vi "Main UI.vi"() -> (3 "CH Name":string[](array[string]))   [LabVIEW 2017]
uses:
  Controls/Load Bank.ctl
  Controls/Available Tests.ctl
  Controls/Graphic Display.ctl
  Controls/Auto Test Display.ctl
  Console Sim/Controls/Console Select.ctl
  Controls/Test TypeDef.ctl
  Code Library/Queue References Array.ctl
  Code Library/Queue Element.ctl
  Controls/Snapshot Typedef.ctl
  Controls/FanMode.ctl
  Controls/LPCA Commands.ctl
  <vilib>/DAQmx/write.llb/DAQmx Write (Analog DBL 1Chan 1Samp).vi
  <vilib>/DAQmx/write.llb/DAQmx Write (Analog Wfm 1Chan NSamp).vi
  <vilib>/DAQmx/write.llb/DAQmx Write (Digital Bool 1Line 1Point).vi
  <vilib>/Utility/config.llb/Read Key (String).vi
  <vilib>/DAQmx/miscellaneous.llb/DAQmx Fill In Error Info.vi
  <vilib>/Utility/config.llb/Write Key (String).vi
  <vilib>/Utility/config.llb/NI_LVConfig.lvlib
  <vilib>/measure/NI_MABase.lvlib
  <resource>/objmgr/daqmx.rc
panel:
  in  "Console Select":T1=enum."SCL Torque"
  in  "Load Config":bool
  in  "Save Config":bool
  in  "SS#":u16
  in  "Snapshot":bool
  in  "Path":path=path "<Data File Path>"
  in  "Test Details":string="<Test Details>"
  out "Test Description":string="<Select Test for a Description>"
  in  "Available Tests":T2
  out "Version":string
  out "Over Temp":bool
  in  "LPCA COM":refnum<visa-resource-name>="COM3"
  in  "Targets":enum32{"Page 1"}(tab)
  in  "Auto Pulse":bool
  in  "Range":i32=2 min=0 max=2 step=1
  in  "Spin":bool
  in  "Load Bank":T3 caption="L/B"
  in  "RPM Target":i32 caption="RPM" min=0 max=250 step=1
  in  "Ibrake":i32=1 caption="MAMP" min=0 max=2500 step=1
  in  "Step Height":i32=2 caption="Ramp" min=1 max=5 step=1
  in  "Thermal Limits":enum32{"Page 1"}(tab)
  in  "S Period":dbl=1.0 min=0.0 max=1440.0 step=0.1 format="%#_g min"
  in  "Thermal Limit":i32=200 min=25 max=250 step=1 format="%.0f degC"
  in  "Thermal Resume":i32=5 min=0 max=250 step=1 format="%.0f degC"
  in  "Stop Time":dbl=60.0 min=1.0 max=1440.0 step=1.0 format="%#_g min"
  in  "Thermal Equilibrium":bool caption="Thermal\nEquilibrium"
  out "Graphic Display":T4
  in  "Data Display":u16(ring) items=["CH.Name", "CH.Name", "CH.Name", "Ibrake", "CH.Name", "CH.Name", "CH.Name", "CH.Name", "CH.Name", "CH.Name", "CH.Name", "CH.Name", "CH.Name", "CH.Name", "Torque", "Ambent", "Brake", "CH.Name", "CH.Name", "CH.Name", "CH.Name", "CH.Name", "CH.Name", "CH.Name", "CH.Name", "CH.Name", "CH.Name"]
  out "Reading Graph":waveform(dbl)(graph)
  out "RPM Graph":cluster{"X":dbl, "Y":dbl}[](graph)
  out "CH Value":dbl[](array[numeric]) format="%.2f"
  in  "Data Setup":i32[](listbox)
  out "RPM":cluster{dbl, dbl}(knob) scale=0.0..300.0
  out "Torque (in-lb)":dbl(knob) scale=-2000.0..2000.0 scale format="%.2f"
  out "Auto Test Controls":T5
  in  "FanMode":bool
  out "Capture":bool
  in  "Stop Test":bool
  in  "Start Test":bool
  in  "Pause Test":bool
  in  "Load Sweep":string
  in  "RPM Sweep":string
  in  "Ibrake Sweep":string
  in  "Sample Frequency":dbl=60.0 min=1.0 max=60.0 step=1.0 format="%.0f S/min"
  in  "Filters":T6(ring)
  out "Sample":bool
  in  "Step Height Sweep":string
  in  "Range Sweep":string
  out "Fan Mode LED Array":bool[](array[boolean])=[FALSE, TRUE, FALSE]
  in  "Save Pulse Data":bool
  in  "Start Pulse":bool
  in  "Pulse Frequency":dbl
  in  "Amplitude":dbl
  in  "Average RPM":dbl
  out "Waveform Graph":waveform(dbl)(graph)
  out "Test Status":string
  out "Test:":string
  out "Time Stamp Control":timestamp format="%<%H:%M:%S  %d/%m/%Y>T"
  # "Targets"
  # "Stop Conditions"
  # "Auto Test Controls"
  # "Swept Targets"
  # "On       Off      Auto"
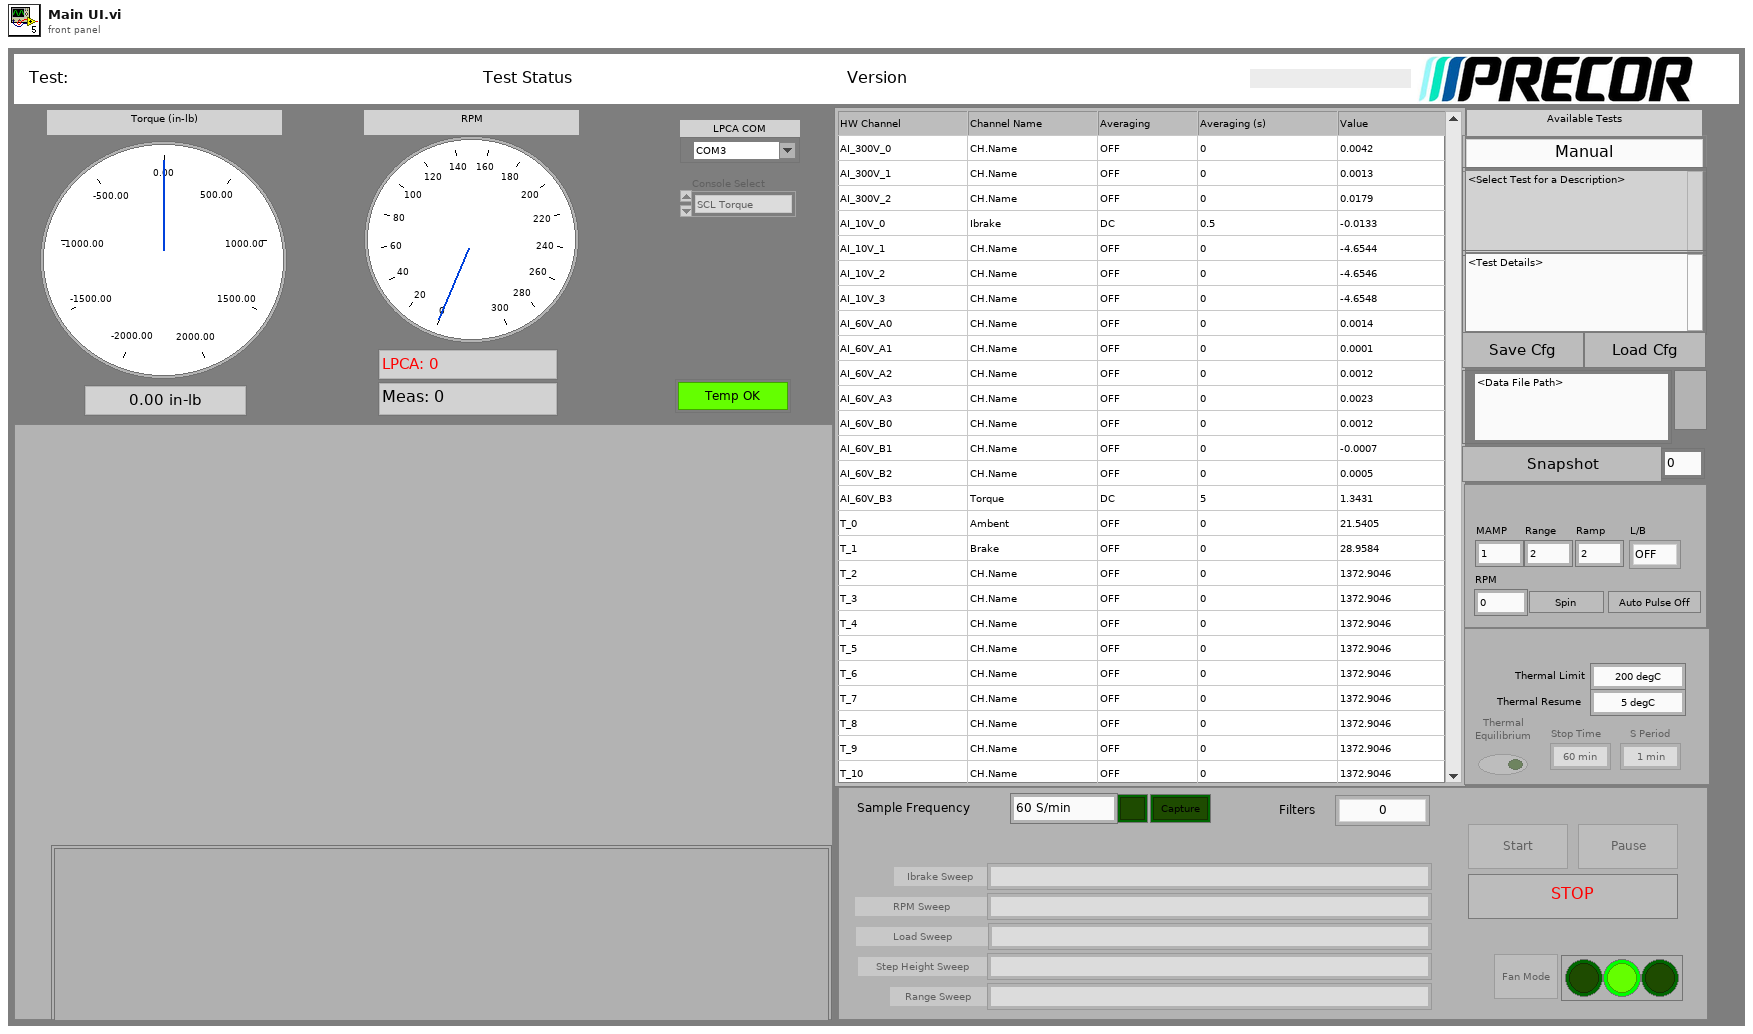
[diagram p1: front panel]
types:
  T1 = typedef "Console Select.ctl" = enum16{"P31 EFX800", "AMT", "SCL Torque"}
  T2 = typedef "Available Tests.ctl" = enum16{"Manual", "EFX Brake Torque", "Generator Torque", "EFX Brake Thermal", "Generator Thermal", "Pulsed RPM", "AMT Brake Torque", "Bike Brake Torque", "AMT Brake Thermal", "Bike Brake Thermal"}
  T3 = typedef "Load Bank.ctl" = enum16{"OFF", "50", "25", "16.7", "12.5", "10.0", "8.3", "7.1", "6.3", "5.6", "5.0", "4.5", "4.2", "3.8", "3.6", "3.3", "3.1"}
  T4 = typedef "Graphic Display.ctl" = enum32{"Analize", "Pulse", "Hidden"}
  T5 = typedef "Auto Test Display.ctl" = enum32{"Sweep Targes", "Pulse", "Hidden"}
  T6 = enum16{"0", "0.1", "0.2", "0.5", "1", "2", "5", "10", "20", "50", "100", "200", "500", "1000", "2000", "5000", "10000"}
  T7 = typedef "Test TypeDef.ctl" = cluster{"Queue Array":T8, "Queue Element":T9, "System Event":refnum<user-event>, "System Event RefNum":refnum<event-registration>, "Queue List":string[], "LPCA COM":refnum<visa-resource-name>, "Rotating":bool, "PrecorAI":refnum<k21>, "T_0 Index":i32, "Bar Graph X":i32[], "Channels":string[], "Active Indicies":i32[], "Active Channels":string[][], "Sample Frequency":dbl, "Ibrake Sweep":string[], "RPM Sweep":string[], "Load Sweep":string[], "Step Height Sweep":string[], "Range Sweep":string[], "A Counter":i32, "B Counter":i32, "C Counter":i32, "#A":i32, "#B":i32, "#C":i32, "Current RPM":dbl, "Current Ibrake":u32, "Current Range":u32, "Current Step Height":u32, "Load Bank":T3, "Cfg Cntrls":refnum<vi>[], "T_Monitor Indices":i32[], "Thermal Limit":i32, "Thermal Resume":i32, "Timer Reset":bool, "Stop Time":dbl, "Autotest":bool, "Pulsed RPM Capture":bool, "Get Sample":bool, "Last State":string, "Reset Timeout":bool, "Ctrl Refs":cluster{"Test Details":refnum<vi>, "Save Config":refnum<vi>, "Load Config":refnum<vi>, "Path":refnum<vi>, "Snapshot":refnum<vi>, "SS#":refnum<vi>, "Ibrake":refnum<vi>, "RPM Target":refnum<vi>, "Spin":refnum<vi>, "Load Bank":refnum<vi>, "Start Test":refnum<vi>, "Pause Test":refnum<vi>, "Load Sweep":refnum<vi>, "RPM Sweep":refnum<vi>, "Ibrake Sweep":refnum<vi>, "Filters":refnum<vi>, "Sample Frequency":refnum<vi>, "Data Setup":refnum<vi>, "Pause":refnum<vi>, "Stop Time":refnum<vi>, "S Period":refnum<vi>, "Range":refnum<vi>, "Step Height":refnum<vi>, "Step Height Sweep":refnum<vi>, "Range Sweep":refnum<vi>, "Available Tests":refnum<vi>, "RPM Graph":refnum<vi>, "RPM Knob":refnum<vi>, "FanMode":refnum<vi>, "Fan Mode LED Array":refnum<vi>, "Thermal Equilibrium":refnum<vi>, "Data Display":refnum<vi>, "LPCA Error":refnum<vi>, "LPCA Ramp":refnum<vi>, "LPCA Range":refnum<vi>, "LPCA Resistance":refnum<vi>, "Analyze Read":refnum<vi>, "Console Select":refnum<vi>, "Sub Panel":refnum<vi>}, "Pulse Waveform":waveform(dbl), "Snapshot":T10, "Sample Period":dbl, "OverTemp":bool, "Available Tests":T2, "FanMode":T11, "Fan Mode LED Array":bool[], "Thermal\nEquilibrium ":bool, "Equilibrium Stop":bool, "AvgDegChg":dbl[]}
  T8 = typedef "Queue References Array.ctl" = refnum<queue>[]
  T9 = typedef "Queue Element.ctl" = cluster{"state":string, "data":variant}
  T10 = typedef "Snapshot Typedef.ctl" = cluster{"Test Details":string, "Version":string, "Date":timestamp, "Selected Test":string, "Snapshot Number":u16, "Time":timestamp, "Ibrake Setpoint":string, "RPM Setpoint":string, "Range Setpoint":string, "Step Height Setpoint":string, "Load Bank Setpoint":string, "Measurement Headers":string, "Measurements":string, "A":i32, "B":i32, "C":i32, "Raw Data":string[][], "Available Tests":T2, "Ibrake List":string, "RPM List":string, "Load Bank List":string, "Range List":string, "Step Height List":string, "FanMode Setpoint":T11}
  T11 = typedef "FanMode.ctl" = enum16{"On", "Off", "Auto"}
  T12 = cluster{"Test Details":refnum<vi>, "Save Config":refnum<vi>, "Load Config":refnum<vi>, "Path":refnum<vi>, "Snapshot":refnum<vi>, "SS#":refnum<vi>, "Ibrake":refnum<vi>, "RPM Target":refnum<vi>, "Spin":refnum<vi>, "Load Bank":refnum<vi>, "Start Test":refnum<vi>, "Pause Test":refnum<vi>, "Load Sweep":refnum<vi>, "RPM Sweep":refnum<vi>, "Ibrake Sweep":refnum<vi>, "Filters":refnum<vi>, "Sample Frequency":refnum<vi>, "Data Setup":refnum<vi>, "Pause":refnum<vi>, "Stop Time":refnum<vi>, "S Period":refnum<vi>, "Range":refnum<vi>, "Step Height":refnum<vi>, "Step Height Sweep":refnum<vi>, "Range Sweep":refnum<vi>, "Available Tests":refnum<vi>, "RPM Graph":refnum<vi>, "RPM Knob":refnum<vi>, "FanMode":refnum<vi>, "Fan Mode LED Array":refnum<vi>, "Thermal Equilibrium":refnum<vi>, "Data Display":refnum<vi>, "LPCA Error":refnum<vi>, "LPCA Ramp":refnum<vi>, "LPCA Range":refnum<vi>, "LPCA Resistance":refnum<vi>, "Analyze Read":refnum<vi>, "Console Select":refnum<vi>, "Sub Panel":refnum<vi>}
  T13 = typedef "lveventtype.ctl" = enum32{"Null", "Timeout", "Annotation Menu Selection", "Annotation Menu Selection?", "App Instance Close", "App Instance Close?", "Autoscale Range Change", "Bookmark Info Change", "Cell Edit", "Cell Edit?", "Cursor Grab", "Cursor Grab?", "Cursor Menu Selection", "Cursor Menu Selection?", "Cursor Move", "Cursor Release", "Data Change", "Direction Change", "Display State Change", "Drag Ended", "Drag Enter", "Drag Leave", "Drag Over", "Drag Source Update", "Drag Starting", "Drag Starting?", "Drop", "Exec State Change", "Key Down", "Key Down?", "Key Repeat", "Key Repeat?", "Key Up", "Listbox Double Click", "Menu Activation?", "Menu Selection (App)", "Menu Selection? (App)", "Menu Selection (User)", "Mouse Down", "Mouse Down?", "Mouse Enter", "Mouse Leave", "Mouse Move", "Mouse Up", "Mouse Wheel", "NI Security User Change (App)", "Pane Size", "Panel Close", "Panel Close?", "Panel Resize", "Plot Attribute Change", "Scale Range Change", "Shortcut Menu Activation?", "Shortcut Menu Selection (App)", "Shortcut Menu Selection? (App)", "Shortcut Menu Selection (User)", "Tree Double Click", "Tree Drag", "Tree Drag?", "Tree Drop", "Tree Drop?", "Tree Item Close", "Tree Item Close?", "Tree Item Open", "Tree Item Open?", "User Event", "Value Change"}
  T14 = typedef "LVPoint32TypeDef.ctl" = cluster{"Horizontal":i32, "Vertical":i32}
  T15 = typedef "LVRowAndColumnTypeDef.ctl" = cluster{"Row":i32, "Column":i32}
  T16 = cluster{"Label.Text":string, "selected path":path}
  T17 = cluster{"ItemTag":string, "Row":i32, "Column":i32}
  T18 = cluster{"String":string, "Row":i32, "Column":i32}
  T19 = typedef "NI_LVConfig.lvlib/Config Data RefNum.ctl" = refnum<k1>
  T20 = typedef "LPCA Commands.ctl" = enum16{"RSET", "stop", "rpmh", "rpml", "prpm", "rpm", "mamp", "rng", "tmp1", "tmp2", "err", "ramp"}
  T21 = enum16{"Init", "Get", "Set Step Counter", "Insert Command", "Insert Now Command"}
  T22 = cluster{"A Counter":i32, "B Counter":i32, "C Counter":i32}
  T23 = cluster{"ItemNames":string[][], "ItemSyms":i32[]}
  T24 = enum8{"Enabled", "Disabled", "Disabled and Grayed Out"}
  T25 = cluster{"A Counter":i32, "B Counter":i32, "B Counter 2":i32}
  T26 = cluster{"seconds since 1Jan1904":timestamp, "SS#":u16, "Snapshot":bool}
  T27 = cluster{"Sample Acquired":bool, "Torque":dbl, "Temperatre Plot Data":cluster{dbl[], i32[]}[], "Temperature Avg":dbl[], "Samples":i32}
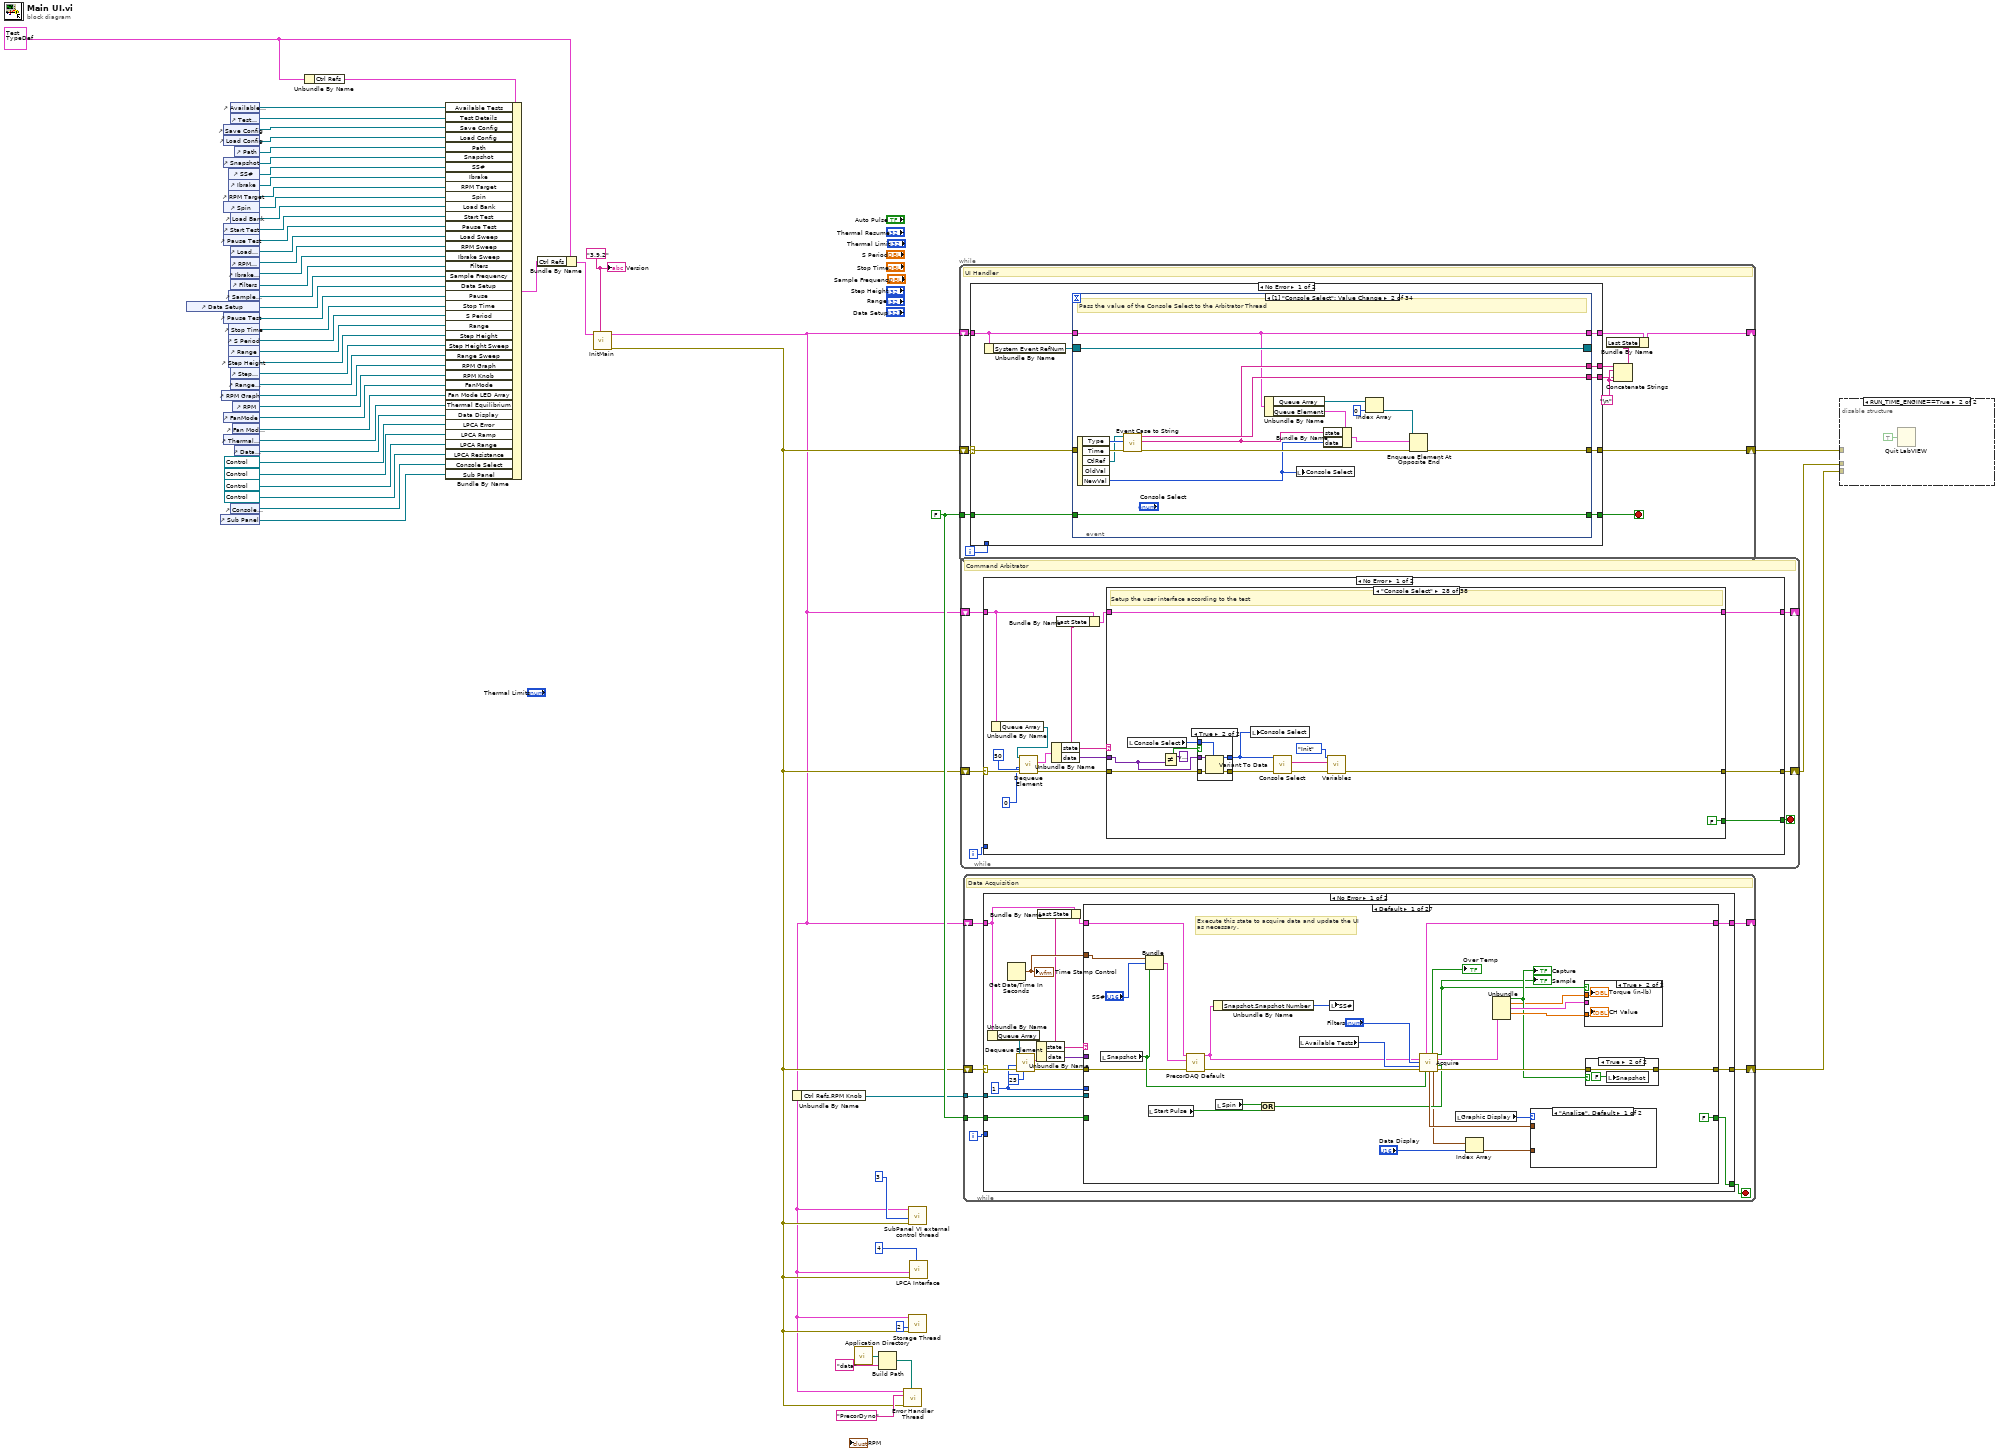
[diagram p0: block diagram]
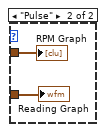
[diagram p3: hidden frame]
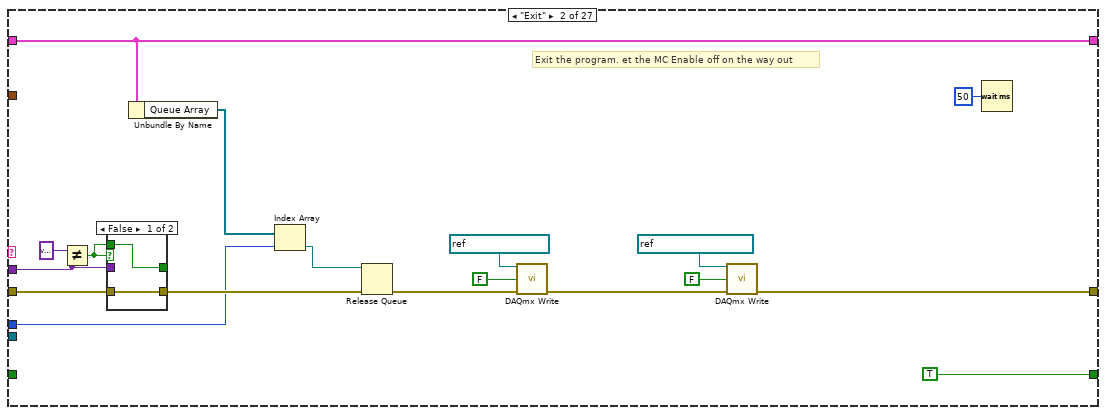
[diagram p5: hidden frame]
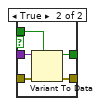
[diagram p6: hidden frame]
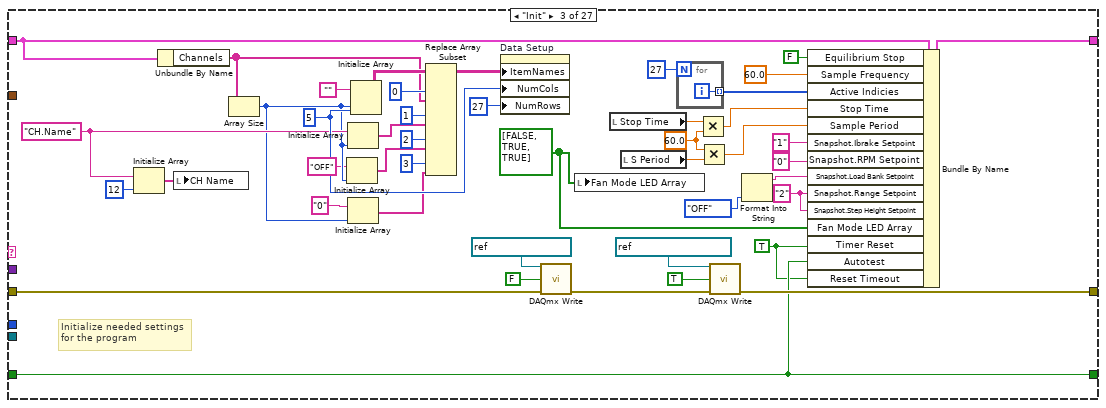
[diagram p7: hidden frame]
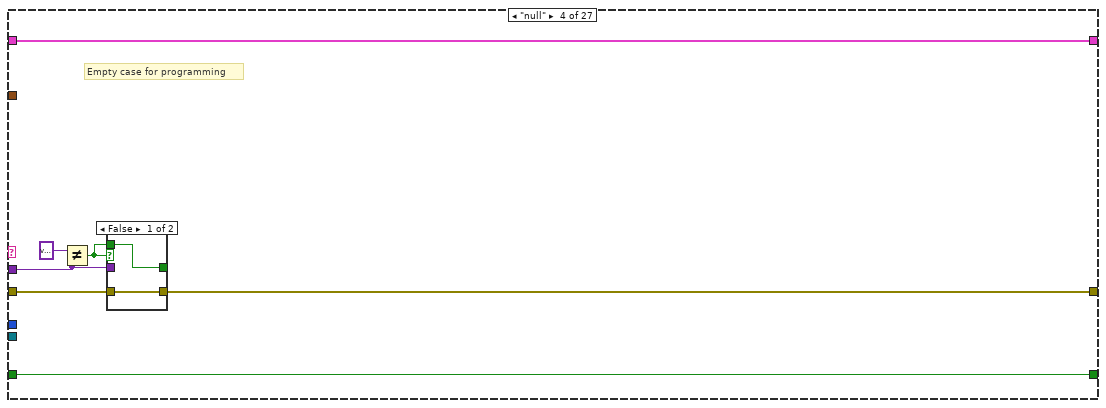
[diagram p8: hidden frame]
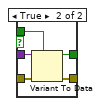
[diagram p9: hidden frame]
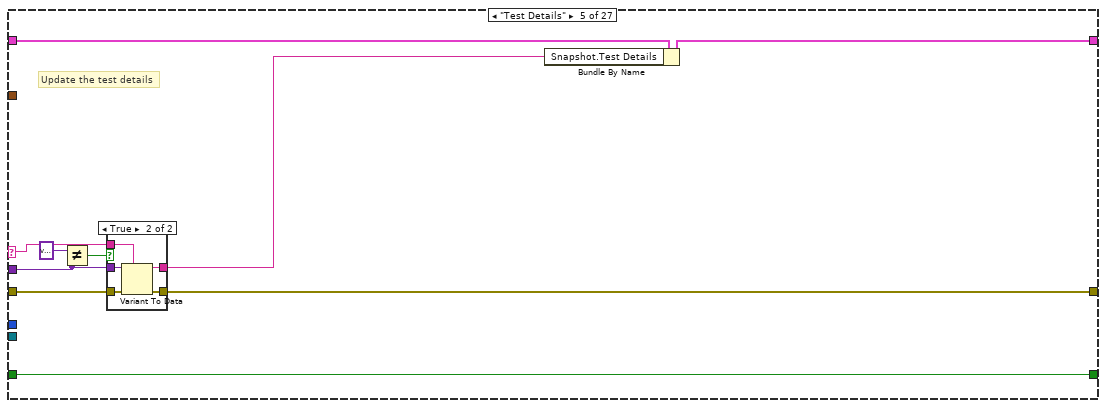
[diagram p10: hidden frame]
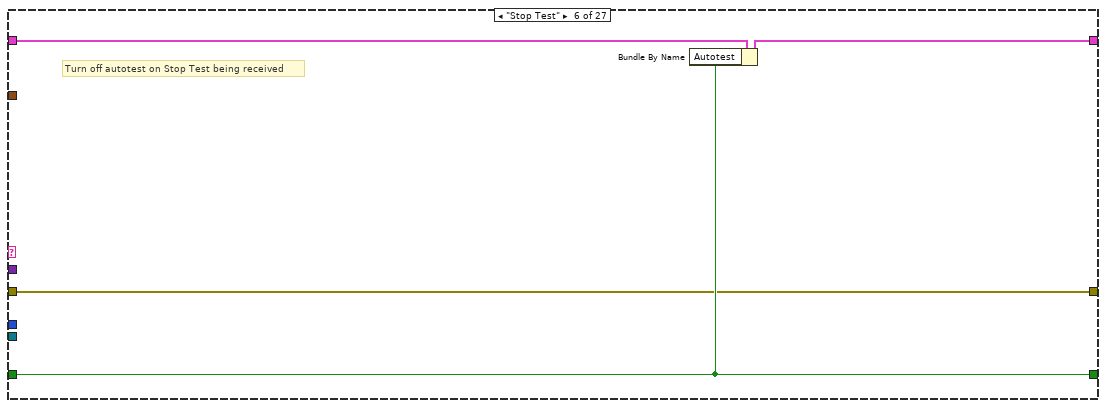
[diagram p12: hidden frame]
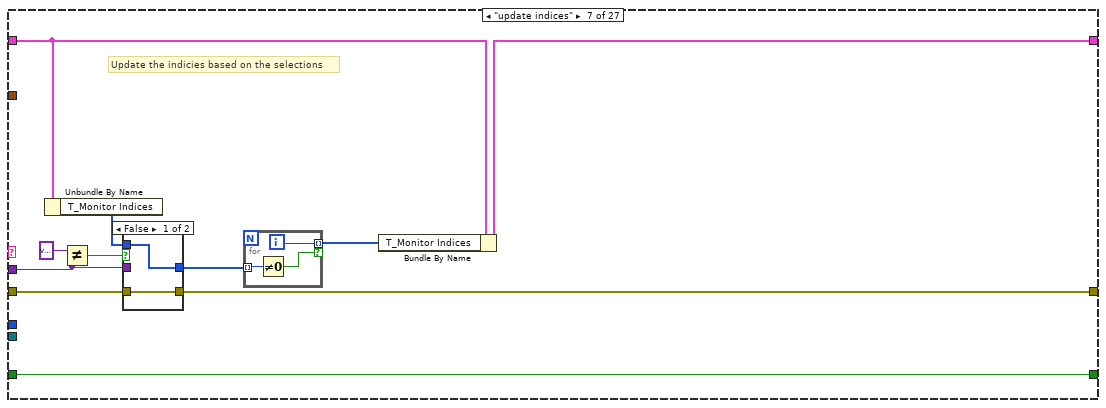
[diagram p13: hidden frame]
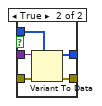
[diagram p14: hidden frame]
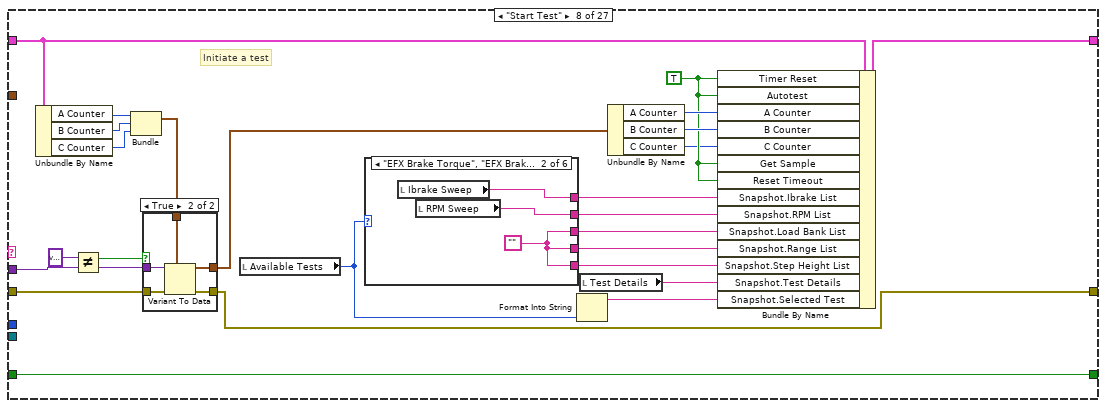
[diagram p15: hidden frame]
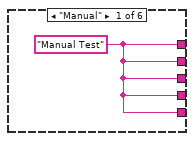
[diagram p16: hidden frame]
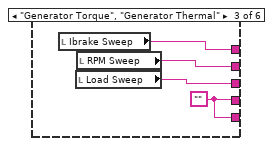
[diagram p17: hidden frame]
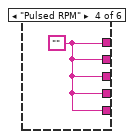
[diagram p18: hidden frame]
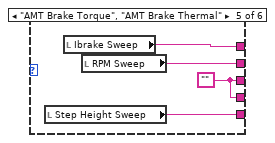
[diagram p19: hidden frame]
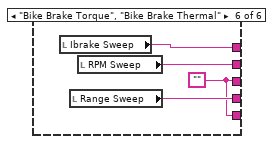
[diagram p20: hidden frame]
diagram:
  w21 = "3.9.2" ("Version")
  w3 = T7 {"Queue Array"=[], "Queue Element"={"state"="", "data"=variant}, "System Event"=refnum, "System Event RefNum"=refnum, "Queue List"=[], "LPCA COM"="", "Rotating"=FALSE, "PrecorAI"="", "T_0 Index"=0, "Bar Graph X"=[], "Channels"=[], "Active Indicies"=[], "Active Channels"=[], "Sample Frequency"=0.0, "Ibrake Sweep"=[], "RPM Sweep"=[], "Load Sweep"=[], "Step Height Sweep"=[], "Range Sweep"=[], "A Counter"=0, "B Counter"=0, "C Counter"=0, "#A"=0, "#B"=0, "#C"=0, "Current RPM"=0.0, "Current Ibrake"=0, "Current Range"=0, "Current Step Height"=0, "Load Bank"=enum."OFF", "Cfg Cntrls"=[], "T_Monitor Indices"=[], "Thermal Limit"=0, "Thermal Resume"=0, "Timer Reset"=FALSE, "Stop Time"=0.0, "Autotest"=FALSE, "Pulsed RPM Capture"=FALSE, "Get Sample"=FALSE, "Last State"="", "Reset Timeout"=FALSE, "Ctrl Refs"={"Test Details"=refnum, "Save Config"=refnum, "Load Config"=refnum, "Path"=refnum, "Snapshot"=refnum, "SS#"=refnum, "Ibrake"=refnum, "RPM Target"=refnum, "Spin"=refnum, "Load Bank"=refnum, "Start Test"=refnum, "Pause Test"=refnum, "Load Sweep"=refnum, "RPM Sweep"=refnum, "Ibrake Sweep"=refnum, "Filters"=refnum, "Sample Frequency"=refnum, "Data Setup"=refnum, "Pause"=refnum, "Stop Time"=refnum, "S Period"=refnum, "Range"=refnum, "Step Height"=refnum, "Step Height Sweep"=refnum, "Range Sweep"=refnum, "Available Tests"=refnum, "RPM Graph"=refnum, "RPM Knob"=refnum, "FanMode"=refnum, "Fan Mode LED Array"=refnum, "Thermal Equilibrium"=refnum, "Data Display"=refnum, "LPCA Error"=refnum, "LPCA Ramp"=refnum, "LPCA Range"=refnum, "LPCA Resistance"=refnum, "Analyze Read"=refnum, "Console Select"=refnum, "Sub Panel"=refnum}, "Pulse Waveform"={"t0"=timestamp(0 s since 1904-01-01), "dt"=1.0, "Y"=[]}, "Snapshot"={"Test Details"="", "Version"="", "Date"=timestamp(0 s since 1904-01-01), "Selected Test"="", "Snapshot Number"=0, "Time"=timestamp(0 s since 1904-01-01), "Ibrake Setpoint"="", "RPM Setpoint"="", "Range Setpoint"="", "Step Height Setpoint"="", "Load Bank Setpoint"="", "Measurement Headers"="", "Measurements"="", "A"=0, "B"=0, "C"=0, "Raw Data"=[], "Available Tests"=enum."Manual", "Ibrake List"="", "RPM List"="", "Load Bank List"="", "Range List"="", "Step Height List"="", "FanMode Setpoint"=enum."On"}, "Sample Period"=0.0, "OverTemp"=FALSE, "Available Tests"=enum."Manual", "FanMode"=enum."On", "Fan Mode LED Array"=[], "Thermal\nEquilibrium "=FALSE, "Equilibrium Stop"=FALSE, "AvgDegChg"=[]}
  w55 = FALSE
  n1 = control-ref of="Data Setup"() -> (w31:refnum<vi>)
  n2 = control-ref of="Sub Panel"() -> (w6:refnum<vi>)
  n3 = control-ref of="RPM Graph"() -> (w20:refnum<vi>)
  n4 = control-ref of="Save Config"() -> (w48:refnum<vi>)
  n5 = control-ref of="Load Config"() -> (w47:refnum<vi>)
  n6 = control-ref of="Snapshot"() -> (w45:refnum<vi>)
  n7 = control-ref of="Spin"() -> (w41:refnum<vi>)
  n8 = control-ref of="Start Test"() -> (w39:refnum<vi>)
  n9 = control-ref of="Pause Test"() -> (w38:refnum<vi>)
  n10 = control-ref of="Pause Test"() -> (w30:refnum<vi>)
  n11 = control-ref of="FanMode"() -> (w17:refnum<vi>)
  n12 = control-ref of="Thermal Equilibrium"() -> (w15:refnum<vi>)
  n13 = control-ref of="SS#"() -> (w44:refnum<vi>)
  n14 = control-ref of="Ibrake"() -> (w43:refnum<vi>)
  n15 = control-ref of="RPM Target"() -> (w42:refnum<vi>)
  n16 = control-ref of="Sample Frequency"() -> (w32:refnum<vi>)
  n17 = control-ref of="Stop Time"() -> (w29:refnum<vi>)
  n18 = control-ref of="S Period"() -> (w28:refnum<vi>)
  n19 = control-ref of="Range"() -> (w27:refnum<vi>)
  n20 = control-ref of="Step Height"() -> (w26:refnum<vi>)
  n21 = control-ref of="Available Tests"() -> (w23:refnum<vi>)
  n22 = control-ref of="Test Details"() -> (w49:refnum<vi>)
  n23 = control-ref of="Load Bank"() -> (w40:refnum<vi>)
  n24 = control-ref of="Load Sweep"() -> (w36:refnum<vi>)
  n25 = control-ref of="RPM Sweep"() -> (w35:refnum<vi>)
  n26 = control-ref of="Ibrake Sweep"() -> (w34:refnum<vi>)
  n27 = control-ref of="Filters"() -> (w33:refnum<vi>)
  n28 = control-ref of="Step Height Sweep"() -> (w25:refnum<vi>)
  n29 = control-ref of="Range Sweep"() -> (w24:refnum<vi>)
  n30 = control-ref of="Console Select"() -> (w1:refnum<vi>)
  n31 = control-ref of="RPM"() -> (w19:refnum<vi>)
  n32 = control-ref of="Fan Mode LED Array"() -> (w16:refnum<vi>)
  n33 = control-ref of="Path"() -> (w46:refnum<vi>)
  n34 = control-ref of="Data Display"() -> (w14:refnum<vi>)
  n35 = Unbundle By Name(w3) -> ("Ctrl Refs"=w37:T12)
  n36 = Bundle By Name(cluster=w37, "Available Tests"=w23, "Test Details"=w49, "Save Config"=w48, "Load Config"=w47, "Path"=w46, "Snapshot"=w45, "SS#"=w44, "Ibrake"=w43, "RPM Target"=w42, "Spin"=w41, "Load Bank"=w40, "Start Test"=w39, "Pause Test"=w38, "Load Sweep"=w36, "RPM Sweep"=w35, "Ibrake Sweep"=w34, "Filters"=w33, "Sample Frequency"=w32, "Data Setup"=w31, "Pause"=w30, "Stop Time"=w29, "S Period"=w28, "Range"=w27, "Step Height"=w26, "Step Height Sweep"=w25, "Range Sweep"=w24, "RPM Graph"=w20, "RPM Knob"=w19, "FanMode"=w17, "Fan Mode LED Array"=w16, "Thermal Equilibrium"=w15, "Data Display"=w14, "LPCA Error"=refnum<vi> refnum, "LPCA Ramp"=refnum<vi> refnum, "LPCA Range"=refnum<vi> refnum, "LPCA Resistance"=refnum<vi> refnum, "Console Select"=w1, "Sub Panel"=w6) -> (w22:T12)
  n37 = Bundle By Name(cluster=w3, "Ctrl Refs"=w22) -> (w4:T7)
  n38 = call "InitMain.vi"("Version"=w21, "Cluster In"=w4) -> ("error out"=w5:errorcluster, "Cluster Out"=w2:T7)  [unwired: 8 in]
  n39 = Unbundle By Name(w2) -> ("Ctrl Refs.RPM Knob"=w18:refnum<vi>)
  n40 = call <vilib>:"Application Directory.vi"() -> ("Application Directory"=w13:path)
  n41 = Build Path(base path=w13, name or relative path="data") -> (appended path=w11:path)
  n42 = call "Error Handler Thread.vi"("Data Path"=w11, "error in (no error)"=w5, "File Name"="PrecorDyno", "Cluster"=w2) -> ()  [unwired: 8 in]
  n43 = call "SubPanel VI external control thread.vi"("error in (no error)"=w5, "index"=3, "Control Data"=w2) -> ()  [unwired: 9 in]
  n44 = call "Storage Thread.vi"("error in (no error)"=w5, "index"=2, "Control Data"=w2) -> ()  [unwired: 9 in]
  n45 = call "LPCA Interface.vi"("index"=4, "error in (no error)"=w5, "Cluster"=w2) -> ()  [unwired: 9 in]
  n46 = while {
    shift-right: [w68] -> w57
    shift-left: w5 -> [w69]
    tunnel: w55 -> [w66]
    shift-right: [w63] -> _
    shift-left: w2 -> [w64]
    i -> [w58]
    stop <- w67 stop-if-true
    w62 = "\n"
    # "UI Handler"
    n47 = case shown="No Error" w69 {
      selector: w69 -> [w74 w937]
      tunnel: [w78 w936] -> w68
      tunnel: [w77 w939] -> w67
      tunnel: w66 -> [w76 w939]
      tunnel: [w75 w935] -> w65
      tunnel: w64 -> [w73 w935]
      tunnel: [w71 _] -> w61
      tunnel: [w70 _] -> w60
      tunnel: w58 -> [_ _]
      frame No Error {
        n48 = Unbundle By Name(w73) -> ("System Event RefNum"=w72:refnum<event-registration>)
        n49 = event shown="[1] \"Console Select\": Value Change" {
          selector: w72 -> [w81 w99 w114 w128 w143 w160 w216 w256 w283 w310 w331 w351 w370 w425 w448 w471 w494 w519 w541 w567 w594 w623 w652 w664 w694 w725 w755 w785 w815 w845 w865 w880 w889 w923]
          dyn-events: [w81 w99 w114 w128 w143 w160 w216 w256 w283 w310 w331 w351 w370 w425 w448 w471 w494 w519 w541 w567 w594 w623 w652 w664 w694 w725 w755 w785 w815 w845 w865 w880 w890 w923] -> _
          timeout: _ -> [_ _ _ _ _ _ _ _ _ _ _ _ _ _ _ _ _ _ _ _ _ _ _ _ _ _ _ _ _ _ _ _ _ _]
          tunnel: w74 -> [w85 w101 w117 w131 w146 w162 w218 w258 w286 w313 w334 w353 w372 w427 w450 w473 w496 w521 w543 w569 w596 w625 w654 w666 w696 w726 w756 w786 w816 w846 w856 w872 w894 w926]
          tunnel: [w82 w90 w112 w125 w141 w153 w207 w250 w273 w305 w327 w349 w369 w410 w444 w467 w490 w515 w537 w563 w590 w604 w634 w660 w689 w719 w749 w779 w809 w839 w862 w877 w888 w921] -> w78
          tunnel: [w86 w102 w118 w132 w147 w163 w219 w259 w274 w314 w335 w354 w358 w428 w451 w474 w497 w522 w544 w570 w597 w626 w655 w667 w697 w727 w757 w787 w817 w847 w866 w881 w886 w919] -> w77
          tunnel: w76 -> [w86 w102 w118 w132 w147 w163 w219 w259 w274 w314 w335 w354 w358 w428 w451 w474 w497 w522 w544 w570 w597 w626 w655 w667 w697 w727 w757 w787 w817 w847 w866 w881 w885 w919]
          tunnel: [w83 w88 w111 w124 w140 w148 w206 w249 w282 w308 w326 w348 w367 w406 w447 w470 w493 w518 w540 w566 w593 w611 w635 w662 w692 w723 w753 w783 w813 w843 w855 w871 w892 w922] -> w75
          tunnel: w73 -> [w83 w88 w111 w124 w140 w148 w206 w249 w282 w308 w326 w348 w367 w406 w447 w470 w493 w518 w540 w566 w593 w609 w636 w662 w692 w723 w753 w783 w813 w843 w855 w871 w891 w922]
          tunnel: [w80 w89 w105 w119 w134 w149 w209 w244 w271 w287 w315 w336 w356 w392 w429 w452 w475 w500 w523 w545 w571 w598 w627 w658 w682 w698 w728 w758 w788 w818 w848 w867 w882 w913] -> w71
          tunnel: [w79 w98 w113 w127 w133 w150 w208 w243 w272 w288 w315 w336 w355 w392 w429 w452 w475 w500 w523 w545 w571 w598 w627 w657 w682 w698 w728 w758 w788 w818 w848 w867 w882 w913] -> w70
          event Timeout {
            # "Generally, a default case for use as a template"
            n50 = event-data() -> ("Type"=w84:T13)  [unwired: 1 in]
            n51 = call "Event Case to String.vi"("error in (no error)"=w85, "Type"=w84) -> ("error out"=w82:errorcluster, "Label.Text"=w80:string, "Diagnostic String"=w79:string)  [unwired: 7 in]
          }
          event Value Change {
            # "Pass the value of the Console Select to the Arbitrator Thread"
            n52 = event-data() -> ("Type"=w100:T13, "CtlRef"=w97:refnum<vi>, "NewVal"=w87:T1)  [unwired: 1 in, 2 out]
            n53 = call "Event Case to String.vi"("error in (no error)"=w101, "Type"=w100, "Control In"=w97) -> ("error out"=w91:errorcluster, "Label.Text"=w89:string, "Diagnostic String"=w98:string)  [unwired: 6 in]
            n54 = Unbundle By Name(w88) -> ("Queue Array"=w96:T8, "Queue Element"=w93:T9)
            n55 = local write "Console Select"(w87) -> ()
            n56 = Bundle By Name(cluster=w93, "state"=w89, "data"=w87) -> (w92:T9)
            n57 = Index Array(array=w96, index=0) -> (element=w95:refnum<queue>)
            n58 = Enqueue Element At Opposite End(queue=w95, element=w92, error in (no error)=w91) -> (error out=w90:errorcluster)  [unwired: 1 in, 2 out]
          }
          event "Test Details": Value Change {
            # "Passes the contents of Test Details to the acquisition thread."
            n59 = event-data() -> ("CtlRef"=w103:refnum<vi>, "Type"=w116:T13, "NewVal"=w104:string)  [unwired: 1 in]
            n60 = call "Event Case to String.vi"("error in (no error)"=w117, "Type"=w116, "Control In"=w103) -> ("error out"=w115:errorcluster, "Label.Text"=w105:string, "Diagnostic String"=w113:string)  [unwired: 6 in]
            n61 = Unbundle By Name(w111) -> ("Queue Array"=w110:T8, "Queue Element"=w107:T9)
            n62 = Bundle By Name(cluster=w107, "state"=w105, "data"=w104) -> (w106:T9)
            n63 = Index Array(array=w110, index=1) -> (element=w109:refnum<queue>)
            n64 = Enqueue Element At Opposite End(queue=w109, element=w106, error in (no error)=w115) -> (error out=w112:errorcluster)  [unwired: 1 in, 2 out]
          }
          event "Average RPM", "Amplitude", "Pulse Frequency": Value Change {
            # "Fires the appropriate case of the Command Arbitrator"
            n65 = event-data() -> ("CtlRef"=w126:refnum<vi>, "Type"=w130:T13)  [unwired: 1 in]
            n66 = call "Event Case to String.vi"("error in (no error)"=w131, "Type"=w130, "Control In"=w126) -> ("error out"=w129:errorcluster, "Label.Text"=w119:string, "Diagnostic String"=w127:string)  [unwired: 6 in]
            n67 = Unbundle By Name(w124) -> ("Queue Array"=w123:T8, "Queue Element"=w121:T9)
            n68 = Bundle By Name(cluster=w121, "state"=w119) -> (w120:T9)
            n69 = Index Array(array=w123) -> (element=w122:refnum<queue>)  [unwired: 1 in]
            n70 = Enqueue Element At Opposite End(queue=w122, element=w120, error in (no error)=w129) -> (error out=w125:errorcluster)  [unwired: 1 in, 2 out]
          }
          event "LPCA COM": Value Change {
            # "Passes the selcted COM port to the LPCA thread."
            n71 = event-data() -> ("NewVal"=w135:refnum<visa-resource-name>, "CtlRef"=w142:refnum<vi>, "Type"=w145:T13)  [unwired: 1 in]
            n72 = call "Event Case to String.vi"("error in (no error)"=w146, "Type"=w145, "Control In"=w142) -> ("error out"=w144:errorcluster, "Label.Text"=w134:string, "Diagnostic String"=w133:string)  [unwired: 6 in]
            n73 = Unbundle By Name(w140) -> ("Queue Array"=w139:T8)
            n74 = Index Array(array=w139) -> (element=w138:refnum<queue>)  [unwired: 1 in]
            n75 = Bundle By Name(cluster=T9 {"state"="init LPCA", "data"=variant} ("element"), "data"=w135) -> (w136:T9)
            n76 = Enqueue Element(queue=w138, element=w136, error in (no error)=w144) -> (error out=w141:errorcluster)  [unwired: 1 in, 2 out]
          }
          event "Snapshot": Mouse Down? {
            # "Fires the case to acquire a data snapshot."
            n77 = event-data() -> ("CtlRef"=w159:refnum<vi>, "Type"=w161:T13)  [unwired: 1 in]
            n78 = call "Event Case to String.vi"("error in (no error)"=w162, "Type"=w161, "Control In"=w159) -> ("error out"=w154:errorcluster, "Label.Text"=w149:string, "Diagnostic String"=w150:string)  [unwired: 6 in]
            n79 = local read "Path"() -> (w157:path)
            n80 = Equal?(x=w157, y=path "<Data File Path>" ("Path")) -> (x = y?=w155:bool)
            n81 = Not A Number/Path/Refnum?(number/path/refnum=w157) -> (NaN/Path/Refnum?=w156:bool)
            n82 = Or(x=w156, y=w155) -> (x .or. y?=w151:bool)
            n83 = case shown="True" w151 {
              selector: w151 -> [w164 _]
              tunnel: w154 -> [w165 w174]
              tunnel: [w165 w169] -> w153
              tunnel: [w164 w167] -> w152
              tunnel: w148 -> [_ w171]
              frame False {
              }
              frame True {
                n84 = call "File Dialog2"("prompt"="Please Select a Storage File", "error in"=w174, "pattern (all files)"="*.csv") -> ("selected path"=w172:path, "cancelled"=w168:bool, "error out"=w170:errorcluster)  [unwired: 9 in, 1 out]
                n85 = case shown="False" w168 {
                  selector: w168 -> [w175 w197]
                  tunnel: w172 -> [w179 _]
                  tunnel: w171 -> [w178 _]
                  tunnel: w170 -> [w177 w198]
                  tunnel: [w176 w198] -> w169
                  tunnel: [w175 w197] -> w167
                  frame False {
                    n86 = local write "Path"(w179) -> ()
                    n87 = Strip Path(path=w179) -> (stripped path=w182:path, name=w186:string)
                    n88 = Match Pattern(string=w186, regular expression="\\.") -> (before substring=w184:string, after substring=w189:string)  [unwired: 1 in, 2 out]
                    n89 = Concatenate Strings(w184, ".csv" ("y")) -> (w183:string)
                    n90 = Equal?(x=w189, y="csv") -> (x = y?=w187:bool)
                    n91 = Build Path(base path=w182, name or relative path=w183) -> (appended path=w181:path)
                    n92 = Select(t=w179, s=w187, f=w181) -> (s? t:f=w180:path)
                    n93 = Unbundle By Name(w178) -> ("Queue Array"=w196:T8)
                    n94 = To Variant(anything=w180) -> (Variant=w191:variant)
                    n95 = local write "Path"(w180) -> ()
                    n96 = Bundle By Name(cluster=T9 {"state"="New File", "data"=variant} ("element"), "data"=w191) -> (w192:T9)
                    n97 = Index Array(array=w196, index=2) -> (element=w194:refnum<queue>)
                    n98 = Enqueue Element(queue=w194, element=w192, error in (no error)=w177) -> (error out=w176:errorcluster)  [unwired: 1 in, 2 out]
                  }
                  frame True {
                  }
                }
              }
            }
            n99 = event-data("Discard?"=w152) -> ()  [unwired: 1 in, 1 out]
          }
          event "Data Setup": Mouse Down {
            # "Modify the symbol of the selected row"
            n100 = event-data() -> ("CtlRef"=w215:refnum<vi>, "Type"=w217:T13, "Coords"=w210:T14)  [unwired: 1 in]
            n101 = call "Event Case to String.vi"("error in (no error)"=w218, "Type"=w217, "Control In"=w215) -> ("error out"=w214:errorcluster, "Label.Text"=w209:string, "Diagnostic String"=w208:string)  [unwired: 6 in]
            n102 = invoke class="MCListbox (strict)" method="Point To Row Column"(reference=w215, error in=w214, "Point"=w210) -> (reference out=w211:refnum<vi>, error out=w212:errorcluster, "CellPosition"=w203:T15, "InGlyph"=w213:bool)  [unwired: 4 in, 3 out]
            n103 = Unbundle By Name(w206) -> ("Queue Array"=w205:T8, "Queue Element"=w204:T9, "T_0 Index"=w201:i32)
            n104 = Unbundle By Name(w203) -> ("Row"=w202:i32)
            n105 = Greater Or Equal?(x=w202, y=w201) -> (x >= y?=w199:bool)
            n106 = Compound Arithmetic op=AND(w199, w213) -> (w200:bool)
            n107 = case shown="True" w200 {
              tunnel: w212 -> [w220 w239]
              tunnel: w211 -> [_ w240]
              tunnel: [w220 w221] -> w207
              tunnel: w205 -> [_ w232]
              tunnel: w204 -> [_ w229]
              tunnel: w202 -> [_ w226]
              frame False {
              }
              frame True {
                n108 = property class="MCListbox (strict)"(reference=w240, error in=w239) -> (reference out=w237:refnum<vi>, error out=w238:errorcluster, "ItemSyms"=w234:i32[])
                n109 = Index Array(array=w234, index=w226) -> (element=w236:i32)
                n110 = case shown="1" w236 {
                  tunnel: [1 0] -> w235
                  frame 0, Default {
                  }
                  frame 1 {
                  }
                }
                n111 = Replace Array Subset(array=w234, new element=w235, index=w226) -> (w227:i32[])
                n112 = Bundle By Name(cluster=w229, "state"="update indices", "data"=w227) -> (w222:T9)
                n113 = Index Array(array=w232, index #1=0 ("index"), index #2=1 ("index")) -> (element #1=w223:refnum<queue>, element #2=w231:refnum<queue>)
                n114 = property class="MCListbox (strict)"(reference=w237, error in=w238, "ItemSyms"=w227) -> (error out=w233:errorcluster)  [unwired: 1 out]
                n115 = Enqueue Element At Opposite End(queue=w231, element=w222, error in (no error)=w233) -> (error out=w224:errorcluster)  [unwired: 1 in, 2 out]
                n116 = Enqueue Element At Opposite End(queue=w223, element=w222, error in (no error)=w224) -> (error out=w221:errorcluster)  [unwired: 1 in, 2 out]
              }
            }
          }
          event "Save Config", "Load Config": Mouse Up {
            # "Save or load a selected configuration"
            n117 = event-data() -> ("CtlRef"=w255:refnum<vi>, "Type"=w257:T13)  [unwired: 1 in]
            n118 = call "Event Case to String.vi"("error in (no error)"=w258, "Type"=w257, "Control In"=w255) -> ("error out"=w253:errorcluster, "Label.Text"=w244:string, "Diagnostic String"=w243:string)  [unwired: 6 in]
            n119 = case shown="\"Save Config\"" w244 {
              tunnel: w253 -> [w268 w270]
              tunnel: [w268 w270] -> w252
              tunnel: ["Select Config File to Load" "Enter a Filename to Save the\nCurrent Configuration"] -> w251
              frame "False", Default {
              }
              frame "Save Config" {
              }
            }
            n120 = Unbundle By Name(w249) -> ("Queue Array"=w248:T8)
            n121 = call "File Dialog"("prompt"=w251, "error in"=w252) -> ("selected path"=w245:path, "cancelled"=w246:bool, "error out"=w254:errorcluster)  [unwired: 10 in, 1 out]
            n122 = Index Array(array=w248) -> (element=w247:refnum<queue>)  [unwired: 1 in]
            n123 = case shown="False" w246 {
              tunnel: w254 -> [w265 w266]
              tunnel: [w264 w266] -> w250
              tunnel: w247 -> [w263 _]
              tunnel: w245 -> [w261 _]
              tunnel: w244 -> [w262 _]
              frame False {
                n124 = Bundle("Label.Text"=w262, "selected path"=w261) -> (w260:T16)  [unwired: 1 in]
                n125 = Enqueue Element(queue=w263, element=w260, error in (no error)=w265) -> (error out=w264:errorcluster)  [unwired: 1 in, 2 out]
              }
              frame True {
              }
            }
          }
          event "Stop Test", "Pause Test", "Start Test", "Start Pulse", "Save Pulse Data": Value Change {
            # "General Value change button handler"
            n126 = event-data() -> ("CtlRef"=w276:refnum<vi>, "Type"=w285:T13, "NewVal"=w275:bool)  [unwired: 1 in]
            n127 = Unbundle By Name(w282) -> ("Queue Array"=w281:T8)
            n128 = call "Event Case to String.vi"("error in (no error)"=w286, "Type"=w285, "Control In"=w276) -> ("error out"=w284:errorcluster, "Label.Text"=w272:string, "Diagnostic String"=w271:string)  [unwired: 6 in]
            n129 = Index Array(array=w281, index=0) -> (element=w279:refnum<queue>)
            n130 = Bundle By Name(cluster=T9 {"state"="", "data"=variant} ("element"), "state"=w272, "data"=w275) -> (w277:T9)
            n131 = Enqueue Element At Opposite End(queue=w279, element=w277, error in (no error)=w284) -> (error out=w273:errorcluster)  [unwired: 1 in, 2 out]
          }
          event "Path": Value Change {
            # "When the path changes, update the storage thread with the new path"
            n132 = event-data() -> ("NewVal"=w295:path, "CtlRef"=w309:refnum<vi>, "Type"=w312:T13)  [unwired: 1 in]
            n133 = call "Event Case to String.vi"("error in (no error)"=w313, "Type"=w312, "Control In"=w309) -> ("error out"=w311:errorcluster, "Label.Text"=w288:string, "Diagnostic String"=w287:string)  [unwired: 6 in]
            n134 = Strip Path(path=w295) -> (stripped path=w291:path, name=w296:string)
            n135 = Match Pattern(string=w296, regular expression="\\.") -> (before substring=w293:string, after substring=w299:string)  [unwired: 1 in, 2 out]
            n136 = Concatenate Strings(w293, ".csv" ("y")) -> (w292:string)
            n137 = Equal?(x=w299, y="csv") -> (x = y?=w297:bool)
            n138 = Build Path(base path=w291, name or relative path=w292) -> (appended path=w290:path)
            n139 = Select(t=w295, s=w297, f=w290) -> (s? t:f=w289:path)
            n140 = Unbundle By Name(w308) -> ("Queue Array"=w307:T8)
            n141 = local write "Path"(w289) -> ()
            n142 = To Variant(anything=w289) -> (Variant=w301:variant)
            n143 = Bundle By Name(cluster=T9 {"state"="New File", "data"=variant} ("element"), "data"=w301) -> (w302:T9)
            n144 = Index Array(array=w307, index=2) -> (element=w304:refnum<queue>)
            n145 = Enqueue Element(queue=w304, element=w302, error in (no error)=w311) -> (error out=w305:errorcluster)  [unwired: 1 in, 2 out]
          }
          event "Data Setup": Shortcut Menu Selection (User) {
            w315 = ""
            # "Set the selected value for a selection"
            n146 = event-data() -> ("ItemTag"=w321:string, "Coords"=w329:T14, "CtlRef"=w330:refnum<vi>, "Type"=w333:T13)  [unwired: 1 in]
            n147 = call "Event Case to String.vi"("error in (no error)"=w334, "Type"=w333, "Control In"=w330) -> ("error out"=w332:errorcluster)  [unwired: 6 in, 2 out]
            n148 = invoke class="MCListbox (strict)" method="Point To Row Column"(reference=w330, error in=w332, "Point"=w329) -> (error out=w316:errorcluster, "CellPosition"=w328:T15)  [unwired: 4 in, 5 out]
            n149 = Unbundle By Name(w328) -> ("Row"=w320:i32, "Column"=w319:i32)
            n150 = Unbundle By Name(w326) -> ("Queue Array"=w325:T8)
            n151 = Bundle("ItemTag"=w321, "Row"=w320, "Column"=w319) -> (w317:T17)  [unwired: 1 in]
            n152 = Index Array(array=w325, index=1) -> (element=w323:refnum<queue>)
            n153 = Bundle By Name(cluster=T9 {"state"="set active channels", "data"=variant} ("element"), "data"=w317) -> (w318:T9)
            n154 = Enqueue Element At Opposite End(queue=w323, element=w318, error in (no error)=w316) -> (error out=w327:errorcluster)  [unwired: 1 in, 2 out]
          }
          event "Data Setup": Edit Cell {
            w336 = ""
            # "When an edit occurs, update the selected channel"
            n155 = event-data() -> ("String"=w339:string, "Coords"=w338:T15, "CtlRef"=w350:refnum<vi>, "Type"=w352:T13)  [unwired: 1 in]
            n156 = call "Event Case to String.vi"("error in (no error)"=w353, "Type"=w352, "Control In"=w350) -> ("error out"=w337:errorcluster)  [unwired: 6 in, 2 out]
            n157 = Unbundle By Name(w338) -> ("Row"=w343:i32, "Column"=w342:i32)
            n158 = Unbundle By Name(w348) -> ("Queue Array"=w347:T8)
            n159 = Bundle("String"=w339, "Row"=w343, "Column"=w342) -> (w340:T18)  [unwired: 1 in]
            n160 = Index Array(array=w347, index=1) -> (element=w345:refnum<queue>)
            n161 = Bundle By Name(cluster=T9 {"state"="set active channels", "data"=variant} ("element"), "data"=w340) -> (w341:T9)
            n162 = Enqueue Element At Opposite End(queue=w345, element=w341, error in (no error)=w337) -> (error out=w349:errorcluster)  [unwired: 1 in, 2 out]
          }
          event "Data Setup": Shortcut Menu Activation? {
            # "Setup the context menu based on the column"
            n163 = event-data() -> ("MenuRef"=w368:refnum<k9>, "CtlRef"=w363:refnum<vi>, "Type"=w371:T13, "Coords"=w362:T14)  [unwired: 1 in]
            n164 = call "Event Case to String.vi"("error in (no error)"=w372, "Type"=w371, "Control In"=w363) -> ("error out"=w366:errorcluster, "Label.Text"=w356:string, "Diagnostic String"=w355:string)  [unwired: 6 in]
            n165 = invoke on="Invoke Node" class="MCListbox (strict)" method="Point To Row Column"(reference=w363, error in=w366, "Point"=w362) -> (error out=w365:errorcluster, "CellPosition"=w361:T15)  [unwired: 4 in, 5 out]
            n166 = Unbundle By Name(w361) -> ("Row"=w357:i32, "Column"=w360:i32)
            n167 = case shown="0" w360 {
              tunnel: w367 -> [_ _ _ w389]
              tunnel: [string[] [] ("Channels") string[] ["OFF", "RMS", "DC"] ("Channels") string[] ["0", "0.5", "1", "2", "5", "10", "20", "50"] w387] -> w359
              tunnel: w365 -> [w373 w375 w378 w388]
              tunnel: [w373 w375 w378 w388] -> w364
              tunnel: w357 -> [_ _ _ w385]
              frame Default {
              }
              frame 2 {
              }
              frame 3 {
              }
              frame 0 {
                w384 = 15 ("y")
                n168 = Unbundle By Name(w389) -> ("Channels"=w381:string[])
                n169 = Split 1D Array(array=w381, index=w384) -> (first subarray=w379:string[], second subarray=w382:string[])
                n170 = Greater Or Equal?(x=w385, y=w384) -> (x >= y?=w383:bool)
                n171 = Select(t=w382, s=w383, f=w379) -> (s? t:f=w380:string[])
                n172 = Build Array (concatenate)("OFF", w380) -> (w387:string[])
              }
            }
            n173 = Insert Menu Items(6:w364, 7:w359, 8:w359, 9:w368) -> (0:w369:errorcluster)  [unwired: 2 in, 2 out]
            n174 = event-data("Discard?"=w358) -> ()  [unwired: 1 in, 1 out]
          }
          event Value Change {
            w392 = ""
            # "set the ui according to the test selected"
            n175 = event-data() -> ("NewVal"=w393:T2, "CtlRef"=w394:refnum<vi>, "Type"=w426:T13)  [unwired: 1 in]
            n176 = call "Event Case to String.vi"("error in (no error)"=w427, "Type"=w426, "Control In"=w394) -> ("error out"=w424:errorcluster, "Label.Text"=w421:string)  [unwired: 6 in, 1 out]
            n177 = call "Setup per test.vi"("Cluster"=w406, "error in (no error)"=w424, "Label.Text"=w421, "NewVal"=w393, "Enum in"=w394) -> ("error out"=w411:errorcluster, "Test Status"=→"Test Status":string, "String"=→"Test:":string, "Graphic Display"=→"Graphic Display":T4, "Auto Test Controls"=→"Auto Test Controls":T5)  [unwired: 2 out]
            n178 = Format Into String(w393) -> (resulting string=w409:string)  [unwired: 3 in, 1 out]
            n179 = Unbundle By Name(w406) -> ("Queue Array"=w405:T8, "Queue Element"=w398:T9)
            n180 = Bundle By Name(cluster=w398, "state"="set ui", "data"=w393) -> (w403:T9)
            n181 = Index Array(array=w405) -> (element=w404:refnum<queue>)  [unwired: 1 in]
            n182 = Enqueue Element(queue=w404, element=w403, error in (no error)=w411) -> (queue out=w399:refnum<queue>, error out=w401:errorcluster)  [unwired: 1 in, 1 out]
            n183 = Bundle By Name(cluster=w398, "state"="Spin", "data"=cluster{"RPM":dbl, bool} {"RPM"=0.0, FALSE}) -> (w397:T9)
            n184 = call <vilib>:"Application Directory.vi"() -> ("Application Directory"=w417:path)
            n185 = Enqueue Element(queue=w399, element=w397, error in (no error)=w401) -> (error out=w400:errorcluster)  [unwired: 1 in, 2 out]
            n186 = Build Path(base path=w417, name or relative path="data") -> (appended path=w419:path)
            n187 = Build Path(base path=w419, name or relative path="details.ini") -> (appended path=w416:path)
            n188 = call <vilib>:"Open Config Data.vi"("error in (no error)"=w400, "configuration file path"=w416) -> ("error out"=w415:errorcluster, "refnum"=w414:T19)  [unwired: 7 in, 1 out]
            n189 = call-poly <vilib>:"Read Key.vi"("section"=w409, "error in (no error)"=w415, "key"="d", "refnum"=w414) -> ("error out"=w413:errorcluster, "value"=→"Test Description":string, "refnum out"=w412:T19)  [unwired: 4 in, 1 out]
            n190 = call <vilib>:"Close Config Data.vi"("error in (no error)"=w413, "refnum"=w412) -> ("error out"=w410:errorcluster)  [unwired: 8 in, 1 out]
          }
          event "Ibrake": Value Change {
            w429 = ""
            # "Change and update the Ibrake value"
            n191 = event-data() -> ("CtlRef"=w438:refnum<vi>, "Type"=w449:T13, "NewVal"=w432:i32)  [unwired: 1 in]
            n192 = call "Event Case to String.vi"("error in (no error)"=w450, "Type"=w449, "Control In"=w438) -> ("error out"=w435:errorcluster, "Label.Text"=w441:string)  [unwired: 6 in, 1 out]
            n193 = property class="DigNum (strict)"(reference=w438, error in=w435) -> (error out=w434:errorcluster, "Maximum"=w436:dbl, "Minimum"=w437:dbl)  [unwired: 1 out]
            n194 = In Range and Coerce(upper limit=w436, x=w432, lower limit=w437) -> (In Range?=w433:bool)  [unwired: 1 out]
            n195 = Select(t=w432, s=w433, f=0) -> (s? t:f=w430:i32)
            n196 = local write "Ibrake"(w430) -> ()
            n197 = Number To Hexadecimal String(2:w430) -> (0:w439:string)  [unwired: 1 in]
            n198 = Unbundle By Name(w447) -> ("Queue Array"=w446:T8, "Queue Element"=w443:T9)
            n199 = To Variant(anything=w439) -> (Variant=w440:variant)
            n200 = Bundle By Name(cluster=w443, "state"=w441, "data"=w440) -> (w442:T9)
            n201 = Index Array(array=w446) -> (element=w445:refnum<queue>)  [unwired: 1 in]
            n202 = Enqueue Element(queue=w445, element=w442, error in (no error)=w434) -> (error out=w444:errorcluster)  [unwired: 1 in, 2 out]
          }
          event "Range": Value Change {
            w452 = ""
            # "Change and update the range value"
            n203 = event-data() -> ("CtlRef"=w461:refnum<vi>, "Type"=w472:T13, "NewVal"=w455:i32)  [unwired: 1 in]
            n204 = call "Event Case to String.vi"("error in (no error)"=w473, "Type"=w472, "Control In"=w461) -> ("error out"=w458:errorcluster, "Label.Text"=w464:string)  [unwired: 6 in, 1 out]
            n205 = property class="DigNum (strict)"(reference=w461, error in=w458) -> (error out=w457:errorcluster, "Maximum"=w459:dbl, "Minimum"=w460:dbl)  [unwired: 1 out]
            n206 = In Range and Coerce(upper limit=w459, x=w455, lower limit=w460) -> (In Range?=w456:bool)  [unwired: 1 out]
            n207 = Select(t=w455, s=w456, f=0) -> (s? t:f=w453:i32)
            n208 = local write "Range"(w453) -> ()
            n209 = Number To Hexadecimal String(2:w453) -> (0:w462:string)  [unwired: 1 in]
            n210 = Unbundle By Name(w470) -> ("Queue Array"=w469:T8, "Queue Element"=w466:T9)
            n211 = To Variant(anything=w462) -> (Variant=w463:variant)
            n212 = Bundle By Name(cluster=w466, "state"=w464, "data"=w463) -> (w465:T9)
            n213 = Index Array(array=w469) -> (element=w468:refnum<queue>)  [unwired: 1 in]
            n214 = Enqueue Element(queue=w468, element=w465, error in (no error)=w457) -> (error out=w467:errorcluster)  [unwired: 1 in, 2 out]
          }
          event "Step Height": Value Change {
            w475 = ""
            # "Change and update the range value"
            n215 = event-data() -> ("CtlRef"=w484:refnum<vi>, "OldVal"=w495:i32, "NewVal"=w478:i32)  [unwired: 1 in]
            n216 = call "Event Case to String.vi"("error in (no error)"=w496, "Type"=w495, "Control In"=w484) -> ("error out"=w481:errorcluster, "Label.Text"=w487:string)  [unwired: 6 in, 1 out]
            n217 = property class="DigNum (strict)"(reference=w484, error in=w481) -> (error out=w480:errorcluster, "Maximum"=w482:dbl, "Minimum"=w483:dbl)  [unwired: 1 out]
            n218 = In Range and Coerce(upper limit=w482, x=w478, lower limit=w483) -> (In Range?=w479:bool)  [unwired: 1 out]
            n219 = Select(t=w478, s=w479, f=1) -> (s? t:f=w476:i32)
            n220 = local write "Step Height"(w476) -> ()
            n221 = Number To Hexadecimal String(2:w476) -> (0:w485:string)  [unwired: 1 in]
            n222 = Unbundle By Name(w493) -> ("Queue Array"=w492:T8, "Queue Element"=w489:T9)
            n223 = To Variant(anything=w485) -> (Variant=w486:variant)
            n224 = Bundle By Name(cluster=w489, "state"=w487, "data"=w486) -> (w488:T9)
            n225 = Index Array(array=w492) -> (element=w491:refnum<queue>)  [unwired: 1 in]
            n226 = Enqueue Element(queue=w491, element=w488, error in (no error)=w480) -> (error out=w490:errorcluster)  [unwired: 1 in, 2 out]
          }
          event "RPM Target": Value Change {
            w500 = ""
            # "Change and update the RPM value"
            n227 = event-data() -> ("CtlRef"=w510:refnum<vi>, "Type"=w520:T13, "NewVal"=w504:i32)  [unwired: 1 in]
            n228 = call "Event Case to String.vi"("error in (no error)"=w521, "Type"=w520, "Control In"=w510) -> ("error out"=w507:errorcluster, "Label.Text"=w512:string)  [unwired: 6 in, 1 out]
            n229 = property class="DigNum (strict)"(reference=w510, error in=w507) -> (error out=w506:errorcluster, "Maximum"=w508:dbl, "Minimum"=w509:dbl)  [unwired: 1 out]
            n230 = In Range and Coerce(upper limit=w508, x=w504, lower limit=w509) -> (In Range?=w505:bool)  [unwired: 1 out]
            n231 = control-ref of="Average RPM"() -> (w499:refnum<vi>)
            n232 = Select(t=w504, s=w505, f=0) -> (s? t:f=w498:i32)
            n233 = local write "RPM Target"(w498) -> ()
            n234 = local read "Spin"() -> (w502:bool)
            n235 = property class="DigNum (strict)"(reference=w499, "Val(Sgnl)"=w498) -> ()  [unwired: 1 in, 2 out]
            n236 = Bundle("f"=w498, "Spin"=w502) -> (w501:cluster{"f":i32, "Spin":bool})  [unwired: 1 in]
            n237 = Unbundle By Name(w518) -> ("Queue Array"=w517:T8, "Queue Element"=w514:T9)  [unwired: 1 out]
            n238 = To Variant(anything=w501) -> (Variant=w511:variant)
            n239 = Bundle By Name(cluster=w514, "state"=w512, "data"=w511) -> (w513:T9)
            n240 = Index Array(array=w517) -> (element=w516:refnum<queue>)  [unwired: 1 in]
            n241 = Enqueue Element(queue=w516, element=w513, error in (no error)=w506) -> (error out=w515:errorcluster)  [unwired: 1 in, 2 out]
          }
          event "Sample Frequency": Value Change {
            w523 = ""
            # "Change and set the sample frequency"
            n242 = event-data() -> ("CtlRef"=w533:refnum<vi>, "Type"=w542:T13, "NewVal"=w527:dbl)  [unwired: 1 in]
            n243 = call "Event Case to String.vi"("error in (no error)"=w543, "Type"=w542, "Control In"=w533) -> ("error out"=w530:errorcluster, "Label.Text"=w534:string)  [unwired: 6 in, 1 out]
            n244 = property class="DigNum (strict)"(reference=w533, error in=w530) -> (error out=w529:errorcluster, "Maximum"=w531:dbl, "Minimum"=w532:dbl)  [unwired: 1 out]
            n245 = In Range and Coerce(upper limit=w531, x=w527, lower limit=w532) -> (In Range?=w528:bool)  [unwired: 1 out]
            n246 = Select(t=w527, s=w528, f=10.0) -> (s? t:f=w524:dbl)
            n247 = local write "Sample Frequency"(w524) -> ()
            n248 = Unbundle By Name(w540) -> ("Queue Array"=w539:T8, "Queue Element"=w536:T9)
            n249 = Bundle By Name(cluster=w536, "state"=w534, "data"=w524) -> (w535:T9)
            n250 = Index Array(array=w539, index=1) -> (element=w538:refnum<queue>)
            n251 = Enqueue Element At Opposite End(queue=w538, element=w535, error in (no error)=w529) -> (error out=w537:errorcluster)  [unwired: 1 in, 2 out]
          }
          event "Stop Time": Value Change {
            w545 = ""
            w550 = 60.0 ("f")
            # "Set the stop time"
            n252 = event-data() -> ("CtlRef"=w559:refnum<vi>, "Type"=w568:T13, "NewVal"=w548:dbl)  [unwired: 1 in]
            n253 = call "Event Case to String.vi"("error in (no error)"=w569, "Type"=w568, "Control In"=w559) -> ("error out"=w556:errorcluster, "Label.Text"=w560:string)  [unwired: 6 in, 1 out]
            n254 = property class="DigNum (strict)"(reference=w559, error in=w556) -> (error out=w555:errorcluster, "Maximum"=w557:dbl, "Minimum"=w558:dbl)  [unwired: 1 out]
            n255 = local read "S Period"() -> (w549:dbl)
            n256 = Less?(x=w549, y=w548) -> (x < y?=w546:bool)
            n257 = In Range and Coerce(upper limit=w557, x=w548, lower limit=w558) -> (In Range?=w554:bool)  [unwired: 1 out]
            n258 = Compound Arithmetic op=AND(w546, w554) -> (w547:bool)
            n259 = Select(t=w548, s=w547, f=w550) -> (s? t:f=w551:dbl)
            n260 = local write "Stop Time"(w551) -> ()
            n261 = Unbundle By Name(w566) -> ("Queue Array"=w565:T8, "Queue Element"=w562:T9)
            n262 = Multiply(x=w551, y=w550) -> (x*y=w552:dbl)
            n263 = Bundle By Name(cluster=w562, "state"=w560, "data"=w552) -> (w561:T9)
            n264 = Index Array(array=w565, index=1) -> (element=w564:refnum<queue>)
            n265 = Enqueue Element(queue=w564, element=w561, error in (no error)=w555) -> (error out=w563:errorcluster)  [unwired: 1 in, 2 out]
          }
          event "S Period": Value Change {
            w571 = ""
            # "Set the sample period"
            n266 = event-data() -> ("CtlRef"=w586:refnum<vi>, "Type"=w595:T13, "NewVal"=w575:dbl)  [unwired: 1 in]
            n267 = call "Event Case to String.vi"("error in (no error)"=w596, "Type"=w595, "Control In"=w586) -> ("error out"=w583:errorcluster, "Label.Text"=w587:string)  [unwired: 6 in, 1 out]
            n268 = local read "Stop Time"() -> (w576:dbl)
            n269 = property class="DigNum (strict)"(reference=w586, error in=w583) -> (error out=w582:errorcluster, "Maximum"=w584:dbl, "Minimum"=w585:dbl)  [unwired: 1 out]
            n270 = Greater?(x=w576, y=w575) -> (0:w573:bool)
            n271 = In Range and Coerce(upper limit=w584, x=w575, lower limit=w585) -> (In Range?=w581:bool)  [unwired: 1 out]
            n272 = Compound Arithmetic op=AND(w573, w581) -> (w574:bool)
            n273 = Select(t=w575, s=w574, f=1.0) -> (s? t:f=w578:dbl)
            n274 = local write "S Period"(w578) -> ()
            n275 = Unbundle By Name(w593) -> ("Queue Array"=w592:T8, "Queue Element"=w589:T9)
            n276 = Multiply(x=w578, y=60.0) -> (x*y=w579:dbl)
            n277 = Bundle By Name(cluster=w589, "state"=w587, "data"=w579) -> (w588:T9)
            n278 = Index Array(array=w592, index=1) -> (element=w591:refnum<queue>)
            n279 = Enqueue Element(queue=w591, element=w588, error in (no error)=w582) -> (error out=w590:errorcluster)  [unwired: 1 in, 2 out]
          }
          event "Thermal Limit": Value Change {
            w598 = ""
            # "Update the thermal limit when it changes"
            n280 = event-data() -> ("CtlRef"=w618:refnum<vi>, "Type"=w624:T13, "NewVal"=w606:i32)  [unwired: 1 in]
            n281 = Unbundle By Name(w609) -> ("Thermal Resume"=w607:i32)
            n282 = call "Event Case to String.vi"("error in (no error)"=w625, "Type"=w624, "Control In"=w618) -> ("error out"=w615:errorcluster, "Label.Text"=w619:string)  [unwired: 6 in, 1 out]
            n283 = property class="DigNum (strict)"(reference=w618, error in=w615) -> (error out=w602:errorcluster, "Maximum"=w616:dbl, "Minimum"=w617:dbl)  [unwired: 1 out]
            n284 = In Range and Coerce(upper limit=w616, x=w606, lower limit=w617) -> (In Range?=w614:bool)  [unwired: 1 out]
            n285 = Less?(x=w607, y=w606) -> (x < y?=w605:bool)
            n286 = Compound Arithmetic op=AND(w605, w614) -> (w608:bool)
            n287 = Select(t=w606, s=w608, f=200) -> (s? t:f=w610:i32)
            n288 = Bundle By Name(cluster=w609, "Thermal Limit"=w610) -> (w611:T7)
            n289 = local write "Thermal Limit"(w610) -> ()
            n290 = Unbundle By Name(w611) -> ("Queue Array"=w622:T8, "Queue Element"=w620:T9)
            n291 = Bundle By Name(cluster=w620, "state"=w619, "data"=w610) -> (w599:T9)
            n292 = Index Array(array=w622, index #1=0 ("index"), index #2=1 ("index")) -> (element #1=w600:refnum<queue>, element #2=w621:refnum<queue>)
            n293 = Enqueue Element(queue=w600, element=w599, error in (no error)=w602) -> (error out=w601:errorcluster)  [unwired: 1 in, 2 out]
            n294 = Enqueue Element(queue=w621, element=w599, error in (no error)=w601) -> (error out=w604:errorcluster)  [unwired: 1 in, 2 out]
          }
          event "Thermal Resume": Value Change {
            w627 = ""
            # "Set the therma limit to allow the test to resume"
            n295 = event-data() -> ("CtlRef"=w647:refnum<vi>, "Type"=w653:T13, "NewVal"=w639:i32)  [unwired: 1 in]
            n296 = Unbundle By Name(w636) -> ("Thermal Limit"=w640:i32)
            n297 = call "Event Case to String.vi"("error in (no error)"=w654, "Type"=w653, "Control In"=w647) -> ("error out"=w644:errorcluster, "Label.Text"=w648:string)  [unwired: 6 in, 1 out]
            n298 = property class="DigNum (strict)"(reference=w647, error in=w644) -> (error out=w630:errorcluster, "Maximum"=w645:dbl, "Minimum"=w646:dbl)  [unwired: 1 out]
            n299 = In Range and Coerce(upper limit=w645, x=w639, lower limit=w646) -> (In Range?=w643:bool)  [unwired: 1 out]
            n300 = Greater?(x=w640, y=w639) -> (0:w637:bool)
            n301 = Compound Arithmetic op=AND(w637, w643) -> (w638:bool)
            n302 = Select(t=w639, s=w638, f=5) -> (s? t:f=w633:i32)
            n303 = Bundle By Name(cluster=w636, "Thermal Resume"=w633) -> (w635:T7)
            n304 = local write "Thermal Resume"(w633) -> ()
            n305 = Unbundle By Name(w635) -> ("Queue Array"=w651:T8, "Queue Element"=w649:T9)
            n306 = Bundle By Name(cluster=w649, "state"=w648, "data"=w633) -> (w628:T9)
            n307 = Index Array(array=w651, index #1=0 ("index"), index #2=1 ("index")) -> (element #1=w629:refnum<queue>, element #2=w650:refnum<queue>)
            n308 = Enqueue Element(queue=w629, element=w628, error in (no error)=w630) -> (error out=w631:errorcluster)  [unwired: 1 in, 2 out]
            n309 = Enqueue Element(queue=w650, element=w628, error in (no error)=w631) -> (error out=w634:errorcluster)  [unwired: 1 in, 2 out]
          }
          event "Spin": Value Change {
            # "Start or stop rotation"
            n310 = event-data() -> ("CtlRef"=w663:refnum<vi>, "Type"=w665:T13, "NewVal"=w659:bool)  [unwired: 1 in]
            n311 = local read "Over Temp"() -> (w656:bool)
            n312 = call "Event Case to String.vi"("error in (no error)"=w666, "Type"=w665, "Control In"=w663) -> ("error out"=w661:errorcluster, "Label.Text"=w658:string, "Diagnostic String"=w657:string)  [unwired: 6 in]
            n313 = case shown="False" w656 {
              tunnel: w662 -> [w679 _]
              tunnel: w661 -> [_ w681]
              tunnel: [w676 w681] -> w660
              tunnel: w659 -> [w673 _]
              tunnel: w658 -> [w669 _]
              frame False {
                n314 = Bundle("RPM Target"="RPM Target", "NewVal"=w673) -> (w671:cluster{"RPM Target":i32, "NewVal":bool})  [unwired: 1 in]
                n315 = Unbundle By Name(w679) -> ("Queue Array"=w678:T8, "Queue Element"=w675:T9)
                n316 = To Variant(anything=w671) -> (Variant=w672:variant)
                n317 = Bundle By Name(cluster=w675, "state"=w669, "data"=w672) -> (w674:T9)
                n318 = Index Array(array=w678, index=0) -> (element=w677:refnum<queue>)
                n319 = Enqueue Element(queue=w677, element=w674) -> (error out=w676:errorcluster)  [unwired: 2 in, 2 out]
              }
              frame True {
                n320 = local write "Spin"(FALSE) -> ()
              }
            }
          }
          event Value Change {
            w682 = ""
            # "Update the load bank setting"
            n321 = event-data() -> ("CtlRef"=w693:refnum<vi>, "Type"=w695:T13, "NewVal"=w683:T3)  [unwired: 1 in]
            n322 = call "Event Case to String.vi"("error in (no error)"=w696, "Type"=w695, "Control In"=w693) -> ("error out"=w684:errorcluster, "Label.Text"=w686:string)  [unwired: 6 in, 1 out]
            n323 = Unbundle By Name(w692) -> ("Queue Array"=w691:T8, "Queue Element"=w688:T9)
            n324 = To Variant(anything=w683) -> (Variant=w685:variant)
            n325 = Bundle By Name(cluster=w688, "state"=w686, "data"=w685) -> (w687:T9)
            n326 = Index Array(array=w691) -> (element=w690:refnum<queue>)  [unwired: 1 in]
            n327 = Enqueue Element(queue=w690, element=w687, error in (no error)=w684) -> (error out=w689:errorcluster)  [unwired: 1 in, 2 out]
          }
          event "Ibrake Sweep": Value Change {
            w698 = ""
            # "Set the Ibrake sweep"
            n328 = event-data() -> ("CtlRef"=w724:refnum<vi>, "Type"=w714:T13, "NewVal"=w701:string)  [unwired: 1 in]
            n329 = call "Event Case to String.vi"("error in (no error)"=w726, "Type"=w714, "Control In"=w724) -> ("error out"=w720:errorcluster, "Label.Text"=w716:string)  [unwired: 6 in, 1 out]
            n330 = Spreadsheet String To Array(delimiter (Tab)=",", format string="", spreadsheet string=w701, array type (2D Dbl)=i32[] []) -> (array=w710:i32[])
            n331 = Array Size(array=w710) -> (size(s)=w706:i32)
            n332 = In Range and Coerce(upper limit=2500, x=w710, lower limit=0) -> (In Range?=w707:bool[])  [unwired: 1 out]
            n333 = And Array Elements(Boolean array=w707) -> (logical AND=w704:bool)
            n334 = Less Or Equal?(x=w706, y=26) -> (x <= y?=w703:bool)
            n335 = And(x=w703, y=w704) -> (x .and. y?=w702:bool)
            n336 = Select(t=w701, s=w702, f="0") -> (s? t:f=w699:string)
            n337 = local write "Ibrake Sweep"(w699) -> ()
            n338 = Unbundle By Name(w723) -> ("Queue Array"=w722:T8, "Queue Element"=w718:T9)
            n339 = To Variant(anything=w699) -> (Variant=w715:variant)
            n340 = Bundle By Name(cluster=w718, "state"=w716, "data"=w715) -> (w717:T9)
            n341 = Index Array(array=w722) -> (element=w721:refnum<queue>)  [unwired: 1 in]
            n342 = Enqueue Element(queue=w721, element=w717, error in (no error)=w720) -> (error out=w719:errorcluster)  [unwired: 1 in, 2 out]
          }
          event "Step Height Sweep": Value Change {
            w728 = ""
            # "Set the resistance sweep"
            n343 = event-data() -> ("CtlRef"=w754:refnum<vi>, "Type"=w744:T13, "NewVal"=w731:string)  [unwired: 1 in]
            n344 = call "Event Case to String.vi"("error in (no error)"=w756, "Type"=w744, "Control In"=w754) -> ("error out"=w750:errorcluster, "Label.Text"=w746:string)  [unwired: 6 in, 1 out]
            n345 = Spreadsheet String To Array(delimiter (Tab)=",", format string="", spreadsheet string=w731, array type (2D Dbl)=i32[] []) -> (array=w740:i32[])
            n346 = Array Size(array=w740) -> (size(s)=w736:i32)
            n347 = In Range and Coerce(upper limit=25, x=w740, lower limit=0) -> (In Range?=w737:bool[])  [unwired: 1 out]
            n348 = And Array Elements(Boolean array=w737) -> (logical AND=w734:bool)
            n349 = Less Or Equal?(x=w736, y=26) -> (x <= y?=w733:bool)
            n350 = And(x=w733, y=w734) -> (x .and. y?=w732:bool)
            n351 = Select(t=w731, s=w732, f="0") -> (s? t:f=w729:string)
            n352 = local write "Step Height Sweep"(w729) -> ()
            n353 = Unbundle By Name(w753) -> ("Queue Array"=w752:T8, "Queue Element"=w748:T9)
            n354 = To Variant(anything=w729) -> (Variant=w745:variant)
            n355 = Bundle By Name(cluster=w748, "state"=w746, "data"=w745) -> (w747:T9)
            n356 = Index Array(array=w752) -> (element=w751:refnum<queue>)  [unwired: 1 in]
            n357 = Enqueue Element(queue=w751, element=w747, error in (no error)=w750) -> (error out=w749:errorcluster)  [unwired: 1 in, 2 out]
          }
          event "Range Sweep": Value Change {
            w758 = ""
            # "Set the resistance sweep"
            n358 = event-data() -> ("CtlRef"=w784:refnum<vi>, "Type"=w774:T13, "NewVal"=w761:string)  [unwired: 1 in]
            n359 = call "Event Case to String.vi"("error in (no error)"=w786, "Type"=w774, "Control In"=w784) -> ("error out"=w780:errorcluster, "Label.Text"=w776:string)  [unwired: 6 in, 1 out]
            n360 = Spreadsheet String To Array(delimiter (Tab)=",", format string="", spreadsheet string=w761, array type (2D Dbl)=i32[] []) -> (array=w770:i32[])
            n361 = Array Size(array=w770) -> (size(s)=w766:i32)
            n362 = In Range and Coerce(upper limit=25, x=w770, lower limit=0) -> (In Range?=w767:bool[])  [unwired: 1 out]
            n363 = And Array Elements(Boolean array=w767) -> (logical AND=w764:bool)
            n364 = Less Or Equal?(x=w766, y=26) -> (x <= y?=w763:bool)
            n365 = And(x=w763, y=w764) -> (x .and. y?=w762:bool)
            n366 = Select(t=w761, s=w762, f="0") -> (s? t:f=w759:string)
            n367 = local write "Range Sweep"(w759) -> ()
            n368 = Unbundle By Name(w783) -> ("Queue Array"=w782:T8, "Queue Element"=w778:T9)
            n369 = To Variant(anything=w759) -> (Variant=w775:variant)
            n370 = Bundle By Name(cluster=w778, "state"=w776, "data"=w775) -> (w777:T9)
            n371 = Index Array(array=w782) -> (element=w781:refnum<queue>)  [unwired: 1 in]
            n372 = Enqueue Element(queue=w781, element=w777, error in (no error)=w780) -> (error out=w779:errorcluster)  [unwired: 1 in, 2 out]
          }
          event "Load Sweep": Value Change {
            w788 = ""
            # "Set the load sweep"
            n373 = event-data() -> ("CtlRef"=w814:refnum<vi>, "Type"=w804:T13, "NewVal"=w791:string)  [unwired: 1 in]
            n374 = call "Event Case to String.vi"("error in (no error)"=w816, "Type"=w804, "Control In"=w814) -> ("error out"=w810:errorcluster, "Label.Text"=w806:string)  [unwired: 6 in, 1 out]
            n375 = Spreadsheet String To Array(delimiter (Tab)=",", format string="", spreadsheet string=w791, array type (2D Dbl)=i32[] []) -> (array=w800:i32[])
            n376 = Array Size(array=w800) -> (size(s)=w796:i32)
            n377 = In Range and Coerce(upper limit=50, x=w800, lower limit=0) -> (In Range?=w797:bool[])  [unwired: 1 out]
            n378 = And Array Elements(Boolean array=w797) -> (logical AND=w794:bool)
            n379 = Less Or Equal?(x=w796, y=17) -> (x <= y?=w793:bool)
            n380 = And(x=w793, y=w794) -> (x .and. y?=w792:bool)
            n381 = Select(t=w791, s=w792, f="50") -> (s? t:f=w789:string)
            n382 = local write "Load Sweep"(w789) -> ()
            n383 = Unbundle By Name(w813) -> ("Queue Array"=w812:T8, "Queue Element"=w808:T9)
            n384 = To Variant(anything=w789) -> (Variant=w805:variant)
            n385 = Bundle By Name(cluster=w808, "state"=w806, "data"=w805) -> (w807:T9)
            n386 = Index Array(array=w812) -> (element=w811:refnum<queue>)  [unwired: 1 in]
            n387 = Enqueue Element(queue=w811, element=w807, error in (no error)=w810) -> (error out=w809:errorcluster)  [unwired: 1 in, 2 out]
          }
          event "RPM Sweep": Value Change {
            w818 = ""
            # "Set the RPM sweep"
            n388 = event-data() -> ("CtlRef"=w844:refnum<vi>, "Type"=w834:T13, "NewVal"=w821:string)  [unwired: 1 in]
            n389 = call "Event Case to String.vi"("error in (no error)"=w846, "Type"=w834, "Control In"=w844) -> ("error out"=w840:errorcluster, "Label.Text"=w836:string)  [unwired: 6 in, 1 out]
            n390 = Spreadsheet String To Array(delimiter (Tab)=",", format string="", spreadsheet string=w821, array type (2D Dbl)=i32[] []) -> (array=w830:i32[])
            n391 = Array Size(array=w830) -> (size(s)=w826:i32)
            n392 = In Range and Coerce(upper limit=250, x=w830, lower limit=0) -> (In Range?=w827:bool[])  [unwired: 1 out]
            n393 = And Array Elements(Boolean array=w827) -> (logical AND=w824:bool)
            n394 = Less Or Equal?(x=w826, y=25) -> (x <= y?=w823:bool)
            n395 = And(x=w823, y=w824) -> (x .and. y?=w822:bool)
            n396 = Select(t=w821, s=w822, f="0") -> (s? t:f=w819:string)
            n397 = local write "RPM Sweep"(w819) -> ()
            n398 = Unbundle By Name(w843) -> ("Queue Array"=w842:T8, "Queue Element"=w838:T9)
            n399 = To Variant(anything=w819) -> (Variant=w835:variant)
            n400 = Bundle By Name(cluster=w838, "state"=w836, "data"=w835) -> (w837:T9)
            n401 = Index Array(array=w842) -> (element=w841:refnum<queue>)  [unwired: 1 in]
            n402 = Enqueue Element(queue=w841, element=w837, error in (no error)=w840) -> (error out=w839:errorcluster)  [unwired: 1 in, 2 out]
          }
          event "FanMode": Mouse Up {
            w848 = ""
            # "Set the fan mode"
            n403 = event-data() -> ("CtlRef"=w858:refnum<vi>, "Type"=w849:T13)  [unwired: 1 in, 4 out]
            n404 = local read "Fan Mode LED Array"() -> (w854:bool[])
            n405 = call "Event Case to String.vi"("error in (no error)"=w856, "Type"=w849, "Control In"=w858) -> ("error out"=w850:errorcluster, "Label.Text"=w859:string)  [unwired: 6 in, 1 out]
            n406 = Rotate 1D Array(1:w854, 2:1 ("n")) -> (0:w853:bool[])
            "Fan Mode LED Array" <- w853
            n407 = Search 1D Array(1D array=w853, element=TRUE) -> (index of element=w851:i32)  [unwired: 1 in]
            n408 = Unbundle By Name(w855) -> ("Queue Array"=w864:T8, "Queue Element"=w861:T9)
            n409 = Bundle By Name(cluster=w861, "state"=w859, "data"=w851) -> (w860:T9)
            n410 = Index Array(array=w864) -> (element=w863:refnum<queue>)  [unwired: 1 in]
            n411 = Enqueue Element(queue=w863, element=w860, error in (no error)=w850) -> (error out=w862:errorcluster)  [unwired: 1 in, 2 out]
          }
          event "Thermal Equilibrium": Value Change {
            w867 = ""
            # "Set the Thermal Equilibrium Test mode"
            n412 = event-data() -> ("CtlRef"=w873:refnum<vi>, "NewVal"=w868:bool, "Type"=w869:T13)  [unwired: 1 in, 1 out]
            n413 = call "Event Case to String.vi"("error in (no error)"=w872, "Type"=w869, "Control In"=w873) -> ("error out"=w870:errorcluster, "Label.Text"=w874:string)  [unwired: 6 in, 1 out]
            n414 = Unbundle By Name(w871) -> ("Queue Array"=w879:T8, "Queue Element"=w876:T9)
            n415 = Bundle By Name(cluster=w876, "state"=w874, "data"=w868) -> (w875:T9)
            n416 = Index Array(array=w879) -> (element=w878:refnum<queue>)  [unwired: 1 in]
            n417 = Enqueue Element(queue=w878, element=w875, error in (no error)=w870) -> (error out=w877:errorcluster)  [unwired: 1 in, 2 out]
          }
          event User Event {
            w882 = ""
            # "Handle programmatic events"
            n418 = event-data() -> ("Type"=w896:u32, "state"=w884:string, "data"=w883:variant)  [unwired: 1 in]
            n419 = Format Into String(error in=w894, w884) -> (resulting string=w895:string, error out=w893:errorcluster)  [unwired: 2 in]
            n420 = call "Event Case to String.vi"("Additional Info"=w895, "error in (no error)"=w893, "Type"=w896) -> ("error out"=w887:errorcluster)  [unwired: 6 in, 2 out]
            n421 = case shown="\"Exit\"" w884 {
              tunnel: [w900 w902 w911] -> w892
              tunnel: w891 -> [w900 w902 w911]
              tunnel: [w899 w904 w912] -> w890
              tunnel: w889 -> [w899 w904 w912]
              tunnel: [w898 w901 w906] -> w888
              tunnel: w887 -> [w898 w901 w907]
              tunnel: [w897 w903 TRUE] -> w886
              tunnel: w885 -> [w897 w903 _]
              tunnel: w883 -> [_ _ _]
              frame Default {
                # "Default case for duplication"
              }
              frame "Init" {
                # "Removed This Section and Placed it on Init Main.vi"
                # "Initialize the queus"
              }
              frame "Exit" {
                # "Close references and exit"
                n422 = Unbundle By Name(w911) -> ("System Event"=w910:refnum<user-event>, "System Event RefNum"=w908:refnum<event-registration>)
                n423 = Destroy User Event(user event=w910, error in=w907) -> (error out=w909:errorcluster)
                n424 = Unregister For Events(event registration refnum=w908, error in=w909) -> (error out=w906:errorcluster)
              }
            }
          }
          event Panel Close? {
            w913 = ""
            # "Begins the exit procedure"
            n425 = event-data() -> ("Type"=w925:T13)  [unwired: 1 in]
            n426 = Unbundle By Name(w922) -> ("Queue Array"=w918:T8)
            n427 = call "Event Case to String.vi"("Additional Info"="Panel Close", "error in (no error)"=w926, "Type"=w925) -> ("error out"=w917:errorcluster)  [unwired: 6 in, 2 out]
            n428 = Index Array(array=w918) -> (element=w915:refnum<queue>)  [unwired: 1 in]
            n429 = Enqueue Element(queue=w915, element=T9 {"state"="save config", "data"=variant}, error in (no error)=w917) -> (error out=w916:errorcluster)  [unwired: 1 in, 2 out]
            n430 = for {
              tunnel: w916 -> [w928]
              tunnel: [w932] -> w921
              tunnel: w918 -> [w930] mode=indexing
              n431 = Flush Queue(queue=w930, error in (no error)=w928) -> (queue out=w929:refnum<queue>, error out=w927:errorcluster)  [unwired: 1 out]
              n432 = Enqueue Element At Opposite End(queue=w929, element=T9 {"state"="Exit", "data"=variant}, error in (no error)=w927) -> (error out=w932:errorcluster)  [unwired: 1 in, 2 out]
            }
            n433 = Not(x=w919) -> (.not. x?=w920:bool)
            n434 = event-data("Discard?"=w920) -> ()  [unwired: 1 in, 1 out]
          }
        }
      }
      frame Error {
        n435 = Unbundle By Name(w935) -> ("Queue List"=w934:string[], "Queue Array"=w933:T8, "Last State"=w938:string)
        n436 = call "Reentrant Send Error.vi"("Queue Names"=w934, "error in (no error)"=w937, "Last State"=w938, "Queues"=w933) -> ("error out"=w936:errorcluster)  [unwired: 7 in]
      }
    }
    n437 = Concatenate Strings(w61, w62, w60, w62) -> (w59:string)
    n438 = Bundle By Name(cluster=w65, "Last State"=w59) -> (w63:T7)
  }
  n439 = while {
    shift-right: [w941] -> _
    shift-left: w2 -> [w945]
    shift-right: [w943] -> w56
    shift-left: w5 -> [w944]
    i -> [w940]
    stop <- w942 stop-if-true
    # "Command Arbitrator"
    n440 = case shown="No Error" w944 {
      selector: w944 -> [w956 w2282]
      tunnel: w945 -> [w950 w2280]
      tunnel: [w954 w2281] -> w943
      tunnel: [w953 FALSE] -> w942
      tunnel: [w951 w2280] -> w941
      tunnel: w940 -> [_ _]
      frame No Error {
        n441 = Unbundle By Name(w950) -> ("Queue Array"=w958:T8)
        n442 = call "Dequeue Element.vi"("timeout in ms (-1)"=50, "error in (no error)"=w956, "index"=0, "Queue Array"=w958) -> ("error out"=w955:errorcluster, "Queue Element"=w947:T9)  [unwired: 5 in, 1 out]
        n443 = Unbundle By Name(w947) -> ("state"=w946:string, "data"=w952:variant)
        n444 = Bundle By Name(cluster=w950, "Last State"=w946) -> (w948:T7)
        n445 = case shown="\"Console Select\"" w946 {
          selector: w946 -> [_ _ _ _ _ _ _ _ _ _ _ _ _ _ w1492 _ _ _ _ _ _ _ _ _ _ _ _ _ _ _ _ _ _ _ _ _ _ _]
          tunnel: w955 -> [w988 w1025 w1039 w1076 w1125 w1171 w1188 w1235 w1260 w1282 w1366 w1394 w1447 w1467 w1514 w1586 w1624 w1657 w1690 w1713 w1736 w1759 w1780 w1823 w1872 w1888 w1921 w1941 w1957 w1984 w2027 w2103 w2144 w2185 w2213 w2230 w2247 w2269]
          tunnel: [w960 w1017 w1044 w1081 w1131 w1166 w1211 w1225 w1250 w1274 w1352 w1383 w1442 w1473 w1507 w1579 w1605 w1638 w1671 w1708 w1731 w1754 w1775 w1790 w1855 w1896 w1917 w1929 w1952 w1980 w2035 w2080 w2128 w2178 w2212 w2229 w2246 w2265] -> w954
          tunnel: [FALSE FALSE FALSE FALSE FALSE TRUE FALSE FALSE FALSE FALSE FALSE FALSE FALSE FALSE FALSE FALSE FALSE FALSE FALSE FALSE FALSE FALSE FALSE FALSE FALSE FALSE FALSE FALSE FALSE FALSE FALSE FALSE FALSE FALSE FALSE FALSE FALSE FALSE] -> w953
          tunnel: w952 -> [w986 w1023 _ _ _ w1169 _ w1233 w1258 w1280 w1364 w1392 w1445 _ w1511 w1584 w1622 w1655 w1688 w1711 w1734 w1757 w1778 w1821 w1870 _ w1919 w1939 w1955 w1982 _ w2100 w2142 w2183 w2210 w2227 w2244 w2267]
          tunnel: [w976 w1016 w1043 w1080 w1130 w1167 w1213 w1223 w1249 w1276 w1356 w1386 w1438 w1475 w1509 w1562 w1602 w1635 w1668 w1704 w1727 w1750 w1771 w1817 w1854 w1897 w1910 w1937 w1950 w1971 w2034 w2098 w2127 w2179 w2206 w2223 w2240 w2264] -> w951
          tunnel: w948 -> [w966 w1019 w1043 w1080 w1130 w1167 w1214 w1223 w1249 w1278 w1358 w1386 w1436 w1476 w1509 w1566 w1612 w1645 w1678 w1703 w1726 w1749 w1769 w1816 w1854 w1905 w1910 w1937 w1950 w1971 w2029 w2098 w2127 w2179 w2208 w2225 w2242 w2264]
          frame "Amplitude", "Average RPM", "Pulse Frequency" {
            w977 = 100.0 ("y")
            # "This case defines the pulse parameters for pulse testing"
            n446 = Unbundle By Name(w966) -> ("Current RPM"=w959:dbl, "Ctrl Refs.RPM Graph"=w973:refnum<vi>)
            n447 = Not Equal?(x=variant, y=w986) -> (x != y?=w985:bool)
            n448 = case shown="False" w985 {
              tunnel: w988 -> [w1003 w1008]
              tunnel: [w1003 w1007] -> w970
              tunnel: w986 -> [_ w1006]
              tunnel: [w1002 w1005] -> _
              tunnel: w985 -> [w1002 w1004]
              frame False {
              }
              frame True {
                n449 = Variant To Data(error in=w1008, type=w1004, Variant=w1006) -> (data=w1005:bool, error out=w1007:errorcluster)
              }
            }
            n450 = Greater Than 0?(x=w959) -> (x > 0?=w972:bool)
            n451 = case shown="True" w972 {
              tunnel: w973 -> [_ w1001]
              tunnel: w959 -> [_ w998]
              tunnel: [w994 w999] -> w971
              tunnel: w970 -> [w994 w1000]
              frame False {
              }
              frame True {
                n452 = local read "RPM Target"() -> (w995:i32)
                n453 = Multiply(x=w998, y=2.0) -> (x*y=w996:dbl)
                n454 = property class="XYGraph (strict)"(reference=w1001, error in=w1000, "YScale.Maximum"=w996) -> (error out=w999:errorcluster)  [unwired: 1 out]
                n455 = local write "Average RPM"(w995) -> ()
              }
            }
            n456 = Multiply(x="Pulse Frequency", y=w977) -> (x*y=w980:dbl)
            n457 = Bundle By Name(cluster=cluster{"Fs":dbl, "#s":dbl} {"Fs"=20.0, "#s"=20.0} ("sampling info"), "Fs"=w980, "#s"=w977) -> (w978:cluster{"Fs":dbl, "#s":dbl})
            n458 = call <vilib>:"Sine Waveform.vi"("offset"=w959, "sampling info"=w978, "error in (no error)"=w971, "amplitude"="Amplitude", "frequency"="Pulse Frequency") -> ("error out"=w968:errorcluster, "signal out"=w974:waveform(dbl))  [unwired: 5 in]
            "Waveform Graph" <- w974
            n459 = Unbundle By Name(w966) -> ("Queue Array"=w965:T8, "Queue Element"=w963:T9)
            n460 = Unbundle By Name(w974) -> ("Y"=w983:dbl[])
            n461 = expression code="x*0.033"(w983) -> (w982:dbl[])
            n462 = local read "Start Pulse"() -> (w967:bool)
            n463 = Bundle By Name(cluster=w963, "state"="Start Pulse") -> (w961:T9)
            n464 = Bundle By Name(cluster=w974, "Y"=w982) -> (w975:waveform(dbl))
            n465 = Index Array(array=w965) -> (element=w964:refnum<queue>)  [unwired: 1 in]
            n466 = case shown="True" w967 {
              tunnel: w968 -> [w989 w991]
              tunnel: w964 -> [_ w993]
              tunnel: w961 -> [_ w992]
              tunnel: [w989 w990] -> w960
              frame False {
              }
              frame True {
                n467 = Enqueue Element At Opposite End(queue=w993, element=w992, error in (no error)=w991) -> (error out=w990:errorcluster)  [unwired: 1 in, 2 out]
              }
            }
            n468 = Bundle By Name(cluster=w966, "Pulse Waveform"=w975) -> (w976:T7)
          }
          frame "Available Tests" {
            # "This queue sets up the system for the selected test"
            n469 = Unbundle By Name(w1019) -> ("Available Tests"=w1021:T2)
            n470 = Not Equal?(x=variant, y=w1023) -> (x != y?=w1022:bool)
            n471 = case shown="True" w1022 {
              tunnel: w1025 -> [w1027 w1032]
              tunnel: [w1027 w1031] -> w1018
              tunnel: w1023 -> [_ w1030]
              tunnel: [w1026 w1029] -> w1020
              tunnel: w1021 -> [w1026 w1028]
              frame False {
              }
              frame True {
                n472 = Variant To Data(error in=w1032, type=w1028, Variant=w1030) -> (data=w1029:T2, error out=w1031:errorcluster)
              }
            }
            n473 = Bundle By Name(cluster=w1019, "Available Tests"=w1020) -> (w1016:T7)
            n474 = Unbundle By Name(w1016) -> ("Queue Array"=w1015:T8, "Queue Element"=w1012:T9)
            n475 = Bundle By Name(cluster=w1012, "state"="load data") -> (w1011:T9)
            n476 = Index Array(array=w1015, index=1) -> (element=w1014:refnum<queue>)
            n477 = Enqueue Element(queue=w1014, element=w1011, error in (no error)=w1018) -> (error out=w1017:errorcluster)  [unwired: 1 in, 2 out]
          }
          frame "Check Temp" {
            # "Case to check the temperature during a sequence"
            n478 = flat-sequence {
              tunnel: [w1046] -> w1034
              frame #0 {
                # "Create Delay to avoid process overload"
                n479 = Wait (ms)(milliseconds to wait=u32 100) -> ()  [unwired: 1 out]
              }
              frame #1 {
                n480 = local read "Over Temp"() -> (w1046:bool)
              }
            }
            n481 = Unbundle By Name(w1043) -> ("Queue Array"=w1042:T8)
            n482 = local read "Stop Test"() -> (w1037:bool)
            n483 = local write "Test Status"("Running" ("Test Status")) -> ()
            n484 = Select(t=T9 {"state"="Check temp", "data"=variant} ("element"), s=w1034, f=T9 {"state"="Set parameters", "data"=variant} ("element")) -> (s? t:f=w1040:T9)
            n485 = Index Array(array=w1042) -> (element=w1041:refnum<queue>)  [unwired: 1 in]
            n486 = case shown="False" w1037 {
              tunnel: [w1050 w1051] -> w1044
              tunnel: w1041 -> [w1049 _]
              tunnel: w1040 -> [w1048 _]
              tunnel: w1039 -> [w1047 w1051]
              frame False {
                n487 = Enqueue Element At Opposite End(queue=w1049, element=w1048, error in (no error)=w1047) -> (error out=w1050:errorcluster)  [unwired: 1 in, 2 out]
              }
              frame True {
              }
            }
          }
          frame "dwell for resume" {
            # "IF T<T_Resume&&OverTemp==0"
            # "Wait for temperatures to be within boundaries to resume testing"
            n488 = flat-sequence {
              tunnel: [w1083] -> w1053
              frame #0 {
                # "Create Delay to avoid process overload"
                n489 = Wait (ms)(milliseconds to wait=u32 100) -> ()  [unwired: 1 out]
              }
              frame #1 {
                n490 = local read "Over Temp"() -> (w1083:bool)
              }
            }
            n491 = Unbundle By Name(w1080) -> ("Queue Array"=w1079:T8, "Available Tests"=w1074:T2, "T_0 Index"=w1065:i32)
            n492 = local read "CH Value"() -> (w1054:dbl[])
            n493 = property on="Data Setup" class="MCListbox (strict)"() -> ("ItemSyms"=w1067:i32[])  [unwired: 2 in, 2 out]
            n494 = local read "Thermal Resume"() -> (w1066:i32)
            n495 = for {
              N -> [w1086]
              tunnel: w1054 -> [w1092]
              tunnel: [w1091] -> w1072 mode=indexing if=w1089
              tunnel: w1067 -> [w1090] mode=indexing
              tunnel: [w1086] -> _ mode=indexing
              tunnel: w1065 -> [w1084]
              i -> [w1088]
              n496 = Subtract(x=w1088, y=w1084) -> (x-y=w1085:i32)
              n497 = Equal?(x=w1090, y=1) -> (x = y?=w1089:bool)
              n498 = Index Array(array=w1092, index=w1085) -> (element=w1091:dbl)
            }
            n499 = To Double Precision Float(number=w1066) -> (double precision float=w1071:dbl)
            n500 = Less?(x=w1072, y=w1071) -> (x < y?=w1070:bool[])
            n501 = And Array Elements(Boolean array=w1070) -> (logical AND=w1069:bool)
            n502 = Bundle By Name(cluster=T9 {"state"="FanMode", "data"=variant} ("element"), "data"=FanMode."On" ("FanMode")) -> (w1058:T9)
            n503 = Bundle By Name(cluster=T9 {"state"="FanMode", "data"=variant} ("element"), "data"=FanMode."Off" ("FanMode")) -> (w1056:T9)
            n504 = Build Array(T9 {"state"="dwell for resume", "data"=variant} ("element"), w1058) -> (w1060:T9[])
            n505 = Build Array(T9 {"state"="Set parameters", "data"=variant} ("element"), w1056) -> (w1059:T9[])
            n506 = Compound Arithmetic op=AND(w1069, invert w1053) -> (w1068:bool)
            n507 = local read "Stop Test"() -> (w1075:bool)
            n508 = Select(t=w1059, s=w1068, f=w1060) -> (s? t:f=w1077:T9[])
            n509 = Index Array(array=w1079) -> (element=w1078:refnum<queue>)  [unwired: 1 in]
            n510 = case shown="\"EFX Brake Torque\", Default" w1074 {
              tunnel: [w1094 w1105] -> w1081
              tunnel: w1078 -> [w1093 w1104]
              tunnel: w1077 -> [_ w1103]
              tunnel: w1076 -> [w1095 w1102]
              tunnel: w1075 -> [_ w1101]
              tunnel: ["Stopped" ("Test Status") w1098] -> w1073
              tunnel: w1068 -> [_ w1100]
              frame "Manual" {
                n511 = Flush Queue(queue=w1093, error in (no error)=w1095) -> (error out=w1094:errorcluster)  [unwired: 2 out]
              }
              frame "EFX Brake Torque", Default {
                n512 = case shown="True" w1101 {
                  tunnel: [w1109 w1115] -> w1105
                  tunnel: w1104 -> [w1108 w1118]
                  tunnel: w1103 -> [w1106 _]
                  tunnel: w1102 -> [w1107 w1119]
                  frame False {
                    n513 = for {
                      tunnel: w1108 -> [w1112]
                      tunnel: w1106 -> [w1110] mode=indexing
                      shift-right: [w1113] -> w1109
                      shift-left: w1107 -> [w1111]
                      n514 = Enqueue Element At Opposite End(queue=w1112, element=w1110, error in (no error)=w1111) -> (error out=w1113:errorcluster)  [unwired: 1 in, 2 out]
                    }
                  }
                  frame True {
                    n515 = Flush Queue(queue=w1118, error in (no error)=w1119) -> (queue out=w1117:refnum<queue>, error out=w1116:errorcluster)  [unwired: 1 out]
                    n516 = Enqueue Element At Opposite End(queue=w1117, element=T9 {"state"="Stop Test", "data"=variant}, error in (no error)=w1116) -> (error out=w1115:errorcluster)  [unwired: 1 in, 2 out]
                  }
                }
                n517 = Select(t="Running", s=w1100, f="Thermal Dwell" ("Test Status")) -> (s? t:f=w1098:string)
              }
            }
            n518 = local write "Test Status"(w1073) -> ()
          }
          frame "End Test" {
            # "Operations to be performed att he end of the test"
            n519 = Unbundle By Name(w1130) -> ("Queue Array"=w1129:T8, "Available Tests"=w1127:T2)
            n520 = Index Array(array=w1129) -> (element #1=w1128:refnum<queue>, element #2=w1122:refnum<queue>)  [unwired: 2 in]
            n521 = Flush Queue(queue=w1128, error in (no error)=w1125) -> (queue out=w1126:refnum<queue>, error out=w1124:errorcluster)  [unwired: 1 out]
            n522 = case shown="\"EFX Brake Torque\", Default" w1127 {
              selector: w1127 -> [_ w1144]
              tunnel: w1124 -> [w1132 w1156]
              tunnel: [w1132 w1151] -> w1131
              tunnel: w1126 -> [_ w1155]
              tunnel: w1122 -> [_ w1150]
              tunnel: T9 {"state"="", "data"=variant} ("element") -> [_ w1136]
              frame "Manual" {
              }
              frame "EFX Brake Torque", Default {
                n523 = Bundle By Name(cluster=w1136, "state"="Spin", "data"=cluster{"RPM":dbl, bool} {"RPM"=0.0, FALSE}) -> (w1153:T9)
                n524 = Enqueue Element(queue=w1155, element=w1153, error in (no error)=w1156) -> (queue out=w1154:refnum<queue>, error out=w1157:errorcluster)  [unwired: 1 in, 1 out]
                n525 = Bundle(cluster=w1136, "state"="Load Bank", "data"=Load_Bank."OFF" ("Load Bank")) -> (w1135:T9)
                n526 = Enqueue Element(queue=w1154, element=w1135, error in (no error)=w1157) -> (queue out=w1146:refnum<queue>, error out=w1142:errorcluster)  [unwired: 1 in, 1 out]
                n527 = Bundle(cluster=w1136, "state"="Ibrake", "data"="0" ("String")) -> (w1134:T9)
                n528 = Enqueue Element(queue=w1146, element=w1134, error in (no error)=w1142) -> (queue out=w1143:refnum<queue>, error out=w1141:errorcluster)  [unwired: 1 in, 1 out]
                n529 = Bundle By Name(cluster=T9 {"state"="Set UI", "data"=variant} ("element"), "data"=w1144) -> (w1145:T9)
                n530 = Enqueue Element(queue=w1143, element=w1145, error in (no error)=w1141) -> (error out=w1147:errorcluster)  [unwired: 1 in, 2 out]
                n531 = Enqueue Element At Opposite End(queue=w1150, element=T9 {"state"="End Test", "data"=variant}, error in (no error)=w1147) -> (error out=w1151:errorcluster)  [unwired: 1 in, 2 out]
              }
            }
            n532 = local write "Test Status"("Complete" ("Test Status")) -> ()
          }
          frame "Exit" {
            # "Shutdown case"
            n533 = Unbundle By Name(w1167) -> ("System Event"=w1165:refnum<user-event>, "Queue Array"=w1163:T8)
            n534 = Not Equal?(x=variant, y=w1169) -> (x != y?=w1168:bool)
            n535 = case shown="False" w1168 {
              tunnel: w1171 -> [w1173 w1178]
              tunnel: [w1173 w1177] -> w1160
              tunnel: w1169 -> [_ w1176]
              tunnel: [w1172 w1175] -> _
              tunnel: w1168 -> [w1172 w1174]
              frame False {
              }
              frame True {
                n536 = Variant To Data(error in=w1178, type=w1174, Variant=w1176) -> (data=w1175:bool, error out=w1177:errorcluster)
              }
            }
            n537 = Index Array(array=w1163, index=0) -> (element=w1161:refnum<queue>)
            n538 = Release Queue(queue=w1161, error in (no error)=w1160) -> (error out=w1159:errorcluster)  [unwired: 1 in, 2 out]
            n539 = Generate User Event(user event=w1165, event data cluster=T9 {"state"="Exit", "data"=variant} ("event data"), error in=w1159) -> (error out=w1166:errorcluster)  [unwired: 1 in, 1 out]
          }
          frame "Init" {
            # "prepare the system for operation"
            n540 = Unbundle By Name(w1214) -> ("Queue Array"=w1187:T8, "Channels"=w1192:string[])
            n541 = control-ref of="LPCA COM"() -> (w1194:refnum<vi>)
            n542 = Array Size(array=w1192) -> (size(s)=w1193:i32)
            n543 = Initialize Array(0 ("element"), w1193) -> (w1190:i32[])
            n544 = control-ref of="Thermal Limit"() -> (w1204:refnum<vi>)
            n545 = control-ref of="Thermal Resume"() -> (w1203:refnum<vi>)
            n546 = control-ref of="Stop Time"() -> (w1202:refnum<vi>)
            n547 = control-ref of="Sample Frequency"() -> (w1197:refnum<vi>)
            n548 = Index Array(array=w1187, index=0) -> (element=w1185:refnum<queue>)
            n549 = control-ref of="Load Sweep"() -> (w1201:refnum<vi>)
            n550 = control-ref of="RPM Sweep"() -> (w1200:refnum<vi>)
            n551 = control-ref of="Ibrake Sweep"() -> (w1199:refnum<vi>)
            n552 = control-ref of="Range Sweep"() -> (w1183:refnum<vi>)
            n553 = control-ref of="Step Height Sweep"() -> (w1184:refnum<vi>)
            n554 = control-ref of="Filters"() -> (w1198:refnum<vi>)
            n555 = property on="Available Tests" class="Enum (strict)"(error in=w1188, "Val(Sgnl)"=Available_Tests."Manual" ("Available Tests")) -> (error out=w1212:errorcluster)  [unwired: 1 in, 1 out]
            n556 = Build Array(w1204, w1203, w1202, w1201, w1200, w1199, w1183, w1184, w1198, w1197, w1194) -> (w1196:refnum<vi>[])
            n557 = property on="Data Setup" class="MCListbox (strict)"(error in=w1212, "ItemSyms"=w1190) -> (error out=w1182:errorcluster)  [unwired: 1 in, 1 out]
            n558 = property on="Thermal Equilibrium" class="Bool (strict)"(error in=w1182, "Val(Sgnl)"=FALSE ("Value (Signaling)")) -> (error out=w1181:errorcluster)  [unwired: 1 in, 1 out]
            n559 = Bundle By Name(cluster=T9 {"state"="Load Bank", "data"=variant} ("element"), "data"=u16 0) -> (w1207:T9)
            n560 = Bundle By Name(cluster=w1214, "Current RPM"=0.0, "Cfg Cntrls"=w1196) -> (w1213:T7)
            n561 = Build Array(T9 {"state"="init LPCA", "data"=variant} ("element"), w1207, T9 {"state"="load config", "data"=variant} ("element")) -> (w1205:T9[])
            n562 = for {
              tunnel: w1181 -> [w1218]
              tunnel: [w1217] -> w1211
              tunnel: w1205 -> [w1216] mode=indexing
              tunnel: w1185 -> [w1215]
              n563 = Enqueue Element(queue=w1215, element=w1216, error in (no error)=w1218) -> (error out=w1217:errorcluster)  [unwired: 1 in, 2 out]
            }
          }
          frame "init LPCA" {
            # "Fire the initialization of the LPCA"
            n564 = Not Equal?(x=variant, y=w1233) -> (x != y?=w1232:bool)
            n565 = case shown="False" w1232 {
              tunnel: w1235 -> [w1237 w1242]
              tunnel: [w1237 w1241] -> w1226
              tunnel: w1233 -> [_ w1240]
              tunnel: [w1236 w1239] -> w1220
              tunnel: "LPCA COM" -> [w1236 w1238]
              frame False {
              }
              frame True {
                n566 = Variant To Data(error in=w1242, type=w1238, Variant=w1240) -> (data=w1239:refnum<visa-resource-name>, error out=w1241:errorcluster)
              }
            }
            n567 = Unbundle By Name(w1223) -> ("Queue Array"=w1227:T8, "Queue Element"=w1229:T9)
            n568 = To Variant(anything=w1220) -> (Variant=w1231:variant)
            n569 = Bundle By Name(cluster=w1229, "state"="init com", "data"=w1231) -> (w1230:T9)
            n570 = Index Array(array=w1227, index=4) -> (element=w1228:refnum<queue>)
            n571 = Enqueue Element(queue=w1228, element=w1230, error in (no error)=w1226) -> (error out=w1225:errorcluster)  [unwired: 1 in, 2 out]
          }
          frame "Load Bank" {
            # "Set the load bank"
            n572 = Unbundle By Name(w1249) -> ("Queue Array"=w1248:T8, "Queue Element"=w1247:T9, "Load Bank"=w1245:T3)
            n573 = Not Equal?(x=variant, y=w1258) -> (x != y?=w1257:bool)
            n574 = case shown="True" w1257 {
              tunnel: w1260 -> [w1262 w1267]
              tunnel: [w1262 w1266] -> w1256
              tunnel: w1258 -> [_ w1265]
              tunnel: [w1261 w1264] -> w1246
              tunnel: w1245 -> [w1261 w1263]
              frame False {
              }
              frame True {
                n575 = Variant To Data(error in=w1267, type=w1263, Variant=w1265) -> (data=w1264:T3, error out=w1266:errorcluster)
              }
            }
            n576 = call "Set Load.vi"("error in (no error)"=w1256, "Boolean"=FALSE, "Numeric"=w1246) -> ("error out"=w1251:errorcluster)  [unwired: 8 in]
            n577 = local write "Load Bank"(w1246) -> ()
            n578 = Bundle By Name(cluster=w1247, "state"="update load", "data"=w1246) -> (w1253:T9)
            n579 = Index Array(array=w1248, index=1) -> (element=w1255:refnum<queue>)
            n580 = Enqueue Element At Opposite End(queue=w1255, element=w1253, error in (no error)=w1251) -> (error out=w1250:errorcluster)  [unwired: 1 in, 2 out]
          }
          frame "FanMode" {
            # "Update FanMode & Fan Mode Array.  Comunicate to Acquisistion Thread"
            n581 = Unbundle By Name(w1278) -> ("Queue Array"=w1277:T8, "Queue Element"=w1275:T9, "FanMode"=w1272:T11)
            n582 = Not Equal?(x=variant, y=w1280) -> (x != y?=w1279:bool)
            n583 = case shown="True" w1279 {
              tunnel: w1282 -> [w1338 w1343]
              tunnel: [w1338 w1342] -> w1273
              tunnel: w1280 -> [_ w1341]
              tunnel: [w1337 w1340] -> w1270
              tunnel: w1272 -> [w1337 w1339]
              frame False {
              }
              frame True {
                n584 = Variant To Data(error in=w1343, type=w1339, Variant=w1341) -> (data=w1340:T11, error out=w1342:errorcluster)
              }
            }
            n585 = Not Equal?(x=w1272, y=w1270) -> (x != y?=w1271:bool)
            n586 = case shown="True" w1271 {
              tunnel: w1277 -> [_ w1290]
              tunnel: w1275 -> [_ w1289]
              tunnel: [w1284 w1287] -> w1274
              tunnel: w1273 -> [w1284 w1288]
              tunnel: w1270 -> [_ w1286]
              tunnel: [w1283 w1285] -> w1269
              frame False {
                n587 = local read "Fan Mode LED Array"() -> (w1283:bool[])
              }
              frame True {
                n588 = case shown="\"Auto\"" w1286 {
                  tunnel: w1290 -> [w1301 w1316 w1333]
                  tunnel: w1289 -> [w1300 w1315 w1332]
                  tunnel: w1288 -> [w1299 w1314 w1331]
                  tunnel: w1286 -> [w1298 w1313 w1330]
                  tunnel: [w1297 w1312 w1322] -> w1287
                  tunnel: [w1291 w1306 w1327] -> w1285
                  frame "Off", Default {
                    n589 = Bundle By Name(cluster=w1300, "state"="update FanMode", "data"=w1298) -> (w1303:T9)
                    n590 = Index Array(array=w1301, index=1) -> (element=w1305:refnum<queue>)
                    n591 = local read "Fan Mode LED Array"() -> (w1296:bool[])
                    n592 = Enqueue Element(queue=w1305, element=w1303, error in (no error)=w1299) -> (error out=w1297:errorcluster)  [unwired: 1 in, 2 out]
                    n593 = Replace Array Subset(array=w1296, new element #1=FALSE ("new element/subarray"), index #1=FanMode."On" ("FanMode"), new element #2=TRUE ("new element/subarray"), index #2=FanMode."Off" ("FanMode")) -> (w1291:bool[])
                  }
                  frame "On" {
                    n594 = Bundle By Name(cluster=w1315, "state"="update FanMode", "data"=w1313) -> (w1318:T9)
                    n595 = Index Array(array=w1316, index=1) -> (element=w1320:refnum<queue>)
                    n596 = local read "Fan Mode LED Array"() -> (w1311:bool[])
                    n597 = Enqueue Element(queue=w1320, element=w1318, error in (no error)=w1314) -> (error out=w1312:errorcluster)  [unwired: 1 in, 2 out]
                    n598 = Replace Array Subset(array=w1311, new element #1=TRUE ("new element/subarray"), index #1=FanMode."On" ("FanMode"), new element #2=FALSE ("new element/subarray"), index #2=FanMode."Off" ("FanMode")) -> (w1306:bool[])
                  }
                  frame "Auto" {
                    n599 = Bundle By Name(cluster=w1332, "state"="update FanMode", "data"=w1330) -> (w1326:T9)
                    n600 = Index Array(array=w1333, index=1) -> (element=w1336:refnum<queue>)
                    n601 = Unbundle By Name(w1326) -> ("data"=w1325:variant)
                    n602 = Enqueue Element(queue=w1336, element=w1326, error in (no error)=w1331) -> (error out=w1323:errorcluster)  [unwired: 1 in, 2 out]
                    n603 = local read "Fan Mode LED Array"() -> (w1329:bool[])
                    n604 = Variant To Data(error in=w1323, type=TRUE, Variant=w1325) -> (data=w1321:bool, error out=w1322:errorcluster)
                    n605 = Replace Array Subset(array=w1329, new element=w1321, index=FanMode."Auto" ("FanMode")) -> (w1327:bool[])
                  }
                }
              }
            }
            n606 = Bundle By Name(cluster=w1278, "FanMode"=w1270, "Fan Mode LED Array"=w1269) -> (w1276:T7)
            n607 = local write "Fan Mode LED Array"(w1269) -> ()
          }
          frame "Thermal Equilibrium" {
            # "Update Thermal Equilibrium Test Mode.  Comunicate to Acquisistion Thread"
            n608 = Unbundle By Name(w1358) -> ("Queue Array"=w1346:T8, "Queue Element"=w1345:T9, "Thermal\nEquilibrium"=w1357:bool)
            n609 = Not Equal?(x=variant, y=w1364) -> (x != y?=w1363:bool)
            n610 = case shown="True" w1363 {
              tunnel: w1366 -> [w1368 w1373]
              tunnel: [w1368 w1372] -> w1354
              tunnel: w1364 -> [_ w1371]
              tunnel: [w1367 w1370] -> w1355
              tunnel: w1357 -> [w1367 w1369]
              frame False {
              }
              frame True {
                n611 = Variant To Data(error in=w1373, type=w1369, Variant=w1371) -> (data=w1370:bool, error out=w1372:errorcluster)
              }
            }
            n612 = Bundle By Name(cluster=w1345, "state"="update Thermal Equilibrium", "data"=w1355) -> (w1360:T9)
            n613 = Index Array(array=w1346, index #1=1 ("index"), index #2=0 ("index")) -> (element #1=w1362:refnum<queue>, element #2=w1348:refnum<queue>)
            n614 = local read "Available Tests"() -> (w1350:T2)
            n615 = Enqueue Element At Opposite End(queue=w1362, element=w1360, error in (no error)=w1354) -> (error out=w1353:errorcluster)  [unwired: 1 in, 2 out]
            n616 = Bundle By Name(cluster=w1358, "Thermal\nEquilibrium"=w1355) -> (w1356:T7)
            n617 = Bundle By Name(cluster=w1345, "state"="set ui", "data"=w1350) -> (w1347:T9)
            n618 = Enqueue Element(queue=w1348, element=w1347, error in (no error)=w1353) -> (error out=w1352:errorcluster)  [unwired: 1 in, 2 out]
          }
          frame "load config" {
            # "Load a configuration from file"
            n619 = call <vilib>:"Application Directory.vi"() -> ("Application Directory"=w1390:path)
            n620 = Build Path(base path=w1390, name or relative path="data") -> (appended path=w1388:path)
            n621 = Equal?(x=variant, y=w1392) -> (x = y?=w1391:bool)
            n622 = Build Path(base path=w1388, name or relative path="lastcfg.ini") -> (appended path=w1385:path)
            n623 = case shown="False" w1391 {
              tunnel: w1394 -> [w1431 w1433]
              tunnel: [w1430 w1433] -> w1379
              tunnel: w1392 -> [w1429 _]
              tunnel: [w1428 w1432] -> w1377
              tunnel: w1385 -> [w1427 w1432]
              frame False {
                n624 = Variant To Data(error in=w1431, type=w1427, Variant=w1429) -> (data=w1428:path, error out=w1430:errorcluster)
              }
              frame True {
              }
            }
            n625 = Unbundle By Name(w1386) -> ("Queue Array"=w1382:T8, "Cfg Cntrls"=w1384:refnum<vi>[])
            n626 = call <vilib>:"Check if File or Folder Exists.vi"("error in (no error)"=w1379, "path"=w1377) -> ("error out"=w1376:errorcluster, "file or folder exists?"=w1375:bool, "dup path"=w1378:path)  [unwired: 7 in]
            n627 = Index Array(array=w1382, index=1) -> (element=w1381:refnum<queue>)
            n628 = case shown="True" w1375 {
              tunnel: w1384 -> [_ w1414]
              tunnel: [w1395 w1406] -> w1383
              tunnel: w1381 -> [_ w1405]
              tunnel: w1378 -> [_ w1401]
              tunnel: w1376 -> [w1395 w1400]
              frame False {
              }
              frame True {
                w1407 = "config"
                n629 = call "Config to DB Data.vi"("error in (no error)"=w1400, "Control References Array"=w1414) -> ("error out"=w1418:errorcluster, "Name"=w1417:string[])  [unwired: 7 in, 1 out]
                n630 = property on="Data Setup" class="MCListbox (strict)"() -> ("Label.Text"=w1411:string)  [unwired: 2 in, 2 out]
                n631 = call <vilib>:"Open Config Data.vi"("error in (no error)"=w1418, "configuration file path"=w1401) -> ("error out"=w1412:errorcluster, "refnum"=w1410:T19)  [unwired: 7 in, 1 out]
                n632 = call-poly <vilib>:"Read Key.vi"("section"=w1407, "error in (no error)"=w1412, "key"=w1411, "refnum"=w1410) -> ("error out"=w1399:errorcluster, "value"=w1408:string, "refnum out"=w1409:T19)  [unwired: 4 in, 1 out]
                n633 = call "dbase string to variant.vi"("error in (no error)"=w1399, "String"=w1408) -> ("error out"=w1398:errorcluster, "Variant"=w1402:variant)  [unwired: 8 in]
                n634 = for {
                  tunnel: w1409 -> [w1425]
                  tunnel: w1417 -> [w1424] mode=indexing
                  tunnel: w1407 -> [w1423]
                  tunnel: [w1421] -> w1415
                  tunnel: [w1419] -> w1413 mode=indexing
                  shift-right: [w1422] -> w1416
                  shift-left: w1398 -> [w1426]
                  n635 = call-poly <vilib>:"Read Key.vi"("section"=w1423, "error in (no error)"=w1426, "key"=w1424, "refnum"=w1425) -> ("error out"=w1422:errorcluster, "value"=w1420:string, "refnum out"=w1421:T19)  [unwired: 4 in, 1 out]
                  n636 = call <vilib>:"Trim Whitespace.vi"("string"=w1420) -> ("trimmed string"=w1419:string)  [unwired: 1 in]
                }
                n637 = call <vilib>:"Close Config Data.vi"("error in (no error)"=w1416, "refnum"=w1415) -> ("error out"=w1397:errorcluster)  [unwired: 8 in, 1 out]
                n638 = call "Load db Config Data to Controls.vi"("error in (no error)"=w1397, "Control References Array"=w1414, "Data"=w1413) -> ("error out"=w1396:errorcluster)  [unwired: 8 in]
                n639 = Bundle By Name(cluster=T9 {"state"="update table", "data"=variant} ("element"), "data"=w1402) -> (w1403:T9)
                n640 = Enqueue Element At Opposite End(queue=w1405, element=w1403, error in (no error)=w1396) -> (error out=w1406:errorcluster)  [unwired: 1 in, 2 out]
              }
            }
          }
          frame "load sweep" {
            # "Pass the sweep into the cluster"
            n641 = Not Equal?(x=variant, y=w1445) -> (x != y?=w1444:bool)
            n642 = case shown="False" w1444 {
              tunnel: w1447 -> [w1449 w1454]
              tunnel: [w1449 w1453] -> w1442
              tunnel: w1445 -> [_ w1452]
              tunnel: [w1448 w1451] -> w1441
              tunnel: "0" -> [w1448 w1450]
              frame False {
              }
              frame True {
                n643 = Variant To Data(error in=w1454, type=w1450, Variant=w1452) -> (data=w1451:string, error out=w1453:errorcluster)
              }
            }
            n644 = Unbundle By Name(w1436) -> ("Load Sweep"=w1435:string[])
            n645 = Spreadsheet String To Array(delimiter (Tab)=",", format string="", spreadsheet string=w1441, array type (2D Dbl)=w1435) -> (array=w1437:string[])
            n646 = Bundle By Name(cluster=w1436, "Load Sweep"=w1437) -> (w1438:T7)
          }
          frame "Next test" {
            # "Controls the counter that keeps track of the secuencing"
            n647 = Unbundle By Name(w1476) -> ("A Counter"=w1477:i32, "#A"=w1478:i32, "B Counter"=w1474:i32, "#B"=w1460:i32, "C Counter"=w1459:i32, "#C"=w1458:i32, "Queue Array"=w1472:T8, "Available Tests"=w1468:T2)
            n648 = Bundle By Name(cluster=T9 {"state"="autotest", "data"=variant} ("element"), "data"=FALSE) -> (w1463:T9)
            n649 = Index Array(array=w1472) -> (element #1=w1471:refnum<queue>, element #2=w1465:refnum<queue>)  [unwired: 2 in]
            n650 = Enqueue Element At Opposite End(queue=w1465, element=w1463, error in (no error)=w1467) -> (error out=w1466:errorcluster)  [unwired: 1 in, 2 out]
            n651 = call "Test Counter.vi"("#C"=w1458, "C Counter"=w1459, "#B"=w1460, "B Counter"=w1474, "#A"=w1478, "A Counter in"=w1477) -> ("Next (T)"=w1461:bool, "C Counter out"=w1457:i32, "B Counter out"=w1469:i32, "A Counter out"=w1470:i32)  [unwired: 2 in]
            n652 = case shown="True" w1461 {
              tunnel: [w1482 w1487] -> w1473
              tunnel: w1466 -> [w1481 w1486]
              tunnel: w1471 -> [w1480 w1485]
              tunnel: w1468 -> [_ w1483]
              frame False {
                n653 = Enqueue Element(queue=w1480, element=T9 {"state"="End Test", "data"=variant}, error in (no error)=w1481) -> (error out=w1482:errorcluster)  [unwired: 1 in, 2 out]
              }
              frame True {
                n654 = case shown="\"EFX Brake Torque\", \"Generator Torque\", \"AMT Brake Torque\", \"Bike Brake Torque\"" w1483 {
                  tunnel: [T9 {"state"="", "data"=variant} ("element") T9 {"state"="", "data"=variant} ("element") T9 {"state"="Check Temp", "data"=variant} ("element") T9 {"state"="dwell for resume", "data"=variant} ("element")] -> w1484
                  frame "Manual" {
                  }
                  frame "Pulsed RPM" {
                  }
                  frame "EFX Brake Torque", "Generator Torque", "AMT Brake Torque", "Bike Brake Torque" {
                  }
                  frame "EFX Brake Thermal", "Generator Thermal", "AMT Brake Thermal", "Bike Brake Thermal" {
                  }
                }
                n655 = Enqueue Element(queue=w1485, element=w1484, error in (no error)=w1486) -> (error out=w1487:errorcluster)  [unwired: 1 in, 2 out]
              }
            }
            n656 = Bundle By Name(cluster=w1476, "A Counter"=w1470, "B Counter"=w1469, "C Counter"=w1457, "Timer Reset"=TRUE) -> (w1475:T7)
          }
          frame "Over Temp", "Pause Test" {
            # "Wait for pt. \nto pause"
            # "Pause stops the test by dumping the remaining sequence elements. Resume picks up at the next test."
            n657 = local read "Capture"() -> (w1501:bool)
            n658 = Not Equal?(x=variant, y=w1511) -> (x != y?=w1510:bool)
            n659 = case shown="True" w1510 {
              tunnel: w1514 -> [w1551 w1556]
              tunnel: [w1551 w1555] -> w1513
              tunnel: w1511 -> [_ w1554]
              tunnel: [w1550 w1553] -> w1496
              tunnel: w1510 -> [w1550 w1552]
              frame False {
              }
              frame True {
                n660 = Variant To Data(error in=w1556, type=w1552, Variant=w1554) -> (data=w1553:bool, error out=w1555:errorcluster)
              }
            }
            n661 = Unbundle By Name(w1509) -> ("Queue Array"=w1508:T8, "Available Tests"=w1495:T2)
            n662 = case shown="\"Over Temp\"" w1492 {
              tunnel: "Paused" -> [w1515 w1518]
              tunnel: [w1515 w1517] -> w1497
              frame "False", Default {
              }
              frame "Over Temp" {
                n663 = Concatenate Strings(w1518, ":Thermal Limit" ("string")) -> (w1517:string)
              }
            }
            n664 = feedback-in #1(w1501) -> ()
            n665 = feedback #1() -> (w1503:bool)  [unwired: 1 in]
            n666 = feedback-in #2(w1492) -> ()
            n667 = feedback #2("") -> (w1493:string)
            n668 = Not Equal?(x=w1501, y=w1503) -> (x != y?=w1502:bool)
            n669 = local read "Stop Test"() -> (w1499:bool)
            n670 = Not Equal?(x=w1492, y=w1493) -> (x != y?=w1504:bool)
            n671 = And(x=w1501, y=w1502) -> (x .and. y?=w1500:bool)
            n672 = Index Array(array=w1508) -> (element=w1506:refnum<queue>)  [unwired: 1 in]
            n673 = local write "Test Status"(w1497) -> ()
            n674 = case shown="True" w1496 {
              selector: w1496 -> [_ w1528]
              tunnel: w1513 -> [w1522 w1540]
              tunnel: [w1521 w1538] -> w1507
              tunnel: w1506 -> [w1520 w1539]
              tunnel: w1504 -> [_ w1537]
              tunnel: w1500 -> [_ _]
              tunnel: w1499 -> [w1519 _]
              tunnel: w1495 -> [_ w1530]
              frame False {
                n675 = case shown="False" w1519 {
                  tunnel: w1522 -> [w1526 w1527]
                  tunnel: [w1525 w1527] -> w1521
                  tunnel: w1520 -> [w1524 _]
                  frame False {
                    n676 = Enqueue Element At Opposite End(queue=w1524, element=T9 {"state"="next test", "data"=variant}, error in (no error)=w1526) -> (error out=w1525:errorcluster)  [unwired: 1 in, 2 out]
                  }
                  frame True {
                  }
                }
              }
              frame True {
                (unwired) T9 {"state"="Load Bank", "data"=variant} ("element")
                (unwired) T9 {"state"="Ibrake", "data"=variant} ("element")
                n677 = Flush Queue(queue=w1539, error in (no error)=w1540) -> (queue out=w1532:refnum<queue>, error out=w1533:errorcluster)  [unwired: 1 out]
                n678 = case shown="\"EFX Brake Torque\", \"AMT Brake Torque\"" w1530 {
                  tunnel: [T9 {"state"="", "data"=variant} ("element") T9 {"state"="Check Temp", "data"=variant} ("element") T9 {"state"="Check Temp", "data"=variant} ("element") T9 {"state"="dwell for resume", "data"=variant} ("element") T9 {"state"="dwell for resume", "data"=variant} ("element")] -> w1529
                  frame "Manual", Default {
                  }
                  frame "EFX Brake Torque", "AMT Brake Torque" {
                  }
                  frame "Generator Torque" {
                  }
                  frame "Bike Brake Torque" {
                  }
                  frame "Generator Thermal" {
                  }
                }
                n679 = And(x=w1528, y=w1537) -> ()  [unwired: 1 out]
                n680 = local write "Snapshot"(w1528) -> ()
                n681 = Bundle By Name(cluster=T9 {"state"="Spin", "data"=variant} ("element"), "data"=cluster{"RPM":dbl, bool} {"RPM"=0.0, FALSE}) -> (w1535:T9)
                n682 = Build Array(w1535, w1529) -> (w1534:T9[])
                n683 = for {
                  tunnel: w1532 -> [w1549]
                  tunnel: w1533 -> [w1548]
                  tunnel: [w1547] -> w1538
                  tunnel: w1534 -> [w1546] mode=indexing
                  n684 = Enqueue Element(queue=w1549, element=w1546, error in (no error)=w1548) -> (error out=w1547:errorcluster)  [unwired: 1 in, 2 out]
                }
              }
            }
          }
          frame "PreStart Dwell" {
            # "Wait for the test conditions to be correct for starting"
            n685 = Not Equal?(x=variant, y=w1584) -> (x != y?=w1583:bool)
            n686 = Unbundle By Name(w1566) -> ("Queue Array"=w1578:T8, "A Counter"=w1576:i32, "B Counter"=w1577:i32, "C Counter"=w1559:i32, "Stop Time"=w1560:dbl, "Timer Reset"=w1563:bool)
            n687 = case shown="True" w1583 {
              selector: w1583 -> [w1592 _]
              tunnel: w1586 -> [w1593 w1598]
              tunnel: [w1593 w1597] -> w1580
              tunnel: w1584 -> [_ w1596]
              tunnel: [w1592 w1595] -> _
              tunnel: w1583 -> [_ w1594]
              frame False {
              }
              frame True {
                n688 = Variant To Data(error in=w1598, type=w1594, Variant=w1596) -> (data=w1595:bool, error out=w1597:errorcluster)
              }
            }
            n689 = call "Elapsed Time"("Time Target (s)"=w1560, "Reset"=w1563, "Auto Reset"=TRUE, "error in (no error)"=w1580) -> ("Time has Elapsed"=w1561:bool, "error out"=w1574:errorcluster)  [unwired: 8 in, 6 out]
            n690 = Bundle("A Counter"=w1576, "B Counter"=w1577, "C Counter"=w1559) -> (w1581:T22)  [unwired: 1 in]
            n691 = Index Array(array=w1578, index #1=1 ("index"), index #2=0 ("index")) -> (element #1=w1568:refnum<queue>, element #2=w1569:refnum<queue>)
            n692 = Bundle By Name(cluster=T9 {"state"="Start Test", "data"=variant} ("element"), "data"=w1581) -> (w1572:T9)
            n693 = local read "Stop Test"() -> (w1565:bool)
            n694 = Select(t=w1568, s=w1561, f=w1569) -> (s? t:f=w1567:refnum<queue>)
            n695 = Select(t=w1572, s=w1561, f=T9 {"state"="PreStart Dwell", "data"=variant} ("element")) -> (s? t:f=w1571:T9)
            n696 = case shown="False" w1565 {
              tunnel: [w1590 w1591] -> w1579
              tunnel: w1574 -> [w1589 w1591]
              tunnel: w1571 -> [w1588 _]
              tunnel: w1567 -> [w1587 _]
              frame False {
                n697 = Enqueue Element At Opposite End(queue=w1587, element=w1588, error in (no error)=w1589) -> (error out=w1590:errorcluster)  [unwired: 1 in, 2 out]
              }
              frame True {
              }
            }
            n698 = Bundle By Name(cluster=w1566, "Timer Reset"=FALSE) -> (w1562:T7)
          }
          frame "Ibrake" {
            # "Set the resistance"
            n699 = Not Equal?(x=variant, y=w1622) -> (x != y?=w1621:bool)
            n700 = case shown="True" w1621 {
              tunnel: w1624 -> [w1626 w1631]
              tunnel: [w1626 w1630] -> w1616
              tunnel: w1622 -> [_ w1629]
              tunnel: [w1625 w1628] -> w1601
              tunnel: "1" -> [w1625 w1627]
              frame False {
              }
              frame True {
                n701 = Variant To Data(error in=w1631, type=w1627, Variant=w1629) -> (data=w1628:string, error out=w1630:errorcluster)
              }
            }
            n702 = Hexadecimal String To Number(string=w1601) -> (number=w1600:u32)  [unwired: 2 in, 1 out]
            n703 = local write "Ibrake"(w1600) -> ()
            n704 = Bundle("LPCA Command"=LPCA_Commands."mamp", w1601) -> (w1613:cluster{"LPCA Command":T20, string})  [unwired: 1 in]
            n705 = Unbundle By Name(w1612) -> ("Queue Array"=w1604:T8, "Queue Element"=w1603:T9)
            n706 = To Variant(anything=w1613) -> (Variant=w1619:variant)
            n707 = Bundle By Name(cluster=w1603, "state"="set", "data"=w1619) -> (w1618:T9)
            n708 = Index Array(array=w1604, index=4) -> (element=w1617:refnum<queue>)
            n709 = Enqueue Element At Opposite End(queue=w1617, element=w1618, error in (no error)=w1616) -> (error out=w1606:errorcluster)  [unwired: 1 in, 2 out]
            n710 = Bundle By Name(cluster=w1612, "Current Ibrake"=w1600) -> (w1602:T7)
            n711 = Bundle By Name(cluster=w1603, "state"="update Ibrake", "data"=w1601) -> (w1608:T9)
            n712 = Index Array(array=w1604, index=1) -> (element=w1610:refnum<queue>)
            n713 = Enqueue Element At Opposite End(queue=w1610, element=w1608, error in (no error)=w1606) -> (error out=w1605:errorcluster)  [unwired: 1 in, 2 out]
          }
          frame "Range" {
            # "Set the resistance"
            n714 = Not Equal?(x=variant, y=w1655) -> (x != y?=w1654:bool)
            n715 = case shown="True" w1654 {
              tunnel: w1657 -> [w1659 w1664]
              tunnel: [w1659 w1663] -> w1649
              tunnel: w1655 -> [_ w1662]
              tunnel: [w1658 w1661] -> w1634
              tunnel: "2" -> [w1658 w1660]
              frame False {
              }
              frame True {
                n716 = Variant To Data(error in=w1664, type=w1660, Variant=w1662) -> (data=w1661:string, error out=w1663:errorcluster)
              }
            }
            n717 = Hexadecimal String To Number(string=w1634) -> (number=w1633:u32)  [unwired: 2 in, 1 out]
            n718 = local write "Range"(w1633) -> ()
            n719 = Bundle("LPCA Command"=LPCA_Commands."rng", w1634) -> (w1646:cluster{"LPCA Command":T20, string})  [unwired: 1 in]
            n720 = Unbundle By Name(w1645) -> ("Queue Array"=w1637:T8, "Queue Element"=w1636:T9)
            n721 = To Variant(anything=w1646) -> (Variant=w1652:variant)
            n722 = Bundle By Name(cluster=w1636, "state"="set", "data"=w1652) -> (w1651:T9)
            n723 = Index Array(array=w1637, index=4) -> (element=w1650:refnum<queue>)
            n724 = Enqueue Element At Opposite End(queue=w1650, element=w1651, error in (no error)=w1649) -> (error out=w1639:errorcluster)  [unwired: 1 in, 2 out]
            n725 = Bundle By Name(cluster=w1645, "Current Range"=w1633) -> (w1635:T7)
            n726 = Bundle By Name(cluster=w1636, "state"="update range", "data"=w1634) -> (w1641:T9)
            n727 = Index Array(array=w1637, index=1) -> (element=w1643:refnum<queue>)
            n728 = Enqueue Element At Opposite End(queue=w1643, element=w1641, error in (no error)=w1639) -> (error out=w1638:errorcluster)  [unwired: 1 in, 2 out]
          }
          frame "Step Height" {
            # "Set the step hieight"
            n729 = Not Equal?(x=variant, y=w1688) -> (x != y?=w1687:bool)
            n730 = case shown="True" w1687 {
              tunnel: w1690 -> [w1692 w1697]
              tunnel: [w1692 w1696] -> w1682
              tunnel: w1688 -> [_ w1695]
              tunnel: [w1691 w1694] -> w1667
              tunnel: "2" -> [w1691 w1693]
              frame False {
              }
              frame True {
                n731 = Variant To Data(error in=w1697, type=w1693, Variant=w1695) -> (data=w1694:string, error out=w1696:errorcluster)
              }
            }
            n732 = Hexadecimal String To Number(string=w1667) -> (number=w1666:u32)  [unwired: 2 in, 1 out]
            n733 = local write "Step Height"(w1666) -> ()
            n734 = Bundle("LPCA Command"=LPCA_Commands."ramp", w1667) -> (w1679:cluster{"LPCA Command":T20, string})  [unwired: 1 in]
            n735 = Unbundle By Name(w1678) -> ("Queue Array"=w1670:T8, "Queue Element"=w1669:T9)
            n736 = To Variant(anything=w1679) -> (Variant=w1685:variant)
            n737 = Bundle By Name(cluster=w1669, "state"="set", "data"=w1685) -> (w1684:T9)
            n738 = Index Array(array=w1670, index=4) -> (element=w1683:refnum<queue>)
            n739 = Enqueue Element At Opposite End(queue=w1683, element=w1684, error in (no error)=w1682) -> (error out=w1672:errorcluster)  [unwired: 1 in, 2 out]
            n740 = Bundle By Name(cluster=w1678, "Current Step Height"=w1666) -> (w1668:T7)
            n741 = Bundle By Name(cluster=w1669, "state"="update Step Height", "data"=w1667) -> (w1674:T9)
            n742 = Index Array(array=w1670, index=1) -> (element=w1676:refnum<queue>)
            n743 = Enqueue Element At Opposite End(queue=w1676, element=w1674, error in (no error)=w1672) -> (error out=w1671:errorcluster)  [unwired: 1 in, 2 out]
          }
          frame "Ibrake Sweep" {
            # "Pass in the values of the resistance sweep"
            n744 = Not Equal?(x=variant, y=w1711) -> (x != y?=w1710:bool)
            n745 = Unbundle By Name(w1703) -> ("Ibrake Sweep"=w1702:string[])
            n746 = case shown="True" w1710 {
              tunnel: w1713 -> [w1715 w1720]
              tunnel: [w1715 w1719] -> w1708
              tunnel: w1711 -> [_ w1718]
              tunnel: [w1714 w1717] -> w1707
              tunnel: "0" -> [w1714 w1716]
              frame False {
              }
              frame True {
                n747 = Variant To Data(error in=w1720, type=w1716, Variant=w1718) -> (data=w1717:string, error out=w1719:errorcluster)
              }
            }
            n748 = Spreadsheet String To Array(delimiter (Tab)=",", format string="", spreadsheet string=w1707, array type (2D Dbl)=w1702) -> (array=w1700:string[])
            n749 = Decimal String To Number(string=w1700) -> (number=w1701:i32[])  [unwired: 2 in, 1 out]
            n750 = Number To Hexadecimal String(2:w1701) -> (0:w1699:string[])  [unwired: 1 in]
            n751 = Bundle By Name(cluster=w1703, "Ibrake Sweep"=w1699) -> (w1704:T7)
          }
          frame "Range Sweep" {
            # "Pass in the values of the resistance sweep"
            n752 = Not Equal?(x=variant, y=w1734) -> (x != y?=w1733:bool)
            n753 = Unbundle By Name(w1726) -> ("Range Sweep"=w1725:string[])
            n754 = case shown="True" w1733 {
              tunnel: w1736 -> [w1738 w1743]
              tunnel: [w1738 w1742] -> w1731
              tunnel: w1734 -> [_ w1741]
              tunnel: [w1737 w1740] -> w1730
              tunnel: "0" -> [w1737 w1739]
              frame False {
              }
              frame True {
                n755 = Variant To Data(error in=w1743, type=w1739, Variant=w1741) -> (data=w1740:string, error out=w1742:errorcluster)
              }
            }
            n756 = Spreadsheet String To Array(delimiter (Tab)=",", format string="", spreadsheet string=w1730, array type (2D Dbl)=w1725) -> (array=w1723:string[])
            n757 = Decimal String To Number(string=w1723) -> (number=w1724:i32[])  [unwired: 2 in, 1 out]
            n758 = Number To Hexadecimal String(2:w1724) -> (0:w1722:string[])  [unwired: 1 in]
            n759 = Bundle By Name(cluster=w1726, "Range Sweep"=w1722) -> (w1727:T7)
          }
          frame "Step Height Sweep" {
            # "Pass in the values of the Step Height sweep"
            n760 = Not Equal?(x=variant, y=w1757) -> (x != y?=w1756:bool)
            n761 = case shown="True" w1756 {
              tunnel: w1759 -> [w1761 w1766]
              tunnel: [w1761 w1765] -> w1754
              tunnel: w1757 -> [_ w1764]
              tunnel: [w1760 w1763] -> w1753
              tunnel: "0" -> [w1760 w1762]
              frame False {
              }
              frame True {
                n762 = Variant To Data(error in=w1766, type=w1762, Variant=w1764) -> (data=w1763:string, error out=w1765:errorcluster)
              }
            }
            n763 = Unbundle By Name(w1749) -> ("Step Height Sweep"=w1748:string[])
            n764 = Spreadsheet String To Array(delimiter (Tab)=",", format string="", spreadsheet string=w1753, array type (2D Dbl)=w1748) -> (array=w1746:string[])
            n765 = Decimal String To Number(string=w1746) -> (number=w1747:i32[])  [unwired: 2 in, 1 out]
            n766 = Number To Hexadecimal String(2:w1747) -> (0:w1745:string[])  [unwired: 1 in]
            n767 = Bundle By Name(cluster=w1749, "Step Height Sweep"=w1745) -> (w1750:T7)
          }
          frame "rpm sweep" {
            # "Pass in the rpm sweet"
            n768 = Not Equal?(x=variant, y=w1778) -> (x != y?=w1777:bool)
            n769 = case shown="False" w1777 {
              tunnel: w1780 -> [w1782 w1787]
              tunnel: [w1782 w1786] -> w1775
              tunnel: w1778 -> [_ w1785]
              tunnel: [w1781 w1784] -> w1774
              tunnel: "0" -> [w1781 w1783]
              frame False {
              }
              frame True {
                n770 = Variant To Data(error in=w1787, type=w1783, Variant=w1785) -> (data=w1784:string, error out=w1786:errorcluster)
              }
            }
            n771 = Unbundle By Name(w1769) -> ("RPM Sweep"=w1768:string[])
            n772 = Spreadsheet String To Array(delimiter (Tab)=",", format string="", spreadsheet string=w1774, array type (2D Dbl)=w1768) -> (array=w1770:string[])
            n773 = Bundle By Name(cluster=w1769, "RPM Sweep"=w1770) -> (w1771:T7)
          }
          frame "RPM Target", "Spin" {
            # "1.65V/50RPM"
            # "Set the RPM target and spin state"
            n774 = Not Equal?(x=variant, y=w1821) -> (x != y?=w1820:bool)
            n775 = Unbundle By Name(w1816) -> ("Current RPM"=w1803:dbl, "Queue Array"=w1813:T8, "Queue Element"=w1806:T9)  [unwired: 1 out]
            n776 = case shown="True" w1820 {
              tunnel: w1823 -> [w1836 w1841]
              tunnel: [w1836 w1840] -> w1800
              tunnel: w1821 -> [_ w1839]
              tunnel: [w1835 w1838] -> w1818
              tunnel: cluster{"RPM":dbl, bool} {"RPM"=0.0, FALSE} -> [w1835 w1837]
              frame False {
              }
              frame True {
                n777 = Variant To Data(error in=w1841, type=w1837, Variant=w1839) -> (data=w1838:cluster{"RPM":dbl, bool}, error out=w1840:errorcluster)
              }
            }
            n778 = Unbundle(w1818) -> ("RPM"=w1812:dbl, w1802:bool)
            n779 = local read "Auto Pulse"() -> (w1793:bool)
            n780 = Select(t=w1812, s=w1802, f=0.0) -> (s? t:f=w1788:dbl)
            n781 = local write "RPM Target"(w1812) -> ()
            n782 = Greater Than 0?(x=w1788) -> (x > 0?=w1792:bool)
            n783 = local write "Spin"(w1792) -> ()
            n784 = And(x=w1792, y=w1793) -> (x .and. y?=w1789:bool)
            n785 = call <vilib>:"DAQmx Stop Task.vi"("task/channels in"=refnum<k21> "PrecorPulsedRPM", "error in"=w1800) -> ("task out"=w1796:refnum<k21>, "error out"=w1799:errorcluster)  [unwired: 12 in]
            n786 = Index Array(array=w1813, index=1) -> (element=w1805:refnum<queue>)
            n787 = Bundle By Name(cluster=w1806, "state"="Update RPM", "data"=w1788) -> (w1808:T9)
            n788 = call <vilib>:"DAQmx Clear Task.vi"("task in"=w1796, "error in"=w1799) -> ("error out"=w1797:errorcluster)  [unwired: 13 in]
            n789 = Enqueue Element At Opposite End(queue=w1805, element=w1808, error in (no error)=w1797) -> (error out=w1807:errorcluster)  [unwired: 1 in, 2 out]
            n790 = call "RPM Ramp.vi"("Requested RPM"=w1788, "Current RPM"=w1803) -> ("RPM Ramp"=w1815:dbl[])  [unwired: 9 in]
            n791 = for {
              tunnel: w1807 -> [w1834]
              tunnel: [w1831] -> w1801
              tunnel: w1815 -> [w1833] mode=indexing
              tunnel: [w1827] -> w1795
              n792 = expression code="x*0.033"(w1833) -> (w1830:dbl)
              n793 = call-poly <vilib>:"DAQmx Write.vi"("task/channels in"=refnum<k21> "PrecorAO", "auto start"=TRUE, "data"=w1830, "error in"=w1834) -> ("task out"=w1827:refnum<k21>, "error out"=w1832:errorcluster)  [unwired: 9 in, 1 out]
              n794 = call "Time Delay"("error in (no error)"=w1832) -> ("error out"=w1831:errorcluster)  [unwired: 10 in]
            }
            n795 = control-ref of="Average RPM"() -> (w1810:refnum<vi>)
            n796 = property class="DigNum (strict)"(reference=w1810, "Val(Sgnl)"=w1788) -> ()  [unwired: 1 in, 2 out]
            n797 = Bundle By Name(cluster=w1816, "Rotating"=w1802, "Current RPM"=w1788) -> (w1817:T7)
            n798 = call <vilib>:"DAQmx Wait Until Done.vi"("task/channels in"=w1795, "timeout (sec)"=-1.0, "error in"=w1801) -> ("error out"=w1791:errorcluster)  [unwired: 11 in, 1 out]
            n799 = case shown="True" w1789 {
              selector: w1789 -> [_ w1825]
              tunnel: w1791 -> [w1824 w1826]
              tunnel: [w1824 w1826] -> w1790
              frame False {
              }
              frame True {
                n800 = property on="Start Pulse" class="Bool (strict)"("Val(Sgnl)"=w1825) -> ()  [unwired: 2 in, 2 out]
              }
            }
          }
          frame "save config" {
            # "Store the current configuration"
            n801 = call <vilib>:"Application Directory.vi"() -> ("Application Directory"=w1867:path)
            n802 = Equal?(x=variant, y=w1870) -> (x = y?=w1869:bool)
            n803 = Build Path(base path=w1867, name or relative path="data") -> (appended path=w1865:path)
            n804 = Build Path(base path=w1865, name or relative path="lastcfg.ini") -> (appended path=w1853:path)
            n805 = Unbundle By Name(w1854) -> ("Cfg Cntrls"=w1843:refnum<vi>[])
            n806 = case shown="False" w1869 {
              tunnel: w1872 -> [w1884 w1886]
              tunnel: [w1883 w1886] -> w1868
              tunnel: w1870 -> [w1882 _]
              tunnel: [w1881 w1885] -> w1852
              tunnel: w1853 -> [w1880 w1885]
              frame False {
                n807 = Variant To Data(error in=w1884, type=w1880, Variant=w1882) -> (data=w1881:path, error out=w1883:errorcluster)
              }
              frame True {
              }
            }
            n808 = call "Config to DB Data.vi"("error in (no error)"=w1868, "Control References Array"=w1843) -> ("error out"=w1863:errorcluster, "Name"=w1860:string[], "Data"=w1859:string[])  [unwired: 7 in]
            n809 = property on="Data Setup" class="MCListbox (strict)"() -> ("Label.Text"=w1850:string, "ItemNames"=w1848:string[][], "ItemSyms"=w1844:i32[])  [unwired: 2 in, 2 out]
            n810 = Build Array (concatenate)(w1850, w1860) -> (w1851:string[])
            n811 = Bundle("ItemNames"=w1848, "ItemSyms"=w1844) -> (w1845:T23)  [unwired: 1 in]
            n812 = To Variant(anything=w1845) -> (Variant=w1849:variant)
            n813 = call "Variant to db String.vi"("Control Data"=w1849) -> ("DB String"=w1846:string)  [unwired: 8 in, 2 out]
            n814 = Build Array (concatenate)(w1846, w1859) -> (w1847:string[])
            n815 = call <vilib>:"Open Config Data.vi"("error in (no error)"=w1863, "configuration file path"=w1852) -> ("error out"=w1862:errorcluster, "refnum"=w1861:T19)  [unwired: 7 in, 1 out]
            n816 = for {
              tunnel: w1862 -> [w1879]
              tunnel: w1861 -> [w1878]
              tunnel: w1851 -> [w1877] mode=indexing
              tunnel: w1847 -> [w1876] mode=indexing
              tunnel: "config" -> [w1875]
              tunnel: [w1874] -> w1857
              tunnel: [w1873] -> w1856
              n817 = call-poly <vilib>:"Write Key.vi"("section"=w1875, "error in (no error)"=w1879, "value"=w1876, "key"=w1877, "refnum"=w1878) -> ("error out"=w1874:errorcluster, "refnum out"=w1873:T19)  [unwired: 4 in, 1 out]
            }
            n818 = call <vilib>:"Close Config Data.vi"("error in (no error)"=w1857, "refnum"=w1856) -> ("error out"=w1855:errorcluster)  [unwired: 8 in, 1 out]
          }
          frame "Set parameters" {
            w1895 = "," ("delimiter (Tab)")
            w1894 = ""
            # "Read the controls again to make certain the newest values are set"
            n819 = local read "Step Height Sweep"() -> (w1891:string)
            n820 = local read "Ibrake Sweep"() -> (w1906:string)
            n821 = local read "Range Sweep"() -> (w1892:string)
            n822 = local read "Load Sweep"() -> (w1904:string)
            n823 = local read "RPM Sweep"() -> (w1903:string)
            n824 = Unbundle By Name(w1905) -> ("Ibrake Sweep"=w1893:string[])
            n825 = Spreadsheet String To Array(delimiter (Tab)=w1895, format string=w1894, spreadsheet string=w1906, array type (2D Dbl)=w1893) -> (array=w1899:string[])
            n826 = Spreadsheet String To Array(delimiter (Tab)=w1895, format string=w1894, spreadsheet string=w1903, array type (2D Dbl)=w1893) -> (array=w1901:string[])
            n827 = Spreadsheet String To Array(delimiter (Tab)=w1895, format string=w1894, spreadsheet string=w1904, array type (2D Dbl)=w1893) -> (array=w1902:string[])
            n828 = Spreadsheet String To Array(delimiter (Tab)=w1895, format string=w1894, spreadsheet string=w1891, array type (2D Dbl)=w1893) -> (array=w1889:string[])
            n829 = Spreadsheet String To Array(delimiter (Tab)=w1895, format string=w1894, spreadsheet string=w1892, array type (2D Dbl)=w1893) -> (array=w1890:string[])
            n830 = Decimal String To Number(string=w1899) -> (number=w1900:i32[])  [unwired: 2 in, 1 out]
            n831 = Number To Hexadecimal String(2:w1900) -> (0:w1898:string[])  [unwired: 1 in]
            n832 = Bundle By Name(cluster=w1905, "Ibrake Sweep"=w1898, "RPM Sweep"=w1901, "Load Sweep"=w1902, "Step Height Sweep"=w1889, "Range Sweep"=w1890) -> (w1907:T7)
            n833 = call "Set Parameters.vi"("error in (no error)"=w1888, "Cluster in"=w1907) -> ("error out"=w1896:errorcluster, "Cluster out"=w1897:T7)  [unwired: 8 in]
          }
          frame "Set UI" {
            # "Setup the user interface according to the test"
            n834 = Unbundle By Name(w1910) -> ("Queue Array"=w1911:T8, "Available Tests"=w1915:T2)
            n835 = Not Equal?(x=variant, y=w1919) -> (x != y?=w1918:bool)
            n836 = case shown="False" w1918 {
              tunnel: w1921 -> [w1923 w1928]
              tunnel: [w1923 w1927] -> w1913
              tunnel: w1919 -> [_ w1926]
              tunnel: [w1922 w1925] -> w1916
              tunnel: w1915 -> [w1922 w1924]
              frame False {
              }
              frame True {
                n837 = Variant To Data(error in=w1928, type=w1924, Variant=w1926) -> (data=w1925:T2, error out=w1927:errorcluster)
              }
            }
            n838 = Index Array(array=w1911, index=0) -> (element=w1914:refnum<queue>)
            n839 = local write "Available Tests"(w1916) -> ()
            n840 = Flush Queue(queue=w1914, error in (no error)=w1913) -> (error out=w1912:errorcluster)  [unwired: 2 out]
            n841 = call "Set UI.vi"("error in (no error)"=w1912, "Available Tests"=w1916, "Cluster"=w1910) -> ("error out"=w1917:errorcluster)  [unwired: 8 in]
          }
          frame "Console Select" {
            # "Setup the user interface according to the test"
            n842 = local read "Console Select"() -> (w1935:T1)
            n843 = Not Equal?(x=variant, y=w1939) -> (x != y?=w1938:bool)
            n844 = case shown="True" w1938 {
              tunnel: w1941 -> [w1943 w1948]
              tunnel: [w1943 w1947] -> w1934
              tunnel: w1939 -> [_ w1946]
              tunnel: [w1942 w1945] -> w1933
              tunnel: w1935 -> [w1942 w1944]
              frame False {
              }
              frame True {
                n845 = Variant To Data(error in=w1948, type=w1944, Variant=w1946) -> (data=w1945:T1, error out=w1947:errorcluster)
              }
            }
            n846 = local write "Console Select"(w1933) -> ()
            n847 = call "Console Select.vi"("error in (no error)"=w1934, "Console Select"=w1933) -> ("error out"=w1932:errorcluster, "Console Out"=w1931:string[])  [unwired: 7 in]
            n848 = call "Variables.vi"("error in (no error)"=w1932, "Value"=w1931, "Command"=T21."Init") -> ("error out"=w1929:errorcluster)  [unwired: 6 in, 2 out]
          }
          frame "lock ui" {
            # "Lock the controls"
            n849 = Not Equal?(x=variant, y=w1955) -> (x != y?=w1954:bool)
            n850 = case shown="True" w1954 {
              selector: w1954 -> [w1958 w1960]
              tunnel: w1957 -> [w1959 w1964]
              tunnel: [w1959 w1963] -> w1953
              tunnel: w1955 -> [_ w1962]
              tunnel: [w1958 w1961] -> w1951
              frame False {
              }
              frame True {
                n851 = Variant To Data(error in=w1964, type=w1960, Variant=w1962) -> (data=w1961:bool, error out=w1963:errorcluster)
              }
            }
            n852 = call "Set UI.vi"("Lock"=w1951, "error in (no error)"=w1953, "Cluster"=w1950) -> ("error out"=w1952:errorcluster)  [unwired: 8 in]
          }
          frame "Start Pulse" {
            # "This case starts the pulse for the pulse test"
            n853 = Unbundle By Name(w1971) -> ("Pulse Waveform"=w1976:waveform(dbl), "Rotating"=w1966:bool)
            n854 = Not Equal?(x=variant, y=w1982) -> (x != y?=w1981:bool)
            n855 = case shown="True" w1981 {
              tunnel: w1984 -> [w2010 w2015]
              tunnel: [w2010 w2014] -> w1978
              tunnel: w1982 -> [_ w2013]
              tunnel: [w2009 w2012] -> _
              tunnel: w1981 -> [w2009 w2011]
              frame False {
              }
              frame True {
                n856 = Variant To Data(error in=w2015, type=w2011, Variant=w2013) -> (data=w2012:bool, error out=w2014:errorcluster)
              }
            }
            n857 = Unbundle By Name(w1976) -> ("dt"=w1975:dbl)
            n858 = local read "Start Pulse"() -> (w1965:bool)
            n859 = Reciprocal(x=w1975) -> (1/x=w1974:dbl)
            n860 = Unbundle By Name(w1971) -> ("Ctrl Refs.RPM Target"=w1969:refnum<vi>, "Current RPM"=w1970:dbl, "Ctrl Refs.RPM Target"=w1967:refnum<vi>, "Ctrl Refs.Spin"=w1968:refnum<vi>)
            n861 = property class="DAQmx Timing"(reference=refnum<k21> "PrecorPulsedRPM" ("task/channels in"), "SampClk.Rate"=w1974) -> (reference out=w1977:refnum<k21>)  [unwired: 1 in, 1 out]
            n862 = And(x=w1966, y=w1965) -> (x .and. y?=w1972:bool)
            n863 = case shown="False" w1972 {
              tunnel: [w1993 w1999] -> w1980
              tunnel: w1977 -> [w1996 w2008]
              tunnel: w1976 -> [_ w2007]
              tunnel: w1978 -> [w1995 w2006]
              tunnel: w1970 -> [w1992 _]
              tunnel: w1969 -> [w1991 _]
              tunnel: w1968 -> [w1985 w2004]
              tunnel: w1967 -> [w1986 w2001]
              frame False {
                w1987 = T24."Enabled" ("Disabled")
                n864 = call <vilib>:"DAQmx Stop Task.vi"("task/channels in"=w1996, "error in"=w1995) -> ("task out"=w1998:refnum<k21>, "error out"=w1997:errorcluster)  [unwired: 12 in]
                n865 = local write "Start Pulse"(FALSE ("Start Pulse")) -> ()
                n866 = call <vilib>:"DAQmx Clear Task.vi"("task in"=w1998, "error in"=w1997) -> ("error out"=w1989:errorcluster)  [unwired: 13 in]
                n867 = property class="Bool (strict)"(reference=w1985, error in=w1989, "DisabledEnum"=w1987) -> (error out=w1990:errorcluster)  [unwired: 1 out]
                n868 = property class="DigNum (strict)"(reference=w1986, error in=w1990, "DisabledEnum"=w1987) -> (error out=w1988:errorcluster)  [unwired: 1 out]
                n869 = property class="DigNum (strict)"(reference=w1991, error in=w1988, "Val(Sgnl)"=w1992) -> (error out=w1993:errorcluster)  [unwired: 1 out]
              }
              frame True {
                w2000 = T24."Enabled" ("Disabled")
                n870 = call-poly <vilib>:"DAQmx Write.vi"("task/channels in"=w2008, "auto start"=TRUE, "data"=w2007, "error in"=w2006) -> ("error out"=w2003:errorcluster)  [unwired: 9 in, 2 out]
                n871 = property class="Bool (strict)"(reference=w2004, error in=w2003, "DisabledEnum"=w2000) -> (error out=w2002:errorcluster)  [unwired: 1 out]
                n872 = property class="DigNum (strict)"(reference=w2001, error in=w2002, "DisabledEnum"=w2000) -> (error out=w1999:errorcluster)  [unwired: 1 out]
              }
            }
          }
          frame "Start Test" {
            w2022 = 0 ("RPM Counter")
            # "This case starts the test sequence"
            n873 = call "Dwell Wait Time"("Enable"=TRUE, "error in (no error)"=w2027) -> ("Dwell Wait Time"=w2024:dbl, "OK"=w2019:bool, "error out"=w2025:errorcluster)  [unwired: 15 in]
            n874 = call "File Storage Selection"("Enable"=w2019, "error in (no error)"=w2025) -> ("Use Current"=w2016:bool, "error out"=w2032:errorcluster)  [unwired: 16 in]
            n875 = Not(x=w2019) -> (.not. x?=w2018:bool)
            n876 = Bundle By Name(cluster=w2029, "Stop Time"=w2024) -> (w2028:T7)
            n877 = Or(x=w2018, y=w2016) -> (x .or. y?=w2017:bool)
            n878 = case shown="True" w2017 {
              tunnel: w2032 -> [w2054 w2065]
              tunnel: [w2050 w2064] -> w2031
              tunnel: [w2047 w2063] -> w2030
              tunnel: w2016 -> [_ w2062]
              frame False {
                n879 = call "File Dialog3"("prompt"="Please Select a Storage File", "error in"=w2054) -> ("selected path"=w2052:path, "exists"=w2049:bool, "cancelled"=w2048:bool, "error out"=w2051:errorcluster)  [unwired: 10 in]
                n880 = case shown="True" w2049 {
                  tunnel: w2051 -> [w2056 w2060]
                  tunnel: [w2056 w2059] -> w2050
                  tunnel: w2048 -> [w2055 _]
                  tunnel: [w2055 w2057] -> w2047
                  frame False {
                  }
                  frame True {
                    n881 = call "Display Message to User2"("error in (no error)"=w2060) -> ("error out"=w2059:errorcluster, "OK"=w2058:bool)  [unwired: 9 in]
                    n882 = Not(x=w2058) -> (.not. x?=w2057:bool)
                  }
                }
                n883 = case shown="False" w2047 {
                  tunnel: w2052 -> [w2061 _]
                  frame False {
                    n884 = property on="Path" class="Path"("Val(Sgnl)"=w2061) -> ()  [unwired: 2 in, 2 out]
                  }
                  frame True {
                  }
                }
              }
              frame True {
                n885 = case shown="True" w2062 {
                  tunnel: w2065 -> [w2066 w2071]
                  tunnel: [w2066 w2070] -> w2064
                  tunnel: [TRUE w2069] -> w2063
                  frame False {
                  }
                  frame True {
                    n886 = call "Display Message to User"("error in (no error)"=w2071, "Message"="Existing Data Will Be Appended!") -> ("error out"=w2070:errorcluster, "OK"=w2072:bool)  [unwired: 8 in]
                    n887 = Not(x=w2072) -> (.not. x?=w2069:bool)
                  }
                }
              }
            }
            n888 = Unbundle By Name(w2028) -> ("Queue Array"=w2033:T8)
            n889 = case shown="False" w2030 {
              tunnel: [w2045 w2046] -> w2035
              tunnel: w2033 -> [w2044 _]
              tunnel: w2031 -> [w2042 w2046]
              frame False {
                n890 = Index Array(array=w2044) -> (element=w2040:refnum<queue>)  [unwired: 1 in]
                n891 = Bundle By Name(cluster=T9 {"state"="Lock UI", "data"=variant} ("element"), "data"=TRUE) -> (w2037:T9)
                n892 = Enqueue Element(queue=w2040, element=w2037, error in (no error)=w2042) -> (queue out=w2039:refnum<queue>, error out=w2041:errorcluster)  [unwired: 1 in, 1 out]
                n893 = Enqueue Element(queue=w2039, element=T9 {"state"="Check Temp", "data"=variant}, error in (no error)=w2041) -> (error out=w2045:errorcluster)  [unwired: 1 in, 2 out]
              }
              frame True {
              }
            }
            n894 = local read "Available Tests"() -> (w2023:T2)
            n895 = local write "Start Test"(FALSE ("Start Test")) -> ()
            n896 = Bundle By Name(cluster=w2028, "A Counter"=w2022, "B Counter"=w2022, "C Counter"=w2022, "Available Tests"=w2023, "#A"=w2022, "#B"=w2022, "#C"=w2022) -> (w2034:T7)
          }
          frame "Stop Test" {
            w2074 = FALSE ("Pause Test")
            # "Case to gracefully stop the test"
            n897 = Not Equal?(x=variant, y=w2100) -> (x != y?=w2099:bool)
            n898 = Unbundle By Name(w2098) -> ("Queue Array"=w2097:T8, "Ctrl Refs.Available Tests"=w2077:refnum<vi>)
            n899 = case shown="False" w2099 {
              tunnel: w2103 -> [w2109 w2114]
              tunnel: [w2109 w2113] -> w2102
              tunnel: w2100 -> [_ w2112]
              tunnel: [w2108 w2111] -> _
              tunnel: w2099 -> [w2108 w2110]
              frame False {
              }
              frame True {
                n900 = Variant To Data(error in=w2114, type=w2110, Variant=w2112) -> (data=w2111:bool, error out=w2113:errorcluster)
              }
            }
            n901 = Index Array(array=w2097) -> (element #1=w2096:refnum<queue>, element #2=w2079:refnum<queue>)  [unwired: 2 in]
            n902 = Flush Queue(queue=w2096, error in (no error)=w2102) -> (queue out=w2095:refnum<queue>, error out=w2094:errorcluster)  [unwired: 1 out]
            n903 = Bundle By Name(cluster=T9 {"state"="Spin", "data"=variant} ("element"), "data"=cluster{"RPM":dbl, bool} {"RPM"=0.0, FALSE}) -> (w2088:T9)
            n904 = Bundle By Name(cluster=T9 {"state"="Load Bank", "data"=variant} ("element"), "data"=Load_Bank."OFF" ("Load Bank")) -> (w2087:T9)
            n905 = Bundle By Name(cluster=T9 {"state"="Ibrake", "data"=variant} ("element"), "data"="0") -> (w2086:T9)
            n906 = Bundle By Name(cluster=T9 {"state"="Set UI", "data"=variant} ("element"), "data"=w2077) -> (w2076:T9)
            n907 = Build Array(w2088, w2086, w2087, w2076) -> (w2085:T9[])
            n908 = for {
              tunnel: w2095 -> [w2107]
              tunnel: w2094 -> [w2106]
              tunnel: [w2105] -> w2093
              tunnel: w2085 -> [w2104] mode=indexing
              n909 = Enqueue Element(queue=w2107, element=w2104, error in (no error)=w2106) -> (error out=w2105:errorcluster)  [unwired: 1 in, 2 out]
            }
            n910 = local write "SS#"(0 ("f")) -> ()
            n911 = Enqueue Element(queue=w2079, element=T9 {"state"="Stop Test", "data"=variant}, error in (no error)=w2093) -> (error out=w2080:errorcluster)  [unwired: 1 in, 2 out]
            n912 = local write "Test Status"("Stopped") -> ()
            n913 = local write "Stop Test"(w2074) -> ()
            n914 = local write "Pause Test"(w2074) -> ()
          }
          frame "test prep" {
            w2122 = T9 {"state"="", "data"=variant} ("t")
            # "This case arbitrates what to execute base on selected test"
            n915 = local read "Over Temp"() -> (w2116:bool)
            n916 = Not Equal?(x=variant, y=w2142) -> (x != y?=w2141:bool)
            n917 = local read "Pause Test"() -> (w2117:bool)
            n918 = case shown="True" w2141 {
              tunnel: w2144 -> [w2171 w2176]
              tunnel: [w2171 w2175] -> w2129
              tunnel: w2142 -> [_ w2174]
              tunnel: [w2170 w2173] -> _
              tunnel: w2141 -> [w2170 w2172]
              frame False {
              }
              frame True {
                n919 = Variant To Data(error in=w2176, type=w2172, Variant=w2174) -> (data=w2173:bool, error out=w2175:errorcluster)
              }
            }
            n920 = Unbundle By Name(w2127) -> ("Available Tests"=w2120:T2, "Queue Array"=w2126:T8)
            n921 = Or(x=w2117, y=w2116) -> (x .or. y?=w2118:bool)
            n922 = Index Array(array=w2126) -> (element=w2140:refnum<queue>)  [unwired: 1 in]
            n923 = Flush Queue(queue=w2140, error in (no error)=w2129) -> (queue out=w2139:refnum<queue>, error out=w2138:errorcluster)  [unwired: 1 out]
            n924 = Select(t=w2122, s=w2118, f=T9 {"state"="Next Test", "data"=variant} ("element")) -> (s? t:f=w2123:T9)
            n925 = Bundle By Name(cluster=T9 {"state"="Spin", "data"=variant} ("element"), "data"=cluster{"RPM":dbl, bool} {"RPM"=0.0, FALSE}) -> (w2134:T9)
            n926 = Bundle By Name(cluster=T9 {"state"="Ibrake", "data"=variant} ("element"), "data"="0") -> (w2132:T9)
            n927 = Bundle By Name(cluster=T9 {"state"="Load Bank", "data"=variant} ("element"), "data"=Load_Bank."OFF" ("Load Bank")) -> (w2133:T9)
            n928 = case shown="\"Generator Torque\"..\"Generator Thermal\", \"AMT Brake Thermal\", \"Bike Brake Thermal\"" w2120 {
              tunnel: w2134 -> [w2150 w2156]
              tunnel: w2133 -> [_ w2161]
              tunnel: w2132 -> [_ w2160]
              tunnel: [w2154 w2159] -> w2131
              tunnel: w2123 -> [w2153 w2158]
              tunnel: w2118 -> [w2151 w2157]
              tunnel: w2122 -> [w2149 w2155]
              frame "Manual", "EFX Brake Torque", "Pulsed RPM".."Bike Brake Torque" {
                n929 = Select(t=w2150, s=w2151, f=w2149) -> (s? t:f=w2152:T9)
                n930 = Build Array(w2152, w2153) -> (w2154:T9[])
              }
              frame "Generator Torque".."Generator Thermal", "AMT Brake Thermal", "Bike Brake Thermal" {
                n931 = case shown="True" w2157 {
                  tunnel: w2156 -> [w2162 w2169]
                  tunnel: w2161 -> [_ w2168]
                  tunnel: w2160 -> [_ w2167]
                  tunnel: [w2164 w2166] -> w2159
                  tunnel: w2158 -> [w2163 w2165]
                  tunnel: w2155 -> [_ _]
                  frame False {
                    n932 = Build Array(w2162, w2163) -> (w2164:T9[])
                  }
                  frame True {
                    n933 = Build Array(w2169, w2167, w2168, w2165) -> (w2166:T9[])
                  }
                }
              }
            }
            n934 = Reverse 1D Array(array=w2131) -> (reversed array=w2125:T9[])
            n935 = for {
              tunnel: w2139 -> [w2148]
              tunnel: w2138 -> [w2147]
              tunnel: [w2146] -> w2128
              tunnel: w2125 -> [w2145] mode=indexing
              n936 = Enqueue Element At Opposite End(queue=w2148, element=w2145, error in (no error)=w2147) -> (error out=w2146:errorcluster)  [unwired: 1 in, 2 out]
            }
          }
          frame Default {
            # "Case for programming"
            n937 = Not Equal?(x=variant, y=w2183) -> (x != y?=w2182:bool)
            n938 = case shown="True" w2182 {
              tunnel: w2185 -> [w2198 w2203]
              tunnel: [w2198 w2202] -> w2180
              tunnel: w2183 -> [_ w2201]
              tunnel: [w2197 w2200] -> _
              tunnel: w2182 -> [w2197 w2199]
              frame False {
              }
              frame True {
                n939 = Variant To Data(error in=w2203, type=w2199, Variant=w2201) -> (data=w2200:bool, error out=w2202:errorcluster)
              }
            }
            n940 = local read "Over Temp"() -> (w2181:bool)
            n941 = case shown="True" w2181 {
              tunnel: w2180 -> [w2186 w2188]
              tunnel: w2179 -> [_ w2196]
              tunnel: [w2186 w2187] -> w2178
              frame False {
              }
              frame True {
                # "Just added this for ver3.3"
                n942 = Unbundle By Name(w2196) -> ("Queue Array"=w2195:T8, "Queue Element"=w2190:T9)
                n943 = Bundle By Name(cluster=w2190, "state"="Over Temp", "data"=TRUE) -> (w2189:T9)
                n944 = Index Array(array=w2195, index=0) -> (element=w2191:refnum<queue>)
                n945 = Enqueue Element At Opposite End(queue=w2191, element=w2189, error in (no error)=w2188) -> (error out=w2187:errorcluster)  [unwired: 1 in, 2 out]
              }
            }
          }
          frame "update indices" {
            n946 = Unbundle By Name(w2208) -> ("T_Monitor Indices"=w2207:i32[])
            n947 = Not Equal?(x=variant, y=w2210) -> (x != y?=w2209:bool)
            n948 = case shown="False" w2209 {
              tunnel: w2213 -> [w2215 w2220]
              tunnel: [w2215 w2219] -> w2212
              tunnel: w2210 -> [_ w2218]
              tunnel: [w2214 w2217] -> w2205
              tunnel: w2207 -> [w2214 w2216]
              frame False {
              }
              frame True {
                n949 = Variant To Data(error in=w2220, type=w2216, Variant=w2218) -> (data=w2217:i32[], error out=w2219:errorcluster)
              }
            }
            n950 = Bundle By Name(cluster=w2208, "T_Monitor Indices"=w2205) -> (w2206:T7)
          }
          frame "Thermal Limit" {
            # "Update the thermal limit"
            n951 = Unbundle By Name(w2225) -> ("Thermal Limit"=w2224:i32)
            n952 = Not Equal?(x=variant, y=w2227) -> (x != y?=w2226:bool)
            n953 = case shown="False" w2226 {
              tunnel: w2230 -> [w2232 w2237]
              tunnel: [w2232 w2236] -> w2229
              tunnel: w2227 -> [_ w2235]
              tunnel: [w2231 w2234] -> w2222
              tunnel: w2224 -> [w2231 w2233]
              frame False {
              }
              frame True {
                n954 = Variant To Data(error in=w2237, type=w2233, Variant=w2235) -> (data=w2234:i32, error out=w2236:errorcluster)
              }
            }
            n955 = Bundle By Name(cluster=w2225, "Thermal Limit"=w2222) -> (w2223:T7)
          }
          frame "Thermal Resume" {
            # "Update the thermal resume"
            n956 = Unbundle By Name(w2242) -> ("Thermal Resume"=w2241:i32)
            n957 = Not Equal?(x=variant, y=w2244) -> (x != y?=w2243:bool)
            n958 = case shown="False" w2243 {
              tunnel: w2247 -> [w2249 w2254]
              tunnel: [w2249 w2253] -> w2246
              tunnel: w2244 -> [_ w2252]
              tunnel: [w2248 w2251] -> w2239
              tunnel: w2241 -> [w2248 w2250]
              frame False {
              }
              frame True {
                n959 = Variant To Data(error in=w2254, type=w2250, Variant=w2252) -> (data=w2251:i32, error out=w2253:errorcluster)
              }
            }
            n960 = Bundle By Name(cluster=w2242, "Thermal Resume"=w2239) -> (w2240:T7)
          }
          frame "Save Pulse Data" {
            # "Setup saving the data from the pulse data test"
            n961 = Not Equal?(x=variant, y=w2267) -> (x != y?=w2266:bool)
            n962 = Unbundle By Name(w2264) -> ("Queue Array"=w2263:T8, "Queue Element"=w2260:T9)
            n963 = case shown="False" w2266 {
              tunnel: w2269 -> [w2271 w2276]
              tunnel: [w2271 w2275] -> w2256
              tunnel: w2267 -> [_ w2274]
              tunnel: [w2270 w2273] -> w2257
              tunnel: w2266 -> [w2270 w2272]
              frame False {
              }
              frame True {
                n964 = Variant To Data(error in=w2276, type=w2272, Variant=w2274) -> (data=w2273:bool, error out=w2275:errorcluster)
              }
            }
            n965 = Index Array(array=w2263, index=1) -> (element=w2261:refnum<queue>)
            n966 = Bundle By Name(cluster=w2260, "state"="update pulse save", "data"=w2257) -> (w2259:T9)
            n967 = Enqueue Element At Opposite End(queue=w2261, element=w2259, error in (no error)=w2256) -> (error out=w2265:errorcluster)  [unwired: 1 in, 2 out]
          }
        }
      }
      frame Error {
        n968 = Unbundle By Name(w2280) -> ("Queue List"=w2278:string[], "Queue Array"=w2279:T8, "Last State"=w2283:string)
        n969 = call "Reentrant Send Error.vi"("Queue Names"=w2278, "error in (no error)"=w2282, "Last State"=w2283, "Queues"=w2279) -> ("error out"=w2281:errorcluster)  [unwired: 7 in]
      }
    }
  }
  n970 = while {
    shift-right: [w2286] -> _
    shift-left: w2 -> [w2291]
    tunnel: w55 -> [w2288]
    shift-right: [w2289] -> w52
    shift-left: w5 -> [w2290]
    tunnel: w18 -> [w2285]
    i -> [w2284]
    stop <- w2287 stop-if-true
    # "Data Acquisition"
    n971 = case shown="No Error" w2290 {
      selector: w2290 -> [w2305 w2925]
      tunnel: w2291 -> [w2298 w2923]
      tunnel: [w2303 w2924] -> w2289
      tunnel: w2288 -> [w2302 w2926]
      tunnel: [w2301 w2926] -> w2287
      tunnel: [w2299 w2923] -> w2286
      tunnel: w2285 -> [w2297 _]
      tunnel: w2284 -> [_ _]
      frame No Error {
        w2292 = 1 ("index")
        n972 = Unbundle By Name(w2298) -> ("Queue Array"=w2307:T8)
        n973 = Get Date/Time In Seconds() -> (seconds since 1Jan1904=w2296:timestamp)
        "Time Stamp Control" <- w2296
        n974 = call "Dequeue Element.vi"("timeout in ms (-1)"=25, "error in (no error)"=w2305, "index"=w2292, "Queue Array"=w2307) -> ("error out"=w2304:errorcluster, "Queue Element"=w2293:T9)  [unwired: 5 in, 1 out]
        n975 = Unbundle By Name(w2293) -> ("state"=w2294:string, "data"=w2300:variant)
        n976 = Bundle By Name(cluster=w2298, "Last State"=w2294) -> (w2295:T7)
        n977 = case shown="Default" w2294 {
          selector: w2294 -> [_ _ _ _ w2431 _ _ _ _ _ _ _ _ _ _ _ _ _ _ _ _ _ _ _ _ _ _]
          tunnel: w2304 -> [w2319 w2362 w2380 w2421 w2438 w2447 w2460 w2494 w2524 w2542 w2554 w2571 w2587 w2604 w2621 w2636 w2669 w2694 w2716 w2736 w2756 w2776 w2797 w2814 w2831 w2849 w2878]
          tunnel: [w2330 w2355 w2397 w2416 w2433 w2447 w2456 w2492 w2523 w2542 w2549 w2566 w2582 w2599 w2616 w2633 w2665 w2685 w2712 w2731 w2751 w2771 w2792 w2810 w2827 w2845 w2859] -> w2303
          tunnel: w2302 -> [_ _ w2383 w2422 w2439 w2448 w2461 w2496 w2533 w2545 w2555 w2572 w2588 w2605 w2622 w2637 w2670 _ w2717 w2737 w2757 w2777 w2798 w2815 w2832 w2850 _]
          tunnel: [FALSE TRUE w2383 w2422 w2439 w2448 w2461 w2496 w2533 w2545 w2555 w2572 w2588 w2605 w2622 w2637 w2670 FALSE w2717 w2737 w2757 w2777 w2798 w2815 w2832 w2850 FALSE] -> w2301
          tunnel: w2300 -> [_ w2360 _ w2419 w2436 _ w2458 w2491 _ _ w2552 w2569 w2585 w2602 w2619 w2634 w2667 w2692 w2714 w2734 w2754 w2774 w2795 w2812 w2829 w2847 w2869]
          tunnel: [w2312 w2358 w2413 w2417 w2432 w2449 w2453 w2495 w2532 w2543 w2547 w2564 w2581 w2597 w2614 w2631 w2664 w2688 w2711 w2728 w2748 w2768 w2785 w2809 w2826 w2842 w2879] -> w2299
          tunnel: w2295 -> [w2318 w2358 w2414 w2417 w2434 w2450 w2455 w2489 w2531 w2544 w2550 w2567 w2583 w2600 w2617 w2632 w2663 w2682 w2713 w2732 w2752 w2772 w2788 w2808 w2825 w2844 w2865]
          tunnel: w2297 -> [_ _ _ _ _ _ _ _ _ _ _ _ _ _ _ _ _ _ _ _ _ _ _ _ _ _ _]
          tunnel: w2296 -> [w2322 _ _ _ _ _ _ _ _ _ _ _ _ _ _ _ _ _ _ _ _ _ _ _ _ _ _]
          tunnel: w2292 -> [_ w2354 _ _ _ _ _ _ _ _ _ _ _ _ _ _ _ _ _ _ _ _ _ _ _ _ _]
          frame Default {
            # "Execute this state to acquire data and update the UI \nas necessary."
            n978 = local read "Snapshot"() -> (w2320:bool)
            n979 = Bundle("seconds since 1Jan1904"=w2322, "SS#"="SS#", "Snapshot"=w2320) -> (w2314:T26)  [unwired: 1 in]
            n980 = local read "Start Pulse"() -> (w2325:bool)
            n981 = call "PrecorDAQ Default.vi"("error in (no error)"=w2319, "Default In"=w2314, "Cluster In"=w2318) -> ("error out"=w2315:errorcluster, "Cluster Out"=w2317:T7)  [unwired: 7 in]
            n982 = Unbundle By Name(w2317) -> ("Snapshot.Snapshot Number"=w2316:u16)
            n983 = local read "Spin"() -> (w2326:bool)
            n984 = Or(x=w2326, y=w2325) -> (x .or. y?=w2313:bool)
            n985 = local read "Available Tests"() -> (w2337:T2)
            n986 = local write "SS#"(w2316) -> ()
            n987 = call "Acquire.vi"("Cluster in"=w2317, "Filters"="Filters", "Available Tests"=w2337, "Active"=w2313, "error in (no error)"=w2315, "Snapshot in"=w2320) -> ("output cluster"=w2312:T7, "Over Temp"=→"Over Temp":bool, "Heartbeat"=w2324:bool, "Parsed Data"=w2334:T27, "RPM Wfm"=w2327:cluster{"X":dbl, "Y":dbl}[], "Waveform 5 seconds"=w2310:waveform(dbl)[], "error out"=w2335:errorcluster)  [unwired: 2 in, 1 out]
            "Sample" <- w2324
            n988 = local read "Graphic Display"() -> (w2328:T4)
            n989 = Index Array(array=w2310, index="Data Display") -> (element=w2308:waveform(dbl))
            n990 = Unbundle(w2334) -> ("Sample Acquired"=w2331:bool, "Torque"=w2329:dbl, "Temperatre Plot Data"=w2333:cluster{dbl[], i32[]}[], "Temperature Avg"=w2332:dbl[])  [unwired: 1 out]
            "Capture" <- w2331
            n991 = case shown="\"Analize\", Default" w2328 {
              tunnel: w2327 -> [_ w2341]
              tunnel: w2308 -> [_ w2340]
              frame "Analize", Default {
              }
              frame "Pulse" {
                "RPM Graph" <- w2341
                "Reading Graph" <- w2340
              }
            }
            n992 = case shown="True" w2324 {
              tunnel: w2333 -> [_ _]
              tunnel: w2332 -> [_ w2339]
              tunnel: w2329 -> [_ w2338]
              frame False {
              }
              frame True {
                "CH Value" <- w2339
                "Torque (in-lb)" <- w2338
              }
            }
            n993 = case shown="True" w2331 {
              tunnel: w2335 -> [w2342 w2343]
              tunnel: [w2342 w2343] -> w2330
              frame False {
              }
              frame True {
                n994 = local write "Snapshot"(FALSE ("Snapshot")) -> ()
              }
            }
          }
          frame "Exit" {
            # "Exit the program. et the MC Enable off on the way out"
            n995 = Not Equal?(x=variant, y=w2360) -> (x != y?=w2359:bool)
            n996 = case shown="False" w2359 {
              tunnel: w2362 -> [w2364 w2369]
              tunnel: [w2364 w2368] -> w2357
              tunnel: w2360 -> [_ w2367]
              tunnel: [w2363 w2366] -> _
              tunnel: w2359 -> [w2363 w2365]
              frame False {
              }
              frame True {
                n997 = Variant To Data(error in=w2369, type=w2365, Variant=w2367) -> (data=w2366:bool, error out=w2368:errorcluster)
              }
            }
            n998 = Unbundle By Name(w2358) -> ("Queue Array"=w2353:T8)
            n999 = Index Array(array=w2353, index=w2354) -> (element=w2352:refnum<queue>)
            n1000 = Release Queue(queue=w2352, error in (no error)=w2357) -> (error out=w2349:errorcluster)  [unwired: 1 in, 2 out]
            n1001 = call-poly <vilib>:"DAQmx Write.vi"("task/channels in"=refnum<k21> "PrecorFanCtrl", "data"=FALSE, "error in"=w2349) -> ("error out"=w2348:errorcluster)  [unwired: 10 in, 2 out]
            n1002 = call-poly <vilib>:"DAQmx Write.vi"("task/channels in"=refnum<k21> "PrecorMCEnable", "data"=FALSE, "error in"=w2348) -> ("error out"=w2355:errorcluster)  [unwired: 10 in, 2 out]
            n1003 = Wait (ms)(milliseconds to wait=u32 50) -> ()  [unwired: 1 out]
          }
          frame "Init" {
            w2370 = bool[] [FALSE, TRUE, TRUE] ("Fan Mode LED Array")
            w2376 = 60.0 ("y")
            w2381 = "2" ("Snapshot.Load Bank Setpoint")
            w2382 = TRUE ("Timer Reset")
            w2401 = "CH.Name" ("element")
            w2404 = 5 ("dimension size")
            # "Initialize needed settings\nfor the program"
            n1004 = Initialize Array(w2401, 12 ("dimension size")) -> (w2399:string[])
            n1005 = Unbundle By Name(w2414) -> ("Channels"=w2405:string[])
            n1006 = local write "CH Name"(w2399) -> ()
            n1007 = Array Size(array=w2405) -> (size(s)=w2390:i32)
            n1008 = Initialize Array("OFF" ("element"), w2390) -> (w2388:string[])
            n1009 = Initialize Array(w2401, w2390) -> (w2403:string[])
            n1010 = Initialize Array("0" ("element"), w2390) -> (w2392:string[])
            n1011 = Initialize Array("", w2390, w2404) -> (w2411:string[][])
            n1012 = Replace Array Subset(array=w2411, new element #1=w2405, index (col) #1=0 ("disabled index (col)"), new element #2=w2403, index (col) #2=1 ("index (col)"), new element #3=w2388, index (col) #3=2 ("index (col)"), new element #4=w2392, index (col) #4=3 ("index (col)")) -> (w2410:string[][])  [unwired: 4 in]
            n1013 = property on="Data Setup" class="MCListbox (strict)"("ItemNames"=w2410, "NumCols"=w2404, "NumRows"=u32 27 ("Number of Rows")) -> ()  [unwired: 2 in, 2 out]
            n1014 = call-poly <vilib>:"DAQmx Write.vi"("task/channels in"=refnum<k21> "PrecorFanCtrl", "data"=FALSE, "error in"=w2380) -> ("error out"=w2379:errorcluster)  [unwired: 10 in, 2 out]
            n1015 = local write "Fan Mode LED Array"(w2370) -> ()
            n1016 = local read "Stop Time"() -> (w2374:dbl)
            n1017 = local read "S Period"() -> (w2375:dbl)
            n1018 = for {
              N: 27 -> [_]
              tunnel: [w2415] -> w2393 mode=indexing
              i -> [w2415]
            }
            n1019 = Multiply(x=w2374, y=w2376) -> (x*y=w2372:dbl)
            n1020 = Multiply(x=w2376, y=w2375) -> (x*y=w2373:dbl)
            n1021 = call-poly <vilib>:"DAQmx Write.vi"("task/channels in"=refnum<k21> "PrecorMCEnable", "data"=TRUE, "error in"=w2379) -> ("error out"=w2397:errorcluster)  [unwired: 10 in, 2 out]
            n1022 = Format Into String(Load_Bank."OFF" ("Load Bank")) -> (resulting string=w2385:string)  [unwired: 3 in, 1 out]
            n1023 = Bundle By Name(cluster=w2414, "Equilibrium Stop"=FALSE, "Sample Frequency"=60.0, "Active Indicies"=w2393, "Stop Time"=w2372, "Sample Period"=w2373, "Snapshot.Ibrake Setpoint"="1" ("Snapshot.Resistance Setpoint"), "Snapshot.RPM Setpoint"="0", "Snapshot.Load Bank Setpoint"=w2385, "Snapshot.Range Setpoint"=w2381, "Snapshot.Step Height Setpoint"=w2381, "Fan Mode LED Array"=w2370, "Timer Reset"=w2382, "Autotest"=w2383, "Reset Timeout"=w2382) -> (w2413:T7)
          }
          frame "null" {
            # "Empty case for programming"
            n1024 = Not Equal?(x=variant, y=w2419) -> (x != y?=w2418:bool)
            n1025 = case shown="False" w2418 {
              tunnel: w2421 -> [w2424 w2429]
              tunnel: [w2424 w2428] -> w2416
              tunnel: w2419 -> [_ w2427]
              tunnel: [w2423 w2426] -> _
              tunnel: w2418 -> [w2423 w2425]
              frame False {
              }
              frame True {
                n1026 = Variant To Data(error in=w2429, type=w2425, Variant=w2427) -> (data=w2426:bool, error out=w2428:errorcluster)
              }
            }
          }
          frame "Test Details" {
            # "Update the test details"
            n1027 = Not Equal?(x=variant, y=w2436) -> (x != y?=w2435:bool)
            n1028 = case shown="True" w2435 {
              tunnel: w2438 -> [w2441 w2446]
              tunnel: [w2441 w2445] -> w2433
              tunnel: w2436 -> [_ w2444]
              tunnel: [w2440 w2443] -> w2430
              tunnel: w2431 -> [w2440 w2442]
              frame False {
              }
              frame True {
                n1029 = Variant To Data(error in=w2446, type=w2442, Variant=w2444) -> (data=w2443:string, error out=w2445:errorcluster)
              }
            }
            n1030 = Bundle By Name(cluster=w2434, "Snapshot.Test Details"=w2430) -> (w2432:T7)
          }
          frame "Stop Test" {
            # "Turn off autotest on Stop Test being received"
            n1031 = Bundle By Name(cluster=w2450, "Autotest"=w2448) -> (w2449:T7)
          }
          frame "update indices" {
            # "Update the indicies based on the selections"
            n1032 = Unbundle By Name(w2455) -> ("T_Monitor Indices"=w2454:i32[])
            n1033 = Not Equal?(x=variant, y=w2458) -> (x != y?=w2457:bool)
            n1034 = case shown="False" w2457 {
              tunnel: w2460 -> [w2466 w2471]
              tunnel: [w2466 w2470] -> w2456
              tunnel: w2458 -> [_ w2469]
              tunnel: [w2465 w2468] -> w2452
              tunnel: w2454 -> [w2465 w2467]
              frame False {
              }
              frame True {
                n1035 = Variant To Data(error in=w2471, type=w2467, Variant=w2469) -> (data=w2468:i32[], error out=w2470:errorcluster)
              }
            }
            n1036 = for {
              tunnel: [w2464] -> w2451 mode=indexing if=w2462
              tunnel: w2452 -> [w2463] mode=indexing
              i -> [w2464]
              n1037 = Not Equal To 0?(x=w2463) -> (x != 0?=w2462:bool)
            }
            n1038 = Bundle By Name(cluster=w2455, "T_Monitor Indices"=w2451) -> (w2453:T7)
          }
          frame "Start Test" {
            w2482 = TRUE
            # "Initiate a test"
            n1039 = Unbundle By Name(w2489) -> ("A Counter"=w2488:i32, "B Counter"=w2487:i32, "C Counter"=w2475:i32)
            n1040 = Not Equal?(x=variant, y=w2491) -> (x != y?=w2490:bool)
            n1041 = Bundle("A Counter"=w2488, "B Counter"=w2487, "C Counter"=w2475) -> (w2486:T22)  [unwired: 1 in]
            n1042 = case shown="True" w2490 {
              tunnel: w2494 -> [w2515 w2520]
              tunnel: [w2515 w2519] -> w2492
              tunnel: w2491 -> [_ w2518]
              tunnel: w2486 -> [_ w2517]
              tunnel: [T25 {"A Counter"=0, "B Counter"=0, "B Counter 2"=0} w2516] -> w2485
              frame False {
              }
              frame True {
                n1043 = Variant To Data(error in=w2520, type=w2517, Variant=w2518) -> (data=w2516:T22, error out=w2519:errorcluster)
              }
            }
            n1044 = local read "Available Tests"() -> (w2477:T2)
            n1045 = case shown="\"EFX Brake Torque\", \"EFX Brake Thermal\"" w2477 {
              tunnel: [w2497 w2500 w2504 w2505 w2509 w2513] -> w2481
              tunnel: [w2497 w2499 w2503 w2505 w2508 w2512] -> w2480
              tunnel: [w2497 w2498 w2502 w2505 w2506 w2510] -> w2479
              tunnel: [w2497 w2498 w2501 w2505 w2506 w2511] -> w2473
              tunnel: [w2497 w2498 w2501 w2505 w2507 w2510] -> w2472
              frame "Manual" {
                w2497 = "Manual Test" ("Resistance Sweep")
              }
              frame "EFX Brake Torque", "EFX Brake Thermal" {
                w2498 = ""
                n1046 = local read "Ibrake Sweep"() -> (w2500:string)
                n1047 = local read "RPM Sweep"() -> (w2499:string)
              }
              frame "Generator Torque", "Generator Thermal" {
                w2501 = ""
                n1048 = local read "Ibrake Sweep"() -> (w2504:string)
                n1049 = local read "Load Sweep"() -> (w2502:string)
                n1050 = local read "RPM Sweep"() -> (w2503:string)
              }
              frame "Pulsed RPM" {
                w2505 = ""
              }
              frame "AMT Brake Torque", "AMT Brake Thermal" {
                w2506 = ""
                n1051 = local read "Step Height Sweep"() -> (w2507:string)
                n1052 = local read "Ibrake Sweep"() -> (w2509:string)
                n1053 = local read "RPM Sweep"() -> (w2508:string)
              }
              frame "Bike Brake Torque", "Bike Brake Thermal" {
                w2510 = ""
                n1054 = local read "Ibrake Sweep"() -> (w2513:string)
                n1055 = local read "Range Sweep"() -> (w2511:string)
                n1056 = local read "RPM Sweep"() -> (w2512:string)
              }
            }
            n1057 = Format Into String(w2477) -> (resulting string=w2478:string)  [unwired: 3 in, 1 out]
            n1058 = local read "Test Details"() -> (w2476:string)
            n1059 = Unbundle By Name(w2485) -> ("A Counter"=w2484:i32, "B Counter"=w2483:i32, "C Counter"=w2474:i32)
            n1060 = Bundle By Name(cluster=w2489, "Timer Reset"=w2482, "Autotest"=w2482, "A Counter"=w2484, "B Counter"=w2483, "C Counter"=w2474, "Get Sample"=w2482, "Reset Timeout"=w2482, "Snapshot.Ibrake List"=w2481, "Snapshot.RPM List"=w2480, "Snapshot.Load Bank List"=w2479, "Snapshot.Range List"=w2473, "Snapshot.Step Height List"=w2472, "Snapshot.Test Details"=w2476, "Snapshot.Selected Test"=w2478) -> (w2495:T7)
          }
          frame "load data" {
            # "Setup the data based onthe selection"
            n1061 = local read "Available Tests"() -> (w2526:T2)
            n1062 = case shown="\"EFX Brake Torque\", Default" w2526 {
              tunnel: [w2534 w2539] -> w2530
              tunnel: [w2534 w2538] -> w2529
              tunnel: [w2534 w2537] -> w2528
              tunnel: [w2534 w2536] -> w2522
              tunnel: [w2534 w2535] -> w2521
              frame "Manual" {
                w2534 = "Manual Test" ("Resistance Sweep")
              }
              frame "EFX Brake Torque", Default {
                n1063 = local read "Step Height Sweep"() -> (w2535:string)
                n1064 = local read "Ibrake Sweep"() -> (w2539:string)
                n1065 = local read "Range Sweep"() -> (w2536:string)
                n1066 = local read "Load Sweep"() -> (w2537:string)
                n1067 = local read "RPM Sweep"() -> (w2538:string)
              }
            }
            n1068 = local read "Test Details"() -> (w2525:string)
            n1069 = Format Into String(error in=w2524, w2526) -> (resulting string=w2527:string, error out=w2523:errorcluster)  [unwired: 2 in]
            n1070 = Bundle By Name(cluster=w2531, "Snapshot.Step Height List"=w2521, "Snapshot.Range List"=w2522, "Snapshot.Ibrake List"=w2530, "Snapshot.RPM List"=w2529, "Snapshot.Load Bank List"=w2528, "Snapshot.Test Details"=w2525, "Snapshot.Selected Test"=w2527) -> (w2532:T7)
          }
          frame "End Test" {
            w2541 = FALSE
            # "Reset the Timer and Autotest at the end of the test"
            n1071 = Bundle By Name(cluster=w2544, "Timer Reset"=w2541, "Autotest"=w2541, "Snapshot"=T10 {"Test Details"="", "Version"="test", "Date"=timestamp(0 s since 1904-01-01), "Selected Test"="", "Snapshot Number"=0, "Time"=timestamp(0 s since 1904-01-01), "Ibrake Setpoint"="", "RPM Setpoint"="", "Range Setpoint"="", "Step Height Setpoint"="", "Load Bank Setpoint"="", "Measurement Headers"="", "Measurements"="", "A"=0, "B"=0, "C"=0, "Raw Data"=[], "Available Tests"=enum."Manual", "Ibrake List"="", "RPM List"="", "Load Bank List"="", "Range List"="", "Step Height List"="", "FanMode Setpoint"=enum."Auto"}) -> (w2543:T7)
          }
          frame "Thermal Limit" {
            # "Update the thermal limit"
            n1072 = Not Equal?(x=variant, y=w2552) -> (x != y?=w2551:bool)
            n1073 = case shown="False" w2551 {
              tunnel: w2554 -> [w2557 w2562]
              tunnel: [w2557 w2561] -> w2549
              tunnel: w2552 -> [_ w2560]
              tunnel: [w2556 w2559] -> w2546
              tunnel: 200 -> [w2556 w2558]
              frame False {
              }
              frame True {
                n1074 = Variant To Data(error in=w2562, type=w2558, Variant=w2560) -> (data=w2559:i32, error out=w2561:errorcluster)
              }
            }
            n1075 = Bundle By Name(cluster=w2550, "Thermal Limit"=w2546) -> (w2547:T7)
          }
          frame "Stop Time" {
            # "Update the Stop Time"
            n1076 = Not Equal?(x=variant, y=w2569) -> (x != y?=w2568:bool)
            n1077 = case shown="False" w2568 {
              tunnel: w2571 -> [w2574 w2579]
              tunnel: [w2574 w2578] -> w2566
              tunnel: w2569 -> [_ w2577]
              tunnel: [w2573 w2576] -> w2563
              tunnel: 1.0 -> [w2573 w2575]
              frame False {
              }
              frame True {
                n1078 = Variant To Data(error in=w2579, type=w2575, Variant=w2577) -> (data=w2576:dbl, error out=w2578:errorcluster)
              }
            }
            n1079 = Bundle By Name(cluster=w2567, "Stop Time"=w2563) -> (w2564:T7)
          }
          frame "autotest" {
            # "Set the autotest state"
            n1080 = Not Equal?(x=variant, y=w2585) -> (x != y?=w2584:bool)
            n1081 = case shown="True" w2584 {
              selector: w2584 -> [w2589 w2591]
              tunnel: w2587 -> [w2590 w2595]
              tunnel: [w2590 w2594] -> w2582
              tunnel: w2585 -> [_ w2593]
              tunnel: [w2589 w2592] -> w2580
              frame False {
              }
              frame True {
                n1082 = Variant To Data(error in=w2595, type=w2591, Variant=w2593) -> (data=w2592:bool, error out=w2594:errorcluster)
              }
            }
            n1083 = Bundle By Name(cluster=w2583, "Autotest"=w2580) -> (w2581:T7)
          }
          frame "S Period" {
            # "Set the sample period"
            n1084 = Not Equal?(x=variant, y=w2602) -> (x != y?=w2601:bool)
            n1085 = case shown="True" w2601 {
              tunnel: w2604 -> [w2607 w2612]
              tunnel: [w2607 w2611] -> w2599
              tunnel: w2602 -> [_ w2610]
              tunnel: [w2606 w2609] -> w2596
              tunnel: 1.0 -> [w2606 w2608]
              frame False {
              }
              frame True {
                n1086 = Variant To Data(error in=w2612, type=w2608, Variant=w2610) -> (data=w2609:dbl, error out=w2611:errorcluster)
              }
            }
            n1087 = Bundle By Name(cluster=w2600, "Sample Period"=w2596) -> (w2597:T7)
          }
          frame "Thermal Resume" {
            # "Set the thermal resume"
            n1088 = Not Equal?(x=variant, y=w2619) -> (x != y?=w2618:bool)
            n1089 = case shown="False" w2618 {
              tunnel: w2621 -> [w2624 w2629]
              tunnel: [w2624 w2628] -> w2616
              tunnel: w2619 -> [_ w2627]
              tunnel: [w2623 w2626] -> w2613
              tunnel: 200 -> [w2623 w2625]
              frame False {
              }
              frame True {
                n1090 = Variant To Data(error in=w2629, type=w2625, Variant=w2627) -> (data=w2626:i32, error out=w2628:errorcluster)
              }
            }
            n1091 = Bundle By Name(cluster=w2617, "Thermal Resume"=w2613) -> (w2614:T7)
          }
          frame "update table" {
            # "Update the names and symbols\nin the table"
            n1092 = Not Equal?(x=variant, y=w2634) -> (x != y?=w2630:bool)
            n1093 = case shown="True" w2630 {
              tunnel: w2636 -> [w2638 w2656]
              tunnel: w2634 -> [_ w2655]
              tunnel: [w2638 w2653] -> w2633
              tunnel: w2632 -> [w2639 w2652]
              tunnel: [w2639 w2643] -> w2631
              frame False {
              }
              frame True {
                n1094 = Variant To Data(error in=w2656, type=T23 {"ItemNames"=[], "ItemSyms"=[]} ("output cluster"), Variant=w2655) -> (data=w2646:T23, error out=w2644:errorcluster)
                n1095 = Unbundle By Name(w2652) -> ("Queue Array"=w2650:T8, "Ctrl Refs.Data Setup"=w2640:refnum<vi>)
                n1096 = Unbundle(w2646) -> ("ItemNames"=w2645:string[][], "ItemSyms"=w2642:i32[])
                n1097 = property class="MCListbox (strict)"(reference=w2640, error in=w2644, "ItemNames"=w2645, "ItemSyms"=w2642) -> (error out=w2654:errorcluster)  [unwired: 1 out]
                n1098 = for {
                  tunnel: [w2659] -> w2641 mode=indexing if=w2657
                  tunnel: w2642 -> [w2658] mode=indexing
                  i -> [w2659]
                  n1099 = Not Equal To 0?(x=w2658) -> (x != 0?=w2657:bool)
                }
                n1100 = Index Array(array=w2650, index=1) -> (element=w2651:refnum<queue>)
                n1101 = Enqueue Element At Opposite End(queue=w2651, element=T9 {"state"="set active channels", "data"=variant}, error in (no error)=w2654) -> (error out=w2653:errorcluster)  [unwired: 1 in, 2 out]
                n1102 = Bundle By Name(cluster=w2652, "T_Monitor Indices"=w2641) -> (w2643:T7)
              }
            }
          }
          frame "update load" {
            # "Set the load value"
            n1103 = Unbundle By Name(w2663) -> ("Load Bank"=w2662:T3)
            n1104 = Not Equal?(x=variant, y=w2667) -> (x != y?=w2666:bool)
            n1105 = case shown="True" w2666 {
              tunnel: w2669 -> [w2672 w2677]
              tunnel: [w2672 w2676] -> w2665
              tunnel: w2667 -> [_ w2675]
              tunnel: [w2671 w2674] -> w2661
              tunnel: w2662 -> [w2671 w2673]
              frame False {
              }
              frame True {
                n1106 = Variant To Data(error in=w2677, type=w2673, Variant=w2675) -> (data=w2674:T3, error out=w2676:errorcluster)
              }
            }
            n1107 = Format Into String(w2661) -> (resulting string=w2660:string)  [unwired: 3 in, 1 out]
            n1108 = Bundle By Name(cluster=w2663, "Load Bank"=w2661, "Snapshot.Load Bank Setpoint"=w2660) -> (w2664:T7)
          }
          frame "update rpm" {
            # "Set the RPM value"
            n1109 = Not Equal?(x=variant, y=w2692) -> (x != y?=w2691:bool)
            n1110 = Unbundle By Name(w2682) -> ("Get Sample"=w2680:bool, "Ctrl Refs.RPM Graph"=w2687:refnum<vi>)
            n1111 = case shown="True" w2691 {
              tunnel: w2694 -> [w2703 w2708]
              tunnel: [w2703 w2707] -> w2686
              tunnel: w2692 -> [_ w2706]
              tunnel: [w2702 w2705] -> w2681
              tunnel: 0.0 -> [w2702 w2704]
              frame False {
              }
              frame True {
                n1112 = Variant To Data(error in=w2708, type=w2704, Variant=w2706) -> (data=w2705:dbl, error out=w2707:errorcluster)
              }
            }
            n1113 = Greater Than 0?(x=w2681) -> (x > 0?=w2679:bool)
            n1114 = And(x=w2680, y=w2679) -> (x .and. y?=w2678:bool)
            n1115 = Number To Decimal String(number=w2681) -> (decimal integer string=w2689:string)  [unwired: 1 in]
            n1116 = Bundle By Name(cluster=w2682, "Get Sample"=w2678, "Current RPM"=w2681, "Snapshot.RPM Setpoint"=w2689) -> (w2688:T7)
            n1117 = Greater Than 0?(x=w2681) -> (x > 0?=w2684:bool)
            n1118 = case shown="True" w2684 {
              tunnel: w2681 -> [_ w2701]
              tunnel: w2687 -> [_ w2699]
              tunnel: w2686 -> [w2695 w2698]
              tunnel: [w2695 w2697] -> w2685
              frame False {
              }
              frame True {
                n1119 = Multiply(x=w2701, y=2.0) -> (x*y=w2696:dbl)
                n1120 = property class="XYGraph (strict)"(reference=w2699, error in=w2698, "YScale.Maximum"=w2696) -> (error out=w2697:errorcluster)  [unwired: 1 out]
              }
            }
          }
          frame "update pulse save" {
            # "Set the capture value for the pulsed RPM test"
            n1121 = Not Equal?(x=variant, y=w2714) -> (x != y?=w2709:bool)
            n1122 = case shown="True" w2709 {
              selector: w2709 -> [w2718 _]
              tunnel: w2716 -> [w2719 w2724]
              tunnel: [w2719 w2723] -> w2712
              tunnel: w2714 -> [_ w2722]
              tunnel: [w2718 w2721] -> w2710
              tunnel: w2709 -> [_ w2720]
              frame False {
              }
              frame True {
                n1123 = Variant To Data(error in=w2724, type=w2720, Variant=w2722) -> (data=w2721:bool, error out=w2723:errorcluster)
              }
            }
            n1124 = Bundle By Name(cluster=w2713, "Pulsed RPM Capture"=w2710) -> (w2711:T7)
          }
          frame "update Ibrake" {
            # "Set the Ibrake value"
            n1125 = Not Equal?(x=variant, y=w2734) -> (x != y?=w2733:bool)
            n1126 = case shown="True" w2733 {
              tunnel: w2736 -> [w2739 w2744]
              tunnel: [w2739 w2743] -> w2731
              tunnel: w2734 -> [_ w2742]
              tunnel: [w2738 w2741] -> w2729
              tunnel: "1" -> [w2738 w2740]
              frame False {
              }
              frame True {
                n1127 = Variant To Data(error in=w2744, type=w2740, Variant=w2742) -> (data=w2741:string, error out=w2743:errorcluster)
              }
            }
            n1128 = Hexadecimal String To Number(string=w2729, default (0uL)=u32 1 ("default (0 I32)")) -> (number=w2726:u32)  [unwired: 1 in, 1 out]
            n1129 = Number To Decimal String(number=w2726) -> (decimal integer string=w2725:string)  [unwired: 1 in]
            n1130 = Bundle By Name(cluster=w2732, "Current Ibrake"=w2726, "Snapshot.Ibrake Setpoint"=w2725) -> (w2728:T7)
          }
          frame "update range" {
            # "Set the Range value"
            n1131 = Not Equal?(x=variant, y=w2754) -> (x != y?=w2753:bool)
            n1132 = case shown="True" w2753 {
              tunnel: w2756 -> [w2759 w2764]
              tunnel: [w2759 w2763] -> w2751
              tunnel: w2754 -> [_ w2762]
              tunnel: [w2758 w2761] -> w2749
              tunnel: "2" -> [w2758 w2760]
              frame False {
              }
              frame True {
                n1133 = Variant To Data(error in=w2764, type=w2760, Variant=w2762) -> (data=w2761:string, error out=w2763:errorcluster)
              }
            }
            n1134 = Hexadecimal String To Number(string=w2749, default (0uL)=u32 1 ("default (0 I32)")) -> (number=w2746:u32)  [unwired: 1 in, 1 out]
            n1135 = Number To Decimal String(number=w2746) -> (decimal integer string=w2745:string)  [unwired: 1 in]
            n1136 = Bundle By Name(cluster=w2752, "Current Range"=w2746, "Snapshot.Range Setpoint"=w2745) -> (w2748:T7)
          }
          frame "update Step Height" {
            # "Set the Step Height value"
            n1137 = Not Equal?(x=variant, y=w2774) -> (x != y?=w2773:bool)
            n1138 = case shown="True" w2773 {
              tunnel: w2776 -> [w2779 w2784]
              tunnel: [w2779 w2783] -> w2771
              tunnel: w2774 -> [_ w2782]
              tunnel: [w2778 w2781] -> w2769
              tunnel: "2" -> [w2778 w2780]
              frame False {
              }
              frame True {
                n1139 = Variant To Data(error in=w2784, type=w2780, Variant=w2782) -> (data=w2781:string, error out=w2783:errorcluster)
              }
            }
            n1140 = Hexadecimal String To Number(string=w2769, default (0uL)=u32 1 ("default (0 I32)")) -> (number=w2766:u32)  [unwired: 1 in, 1 out]
            n1141 = Number To Decimal String(number=w2766) -> (decimal integer string=w2765:string)  [unwired: 1 in]
            n1142 = Bundle By Name(cluster=w2772, "Current Step Height"=w2766, "Snapshot.Step Height Setpoint"=w2765) -> (w2768:T7)
          }
          frame "update FanMode" {
            (unwired) refnum<vi> refnum ("x")
            # "Set the FanMode"
            n1143 = Unbundle By Name(w2788) -> ("FanMode"=w2789:T11)
            n1144 = Not Equal?(x=variant, y=w2795) -> (x != y?=w2794:bool)
            n1145 = case shown="False" w2794 {
              tunnel: w2797 -> [w2800 w2805]
              tunnel: [w2800 w2804] -> w2793
              tunnel: w2795 -> [_ w2803]
              tunnel: [w2799 w2802] -> w2787
              tunnel: w2789 -> [w2799 w2801]
              frame False {
              }
              frame True {
                n1146 = Variant To Data(error in=w2805, type=w2801, Variant=w2803) -> (data=w2802:T11, error out=w2804:errorcluster)
              }
            }
            n1147 = Bundle By Name(cluster=w2788, "FanMode"=w2787) -> (w2785:T7)
            n1148 = Equal?(x=FanMode."On" ("FanMode"), y=w2787) -> (x = y?=w2791:bool)
            n1149 = call-poly <vilib>:"DAQmx Write.vi"("task/channels in"=refnum<k21> "PrecorFanCtrl", "data"=w2791, "error in"=w2793) -> ("error out"=w2792:errorcluster)  [unwired: 10 in, 2 out]
          }
          frame "Update Fan Mode LED Array" {
            # "Set the Fan Mode LED Array"
            n1150 = Unbundle By Name(w2808) -> ("Ctrl Refs.Fan Mode LED Array"=w2807:refnum<vi>)
            n1151 = Not Equal?(x=variant, y=w2812) -> (x != y?=w2811:bool)
            n1152 = case shown="True" w2811 {
              tunnel: w2814 -> [w2817 w2822]
              tunnel: [w2817 w2821] -> w2810
              tunnel: w2812 -> [_ w2820]
              tunnel: [w2816 w2819] -> w2806
              tunnel: w2807 -> [w2816 w2818]
              frame False {
              }
              frame True {
                n1153 = Variant To Data(error in=w2822, type=w2818, Variant=w2820) -> (data=w2819:refnum<vi>, error out=w2821:errorcluster)
              }
            }
            n1154 = Bundle By Name(cluster=w2808, "Ctrl Refs.Fan Mode LED Array"=w2806) -> (w2809:T7)
          }
          frame "update Thermal Equilibrium" {
            # "Set the Thermal Equilibrium"
            n1155 = Unbundle By Name(w2825) -> ("Thermal\nEquilibrium"=w2824:bool)
            n1156 = Not Equal?(x=variant, y=w2829) -> (x != y?=w2828:bool)
            n1157 = case shown="True" w2828 {
              tunnel: w2831 -> [w2834 w2839]
              tunnel: [w2834 w2838] -> w2827
              tunnel: w2829 -> [_ w2837]
              tunnel: [w2833 w2836] -> w2823
              tunnel: w2824 -> [w2833 w2835]
              frame False {
              }
              frame True {
                n1158 = Variant To Data(error in=w2839, type=w2835, Variant=w2837) -> (data=w2836:bool, error out=w2838:errorcluster)
              }
            }
            n1159 = Bundle By Name(cluster=w2825, "Thermal\nEquilibrium"=w2823) -> (w2826:T7)
          }
          frame "Sample Frequency" {
            # "Set the sample frequency"
            n1160 = Unbundle By Name(w2844) -> ("Sample Frequency"=w2843:dbl)
            n1161 = Not Equal?(x=variant, y=w2847) -> (x != y?=w2846:bool)
            n1162 = case shown="False" w2846 {
              tunnel: w2849 -> [w2852 w2857]
              tunnel: [w2852 w2856] -> w2845
              tunnel: w2847 -> [_ w2855]
              tunnel: [w2851 w2854] -> w2841
              tunnel: w2843 -> [w2851 w2853]
              frame False {
              }
              frame True {
                n1163 = Variant To Data(error in=w2857, type=w2853, Variant=w2855) -> (data=w2854:dbl, error out=w2856:errorcluster)
              }
            }
            n1164 = expression code="60/x"(w2841) -> (w2840:dbl)
            n1165 = Bundle By Name(cluster=w2844, "Sample Frequency"=w2840) -> (w2842:T7)
          }
          frame "set active channels" {
            # "Set the active channels in the system"
            n1166 = Unbundle By Name(w2865) -> ("Ctrl Refs.Data Display"=w2861:refnum<vi>, "Ctrl Refs.Data Setup"=w2864:refnum<vi>)
            n1167 = Not Equal?(x=variant, y=w2869) -> (x != y?=w2867:bool)
            n1168 = case shown="True" w2867 {
              tunnel: w2878 -> [w2881 w2898]
              tunnel: [w2880 w2897] -> w2863
              tunnel: [0 ("Column") w2893] -> w2877
              tunnel: w2864 -> [w2882 w2889]
              tunnel: [w2884 w2892] -> w2873
              tunnel: w2869 -> [_ w2891]
              tunnel: [w2883 w2890] -> w2866
              frame False {
                n1169 = property on="Property Node" class="MCListbox (strict)"(reference=w2882, error in=w2881) -> (reference out=w2884:refnum<vi>, error out=w2880:errorcluster, "ItemNames"=w2883:string[][])
              }
              frame True {
                n1170 = property on="Property Node" class="MCListbox (strict)"(reference=w2889) -> (reference out=w2888:refnum<vi>, error out=w2887:errorcluster, "ItemNames"=w2886:string[][])  [unwired: 1 in]
                n1171 = Variant To Data(error in=w2898, type=T17 {"ItemTag"="", "Row"=0, "Column"=0} ("output cluster"), Variant=w2891) -> (data=w2896:T17, error out=w2897:errorcluster)
                n1172 = Unbundle By Name(w2896) -> ("ItemTag"=w2895:string, "Row"=w2894:i32, "Column"=w2893:i32)
                n1173 = Replace Array Subset(array=w2886, new element=w2895, index (row)=w2894, index (col)=w2893) -> (w2890:string[][])
                n1174 = property on="Property Node" class="MCListbox (strict)"(reference=w2888, error in=w2887, "ItemNames"=w2890) -> (reference out=w2892:refnum<vi>)  [unwired: 1 out]
              }
            }
            n1175 = Index Array(array=w2866, index (col)=1 ("disabled index (col)")) -> (element=w2858:string[])  [unwired: 1 in]
            n1176 = call "Set Multicolumn Listbox Column Width.vi"("Number of Columns"=5, "Auto Columns"=TRUE, "Number of Rows"=u32 27, "error in (no error)"=w2863, "Multicolumn ListBox"=w2873) -> ("error out"=w2860:errorcluster)  [unwired: 5 in, 1 out]
            n1177 = Array Subset(array=w2858, index=15) -> (→"CH Name":string[])  [unwired: 1 in]
            n1178 = case shown="0" w2877 {
              tunnel: [w2907 w2917] -> w2879
              tunnel: w2865 -> [w2903 w2918]
              tunnel: w2866 -> [w2902 w2919]
              frame 0 {
                n1179 = Unbundle By Name(w2903) -> ("Channels"=w2904:string[])
                n1180 = Index Array(array=w2902, index (col)=0 ("disabled index (col)")) -> (element=w2901:string[])  [unwired: 1 in]
                n1181 = for {
                  tunnel: w2904 -> [w2912]
                  tunnel: w2901 -> [w2911] mode=indexing
                  shift-right: [w2909] -> w2900
                  shift-left: i32[] [] ("Inidicies") -> [w2908]
                  n1182 = Search 1D Array(1D array=w2912, element=w2911) -> (index of element=w2910:i32)  [unwired: 1 in]
                  n1183 = case shown="0, Default" w2910 {
                    selector: w2910 -> [w2913 _]
                    tunnel: [w2914 w2916] -> w2909
                    tunnel: w2908 -> [w2915 w2916]
                    frame 0, Default {
                      n1184 = Build Array (concatenate)(w2915, w2913) -> (w2914:i32[])
                    }
                    frame -1 {
                    }
                  }
                }
                n1185 = Bundle By Name(cluster=w2903, "Active Channels"=w2902, "Active Indicies"=w2900) -> (w2907:T7)
              }
              frame 1, Default {
                n1186 = Bundle By Name(cluster=w2918, "Active Channels"=w2919) -> (w2917:T7)
              }
            }
            n1187 = property class="Ring (strict)"(reference=w2861, error in=w2860, "Strings []"=w2858) -> (error out=w2859:errorcluster)  [unwired: 1 out]
          }
        }
      }
      frame Error {
        n1188 = Unbundle By Name(w2923) -> ("Queue List"=w2920:string[], "Queue Array"=w2921:T8, "Last State"=w2922:string)
        n1189 = call "Reentrant Send Error.vi"("Queue Names"=w2920, "error in (no error)"=w2925, "Last State"=w2922, "Queues"=w2921) -> ("error out"=w2924:errorcluster)  [unwired: 7 in]
      }
    }
  }
  n1190 = disable-structure shown="RUN_TIME_ENGINE==True" {
    disable-tunnel: w57 -> [_ _]
    disable-tunnel: w56 -> [_ _]
    disable-tunnel: w52 -> [_ _]
    frame condition #0 (active) {
    }
    frame condition #1 {
      n1191 = Quit LabVIEW(quit? (T)=TRUE) -> ()
    }
  }
  "Version" <- w21
